vi "MC_8_7_12a_JW.vi"() -> ()   [LabVIEW 2011]
uses:
  <vilib>/Utility/file.llb/Read From Spreadsheet File (string).vi
  <vilib>/Utility/inputDevices.llb/keyboardAcquire.vi
  <vilib>/Utility/file.llb/Write To Spreadsheet File (DBL).vi
  <vilib>/Utility/file.llb/Write To Spreadsheet File (string).vi
  <vilib>/regexp/Match Regular Expression.xnode
panel:
  out "Opj X Axis":string
  in  "Room Temp":dbl=294.0
  out "No Image 2":path=path "\\\\acad1\\physics/Jurchescu-group/JW-PD/Image Not Found.png"
  out "Save1 Array":string[][](array[string])
  out "Lin Vd":dbl
  out "Lin-Vg Array-Used":dbl[](array[numeric])
  out "Lin Id-Used":dbl[](array[numeric])
  out "Comments":string
  out "Folder Index":dbl caption="Length"
  out "Current \nRecord":string[](array[string])
  out "Transformer \nHeaders":string[](array[string])
  out "Current Device ID":string
  out "Column":string
  out "Row":string
  out "Rec: Concentration":dbl
  out "Rec: Solvent":string
  out "Rec: Method":string
  in  "?":T1(tab)
  in  "Transport File":path
  out "Transport Folder":path
  out "Rec: Material":string
  in  "Treatment Concentration (mM):":dbl=nan
  in  "Surface Treatment:":string="NaN"
  in  "# Drops*:":dbl=inf
  in  "Solution Temp (C):":dbl=nan
  in  "Relative Humidity (%):":dbl=nan
  in  "Room Temp (F):":dbl=nan
  in  "Time (s):":dbl=nan
  out "Accel (RPM/s):":dbl
  in  "RPM:":dbl=nan
  in  "Wait Time (s):":dbl=nan
  in  "Sample #:":dbl=1.0
  in  "Fabricator:":string="NaN"
  in  "Transfer File":path
  out "Transfer Folder":path
  in  "Image Folder":path
  out "Image File":path=path "D:/UserData/Desktop/Jeremy/WFU/Research/Programs/VI mods/Image Not Found.png"
  in  "Ramp (s):":dbl=3.0
  out "Calc: On/Off":dbl caption="On/Off-Sat" format="%#.2e"
  out "Calc: Off I-Sat":dbl caption="Off I-Sat" format="%#.2e"
  in  "Manuel-Dielectric":bool
  in  "Manuel-Length":bool
  out "Calc: VT-Lin":dbl
  out "New: VT-Lin":dbl
  out "Rec: VT-Lin":dbl caption="VT-Lin" format="%#_3g"
  out "Calc: Trap Density-STS":dbl format="%#.2e"
  out "New: Trap Density-STS":dbl format="%#.2e"
  out "Rec: Trap Density-STS":dbl caption="N-Sat (STS)" format="%#.2e"
  out "Calc: Trap Density-VT":dbl format="%#.2e"
  out "New: Trap Density-VT":dbl format="%#.2e"
  out "Rec: Trap Density-VT":dbl caption="N-Sat (VT)" format="%#.2e"
  out "Calc: Mobility-Lin":dbl format="%#.2e"
  out "New: Mobility-Lin":dbl format="%#_4e"
  out "Rec: Mobility-Lin":dbl caption="Mobility-Lin" format="%#_3e"
  out "Calc: Mobility-Sat":dbl format="%#.2e"
  out "Rec: Length":dbl caption="Length" format="%#_3g"
  out "Rec: Width":dbl caption="Width" format="%#_4g"
  out "Rec: Dielectric (d)":dbl caption="Dielectric (d)" format="%#_3g"
  in  "Cancel Button":bool
  in  "Up Button":bool
  in  "Down Button":bool
  out "Data Name:":string
  in  "Save Changes?":bool
  in  "New: Dielectric":dbl
  in  "New: Length":dbl
  in  "New: Width":dbl
  out "New: Mobility-Sat":dbl format="%#.2e"
  in  "Blank Button":bool
  in  "Zoom":i16(slide)=-3 scale=-5.0..5.0
  out "Image Out 2":T2(plugin-control)
  out "Image Out":T2(plugin-control)
  in  "Magnification":u16(ring) items=["5x", "10x", "20x", "50x", "80x"]
  out "Total Width":dbl
  out "Distances":dbl[](array[numeric])
  in  "Undo Button":bool
  in  "Remove Button":bool
  out "Rec: Mobility-Sat":dbl caption="Mobility-Sat" format="%#.2e"
  out "Index":string
  out "Image Name":string
  in  "Export":bool
  out "Calc: VT-Sat":dbl format="%#.2g"
  out "New: VT-Sat":dbl format="%#.2g"
  in  "Manual-Width":bool caption="Manual"
  out "Calc: STS":dbl format="%#.2g"
  out "New: STS":dbl format="%#.2g"
  out "Rec: VT-Sat":dbl caption="VT-Sat" format="%#.2g"
  out "Rec: STS":dbl caption="STS-Sat" format="%#.2g"
  out "Rec: On/Off":dbl caption="On/Off-Sat" format="%#.2e"
  in  "Save Changes? 2":bool
  in  "Save Changes? 3":bool
  out "Date Recorded":string="Date Recorded" caption="Measured"
  out "Date Created":string caption="Fabricated"
  out "Rec: Temp":dbl caption="Sample Temp" format="%.1f"
  in  "New: Temp":dbl format="%.1f"
  out "Rec: Off I-Sat":dbl caption="Off I-Sat" format="%#.2e"
  in  "Independant Variable":string(combo)="Length (um):"
  in  "Transfer Plots":enum32{"Linear", "Saturation"}(tab)=enum."Saturation"
  out "XY Graph-Lin":cluster{dbl[], dbl[]}[](graph)
  in  "Slide":dbl(slide) step=1.0 scale=-22.0..89.0 scale format="%#_1p"
  out "XY Graph":cluster{dbl[], dbl[]}[](graph)
  in  "Previous Button":bool
  in  "Next Button":bool
  in  "NumPts":dbl=5.0
  in  "Log Plots":enum32{"Linear", "Saturation"}(tab)=enum."Saturation"
  in  "Slide 2":dbl(slide) step=1.0 scale=-1.0..82.0 scale format="%#_1p"
  out "XY Graph 2":cluster{dbl[], dbl[]}[](graph)
  in  "Previous Button 2":bool
  in  "Next Button 2":bool
  in  "NumPts 2":dbl=5.0 caption="NumPts"
  in  "Manual-Temp":bool caption="Manual"
  in  "Origin Project File":path=path "\\\\acad1\\physics/Jurchescu-group/JW-PD/Group Library/Origin Project Files/DeviceData_7_31_12b_JW.opj"
  in  "No Image File":path=path "\\\\acad1\\physics/Jurchescu-group/JW-PD/Mega Awesome/Image Not Found.png"
  out "String":string
  out "Index 2":dbl
  out "Sat Id-Log-Used":dbl[](array[numeric])
  out "Vg Array-Log-Used":dbl[](array[numeric])
  out "ROI Descriptor out":T3 {"Contours"."Type" items=["No Selection", "Point", "Line", "Rectangle", "Oval", "Polygon", "Freehand Region", "Annulus", "Unused2", "Unused3", "Broken Line", "Freehand Line", "Rotated Rectangle"]}
  out "ROI Descriptor":T3 {"Contours"."Type" items=["No Selection", "Point", "Line", "Rectangle", "Oval", "Polygon", "Freehand Region", "Annulus", "Unused2", "Unused3", "Broken Line", "Freehand Line", "Rotated Rectangle"]}
  out "Numeric 3":dbl
  out "Array 6":dbl[][](array[numeric])
  out "Cluster":T4
  out "Array 5":dbl[](array[numeric])
  out "Array 4":dbl[](array[numeric])
  out "Array 3":dbl[](array[numeric])
  out "Numeric 2":dbl
  out "Numeric":dbl
  out "Sat Id-Used":dbl[](array[numeric])
  out "Sat Vg Array-Used":dbl[](array[numeric])
  out "MobVi Index":dbl
  in  "Row Start":dbl=20.0
  # "Data Locations"
  # "Transport Location"
  # "Transfer Location"
  # "Image Location"
  # "Sample Properties"
  # "*     Inf = Full coverage\n   NaN = Unknown or Not Applicable"
  # "Recorded"
  # "Calculated"
  # "Re-Calculated"
  # "Manual"
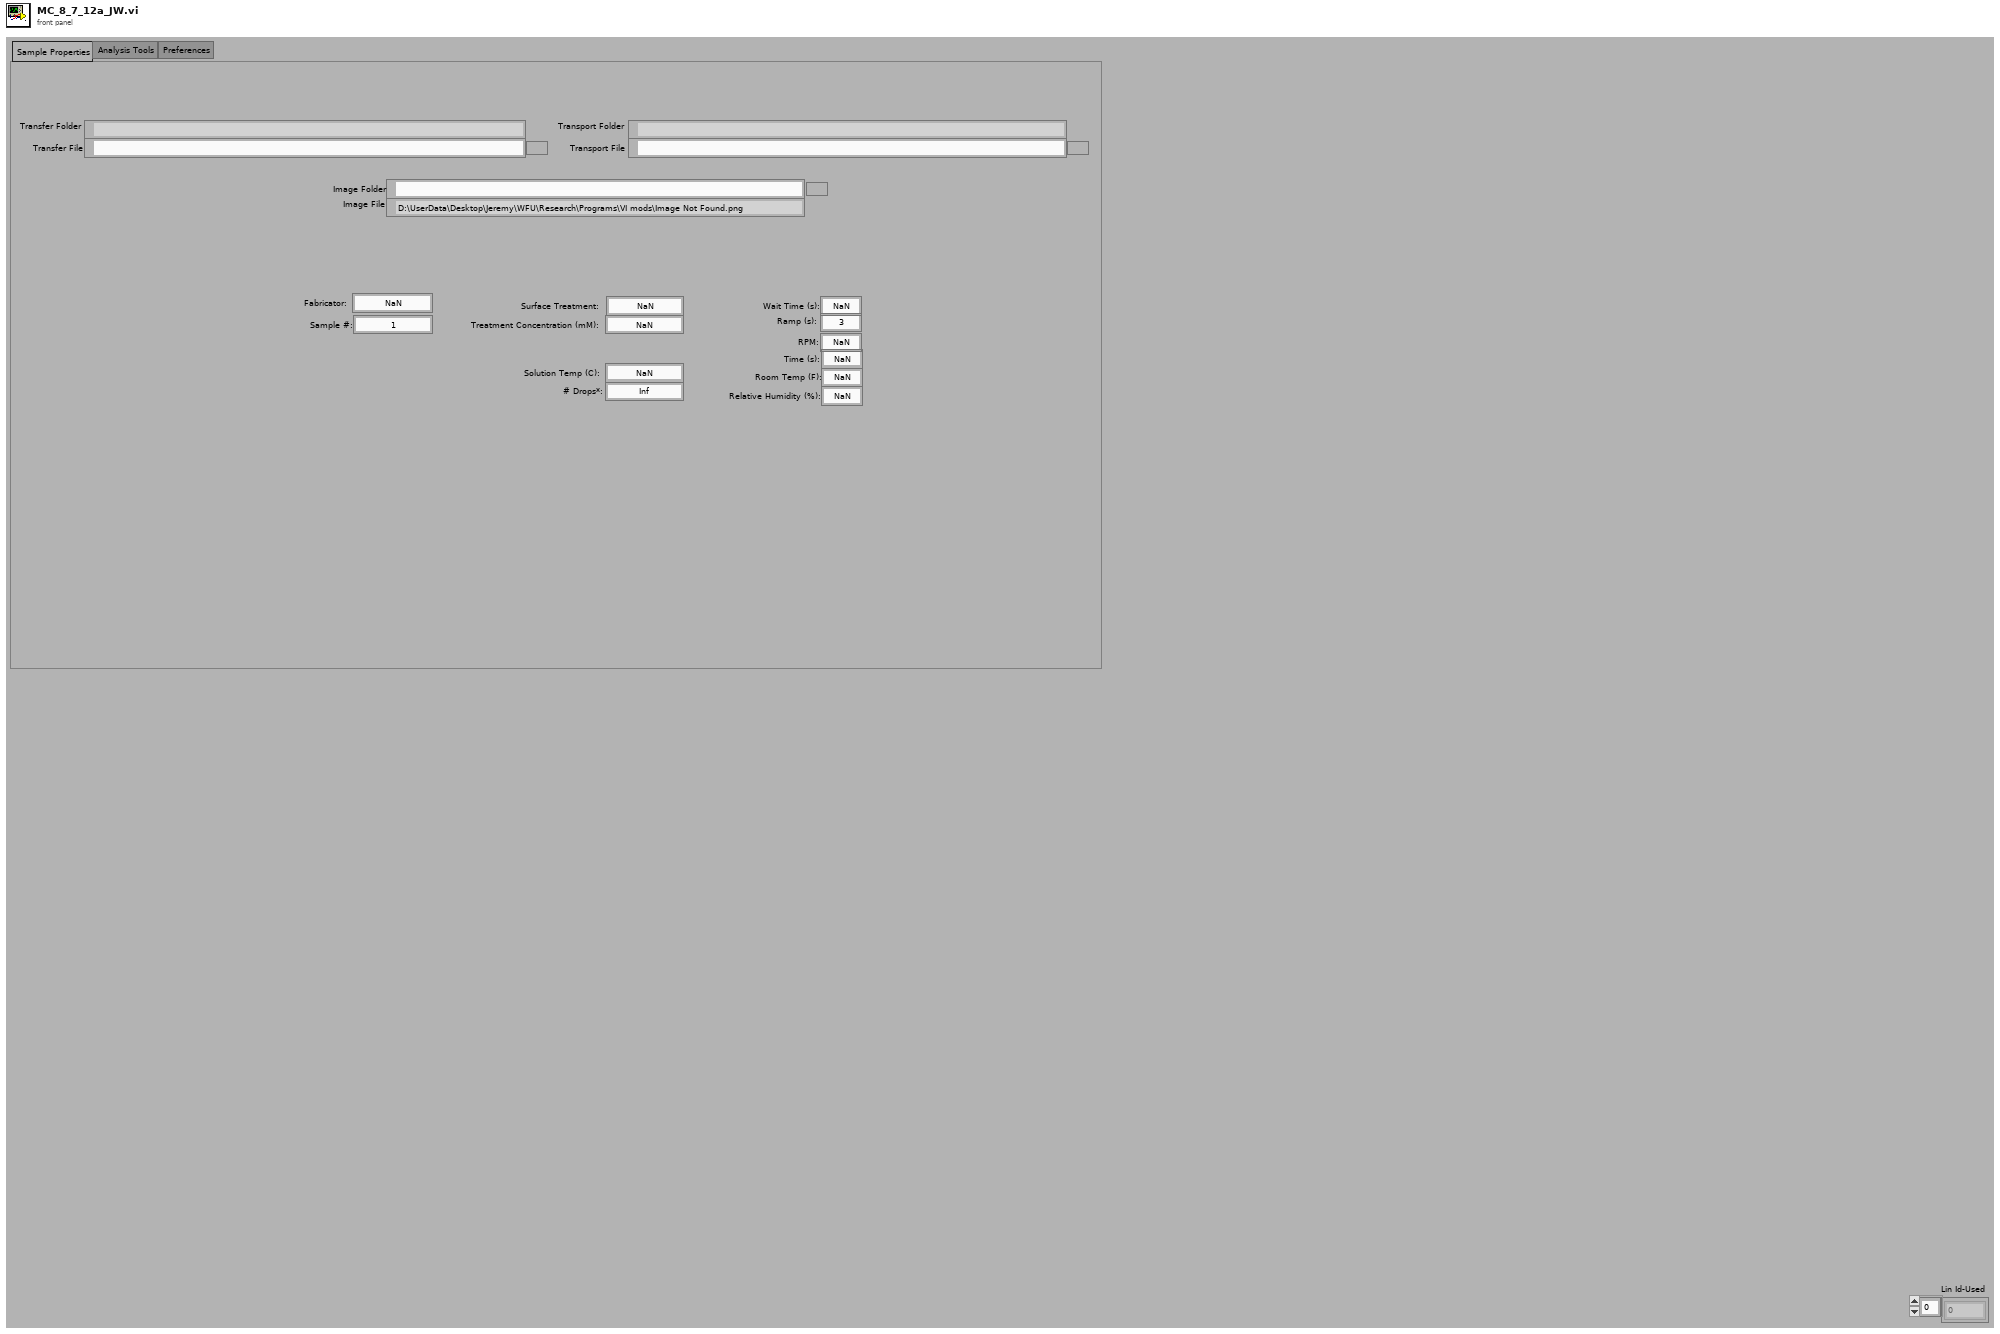
[diagram p1: front panel]
types:
  T1 = enum32{"Sample Properties", "Analysis Tools", "Preferences", "Current Database"}
  T2 = typedef "IMAQ Image.ctl" = refnum<image>
  T3 = typedef "ROI Descriptor" = cluster{"Global Rectangle":i32[], "Contours":cluster{"ID":enum32{"External", "Internal"}, "Type":u32, "Coordinates":i32[]}[]}
  T4 = cluster{"Numeric":dbl, "Numeric 2":dbl, "Numeric 3":dbl, "Numeric 4":dbl}
  T5 = cluster{"Mobility-Sat":dbl, "Moblitity-Lin":dbl, "On/Off":dbl, "Off Current":dbl, "Vt-Sat":dbl, "STS":dbl, "Trap Density-VT":dbl, "Trap Density-STS":dbl}
  T6 = cluster{"Date Recorded":string, "Index":string, "Length":dbl, "Width":dbl, "Sample Temp":dbl}
  T7 = cluster{"Date Created":string, "Material":string, "Solvent":string, "Concentration":dbl, "Method":string, "Dielectric (nm)":dbl, "Treatment":string, "Comments":string}
  T8 = cluster{"Mobility-Sat":dbl, "Vt-Sat":dbl, "Mobility-Lin":dbl, "Vt-Lin":dbl, "Off I-Sat":dbl, "On/Off I-Sat":dbl}
  T9 = cluster{"[0]":cluster{dbl[], dbl[]}, "[1]":cluster{dbl[], dbl[]}, "[2]":cluster{dbl[], dbl[]}, "[3]":cluster{dbl[], dbl[]}, "[4]":cluster{dbl[], dbl[]}, "[5]":cluster{dbl[], dbl[]}, "[6]":cluster{dbl[], dbl[]}, "[7]":cluster{dbl[], dbl[]}, "[8]":cluster{dbl[], dbl[]}}
  T10 = cluster{"Global Rectangle":i32[], "Contours":cluster{"Contour Type":u32, "ROI Type":u32, "Points":i32[]}[]}
  T11 = typedef "LVBoundsTypeDef.ctl" = cluster{"Width":u32, "Height":u32}
  T12 = enum16{"0", "1", "2", "3", "4", "5", "6", "7", "8", "9", "A", "B", "C", "D", "E", "F", "G", "H", "I", "J", "K", "L", "M", "N", "O", "P", "Q", "R", "S", "T", "U", "V", "W", "X", "Y", "Z", "F1", "F2", "F3", "F4", "F5", "F6", "F7", "F8", "F9", "F10", "F11", "F12", "F13", "F14", "F15", "ADD", "BACK", "BACKSLASH", "CAPITAL", "COMMA", "DECIMAL", "DELETE", "DIVIDE", "DOWN", "END", "EQUALS", "ESCAPE", "GRAVE (`)", "HOME", "INSERT", "LBRACKET", "LCONTROL", "LEFT", "L ALT", "LSHIFT", "LWIN", "MINUS", "MULTIPLY", "NEXT", "NUMLOCK", "NUMPAD_0", "NUMPAD_1", "NUMPAD_2", "NUMPAD_3", "NUMPAD_4", "NUMPAD_5", "NUMPAD_6", "NUMPAD_7", "NUMPAD_8", "NUMPAD_9", "PAUSE", "PERIOD", "PRIOR (PG UP)", "RBRACKET", "RCONTROL", "RETURN", "RIGHT", "R ALT", "RSHIFT", "RWIN", "SCROLL", "SEMICOLON", "SLASH", "SPACE", "SUBTRACT", "TAB", "UP", "ENTER (num pad)", "' (quote)"}[]
  T13 = enum16{"0", "1", "2", "3", "4", "5", "6", "7", "8", "9", "A", "B", "C", "D", "E", "F", "G", "H", "I", "J", "K", "L", "M", "N", "O", "P", "Q", "R", "S", "T", "U", "V", "W", "X", "Y", "Z", "F1", "F2", "F3", "F4", "F5", "F6", "F7", "F8", "F9", "F10", "F11", "F12", "F13", "F14", "F15", "ADD", "BACK", "BACKSLASH", "CAPITAL", "COMMA", "DECIMAL", "DELETE", "DIVIDE", "DOWN", "END", "EQUALS", "ESCAPE", "GRAVE (`)", "HOME", "INSERT", "LBRACKET", "LCONTROL", "LEFT", "L ALT", "LSHIFT", "LWIN", "MINUS", "MULTIPLY", "NEXT", "NUMLOCK", "NUMPAD_0", "NUMPAD_1", "NUMPAD_2", "NUMPAD_3", "NUMPAD_4", "NUMPAD_5", "NUMPAD_6", "NUMPAD_7", "NUMPAD_8", "NUMPAD_9", "PAUSE", "PERIOD", "PRIOR (PG UP)", "RBRACKET", "RCONTROL", "RETURN", "RIGHT", "R ALT", "RSHIFT", "RWIN", "SCROLL", "SEMICOLON", "SLASH", "SPACE", "SUBTRACT", "TAB", "UP", "ENTER (num pad)", "' (quote)"}
  T14 = cluster{"Contour Type":u32, "ROI Type":u32, "Points":i32[]}[]
  T15 = cluster{i32[], cluster{"Contour Type":u32, "ROI Type":u32, "Points":i32[]}[]}
  T16 = cluster{"Independant  Variable Indicator":string, "Parameter String Indicator":string}
  T17 = cluster{string, sgl, bool, bool, bool, bool, bool, bool, i32}
  T18 = cluster{i32, cluster{string, sgl, bool, bool, bool, bool, bool, bool, i32}, i32, i32}
  T19 = cluster{"Contour Type":u32, "ROI Type":u32, "Points":i32[]}
  T20 = cluster{"Points[0]":i32, "Points[1]":i32, "Points[2]":i32, "Points[3]":i32, "Points[4]":i32, "Points[5]":i32, "Points[6]":i32, "Points[7]":i32, "Points[8]":i32}
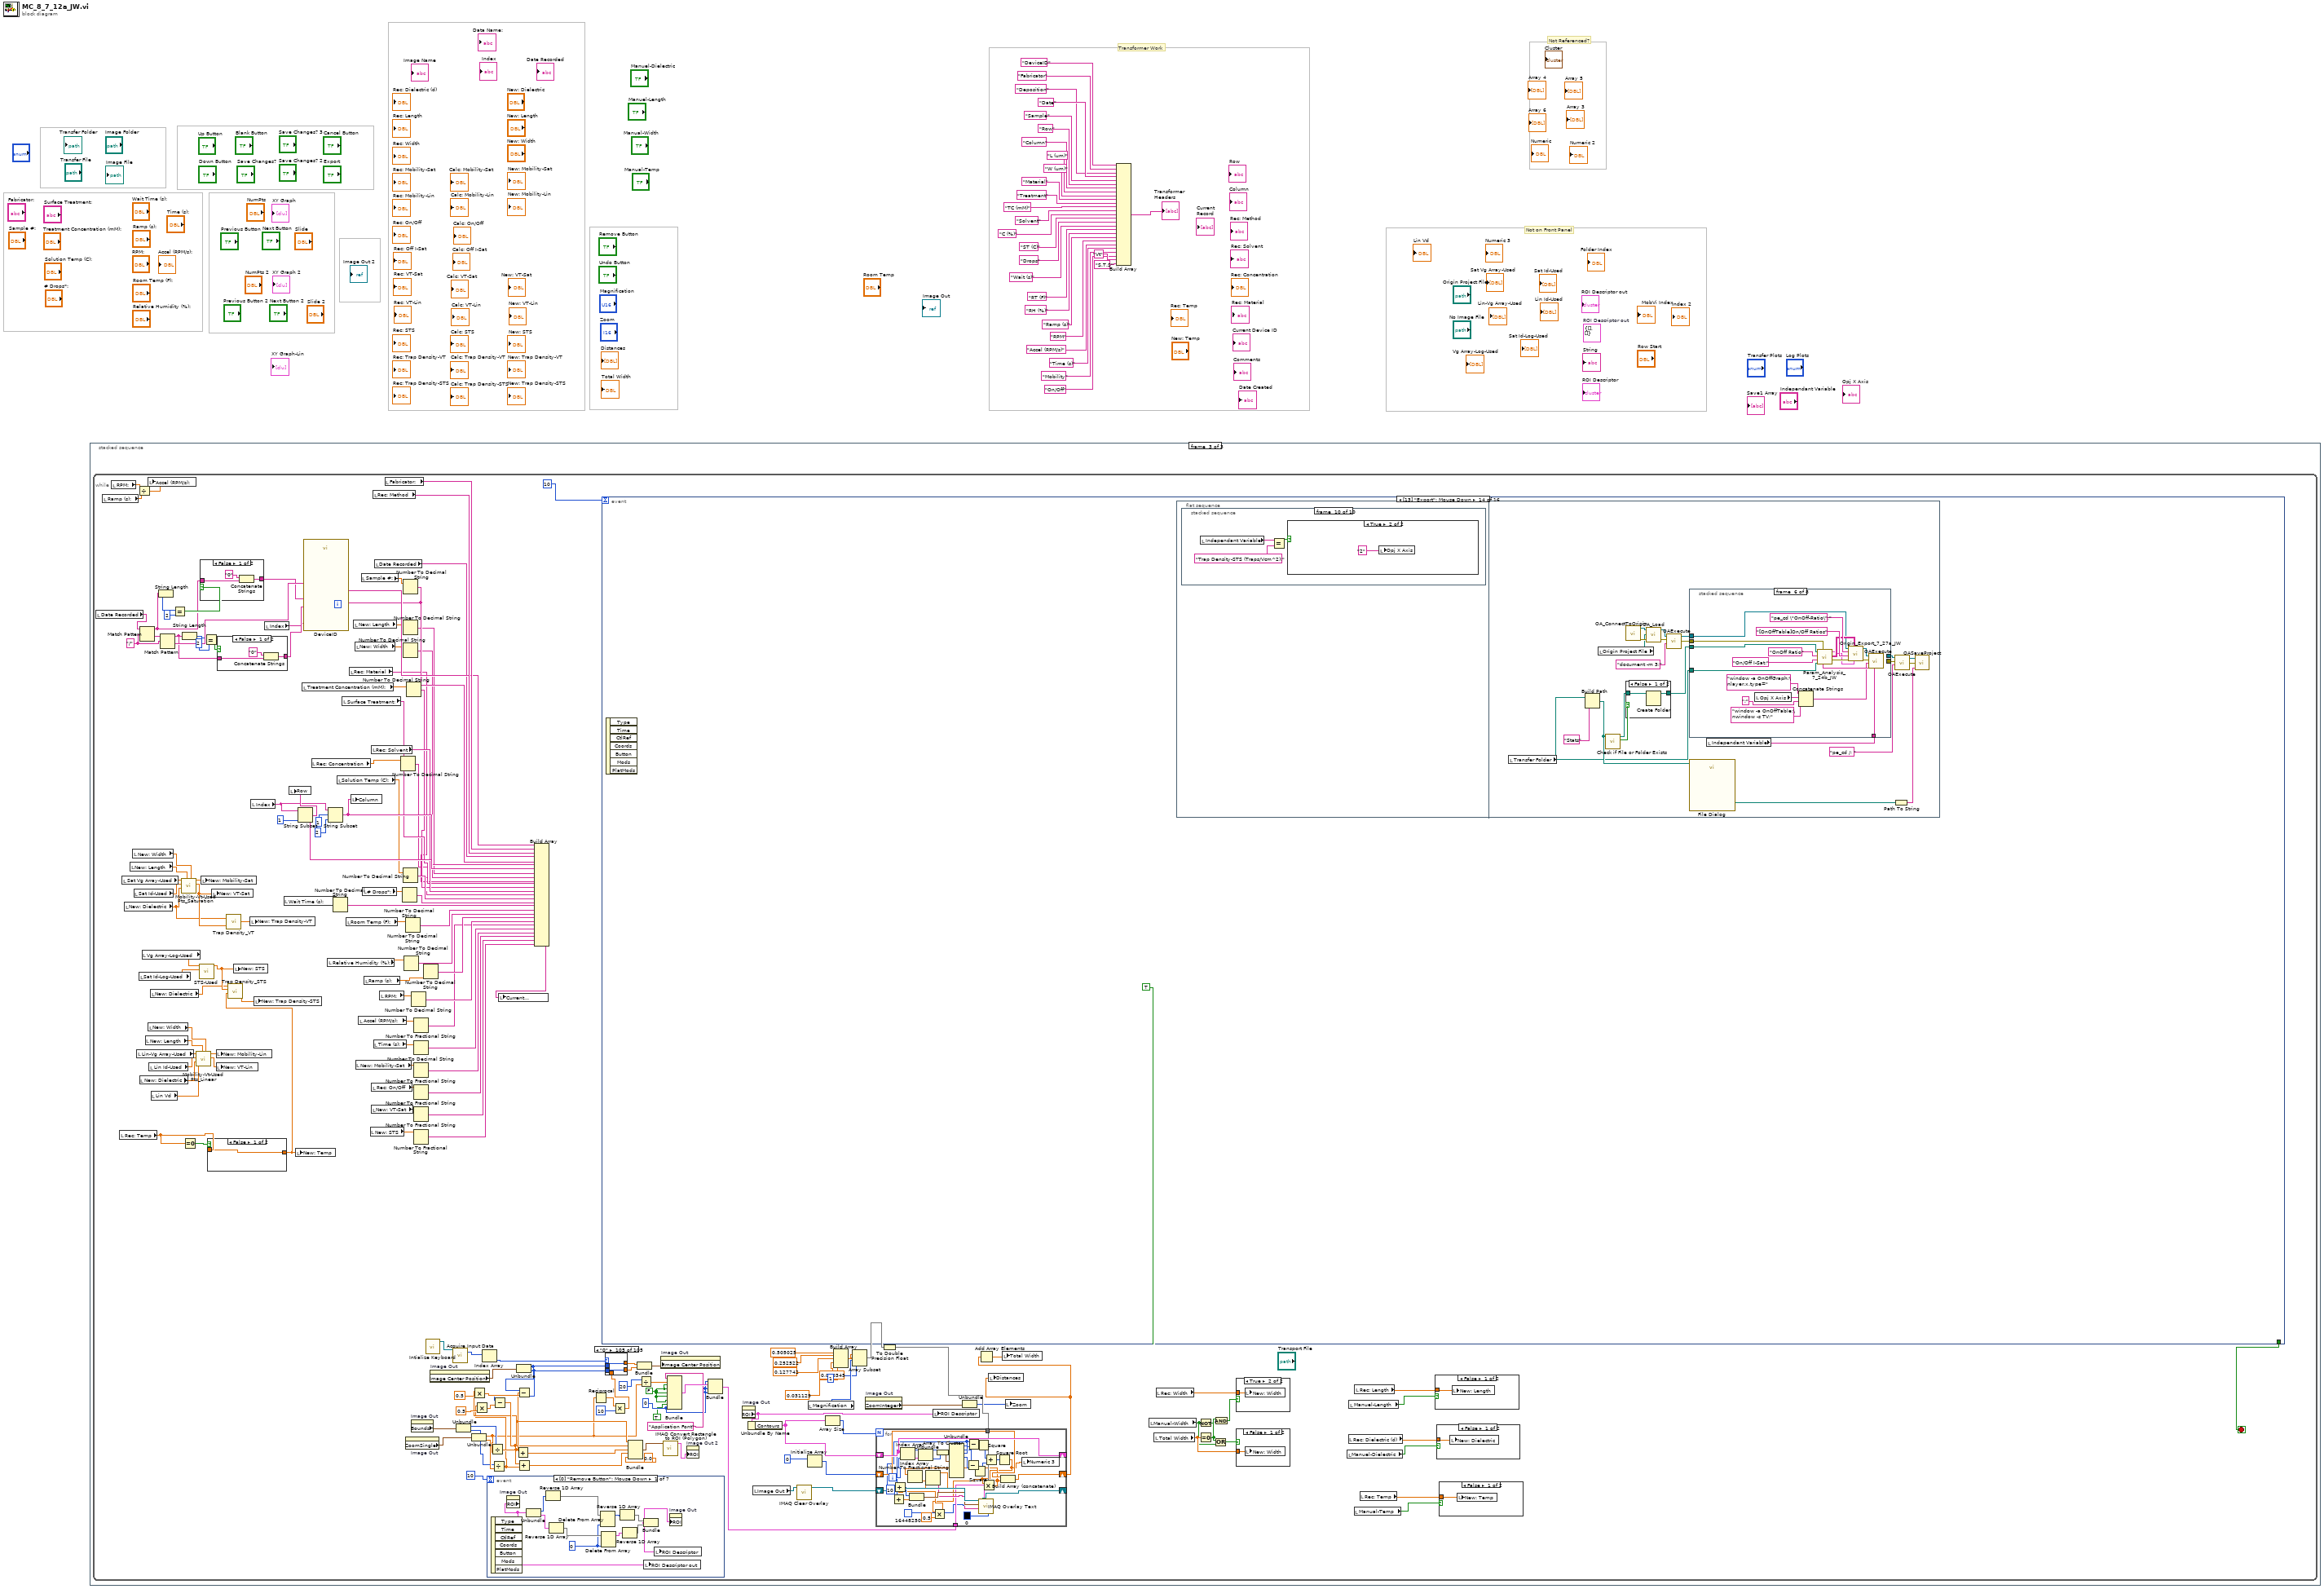
[diagram p0: block diagram]
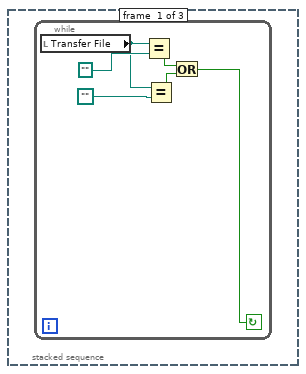
[diagram p2: hidden frame]
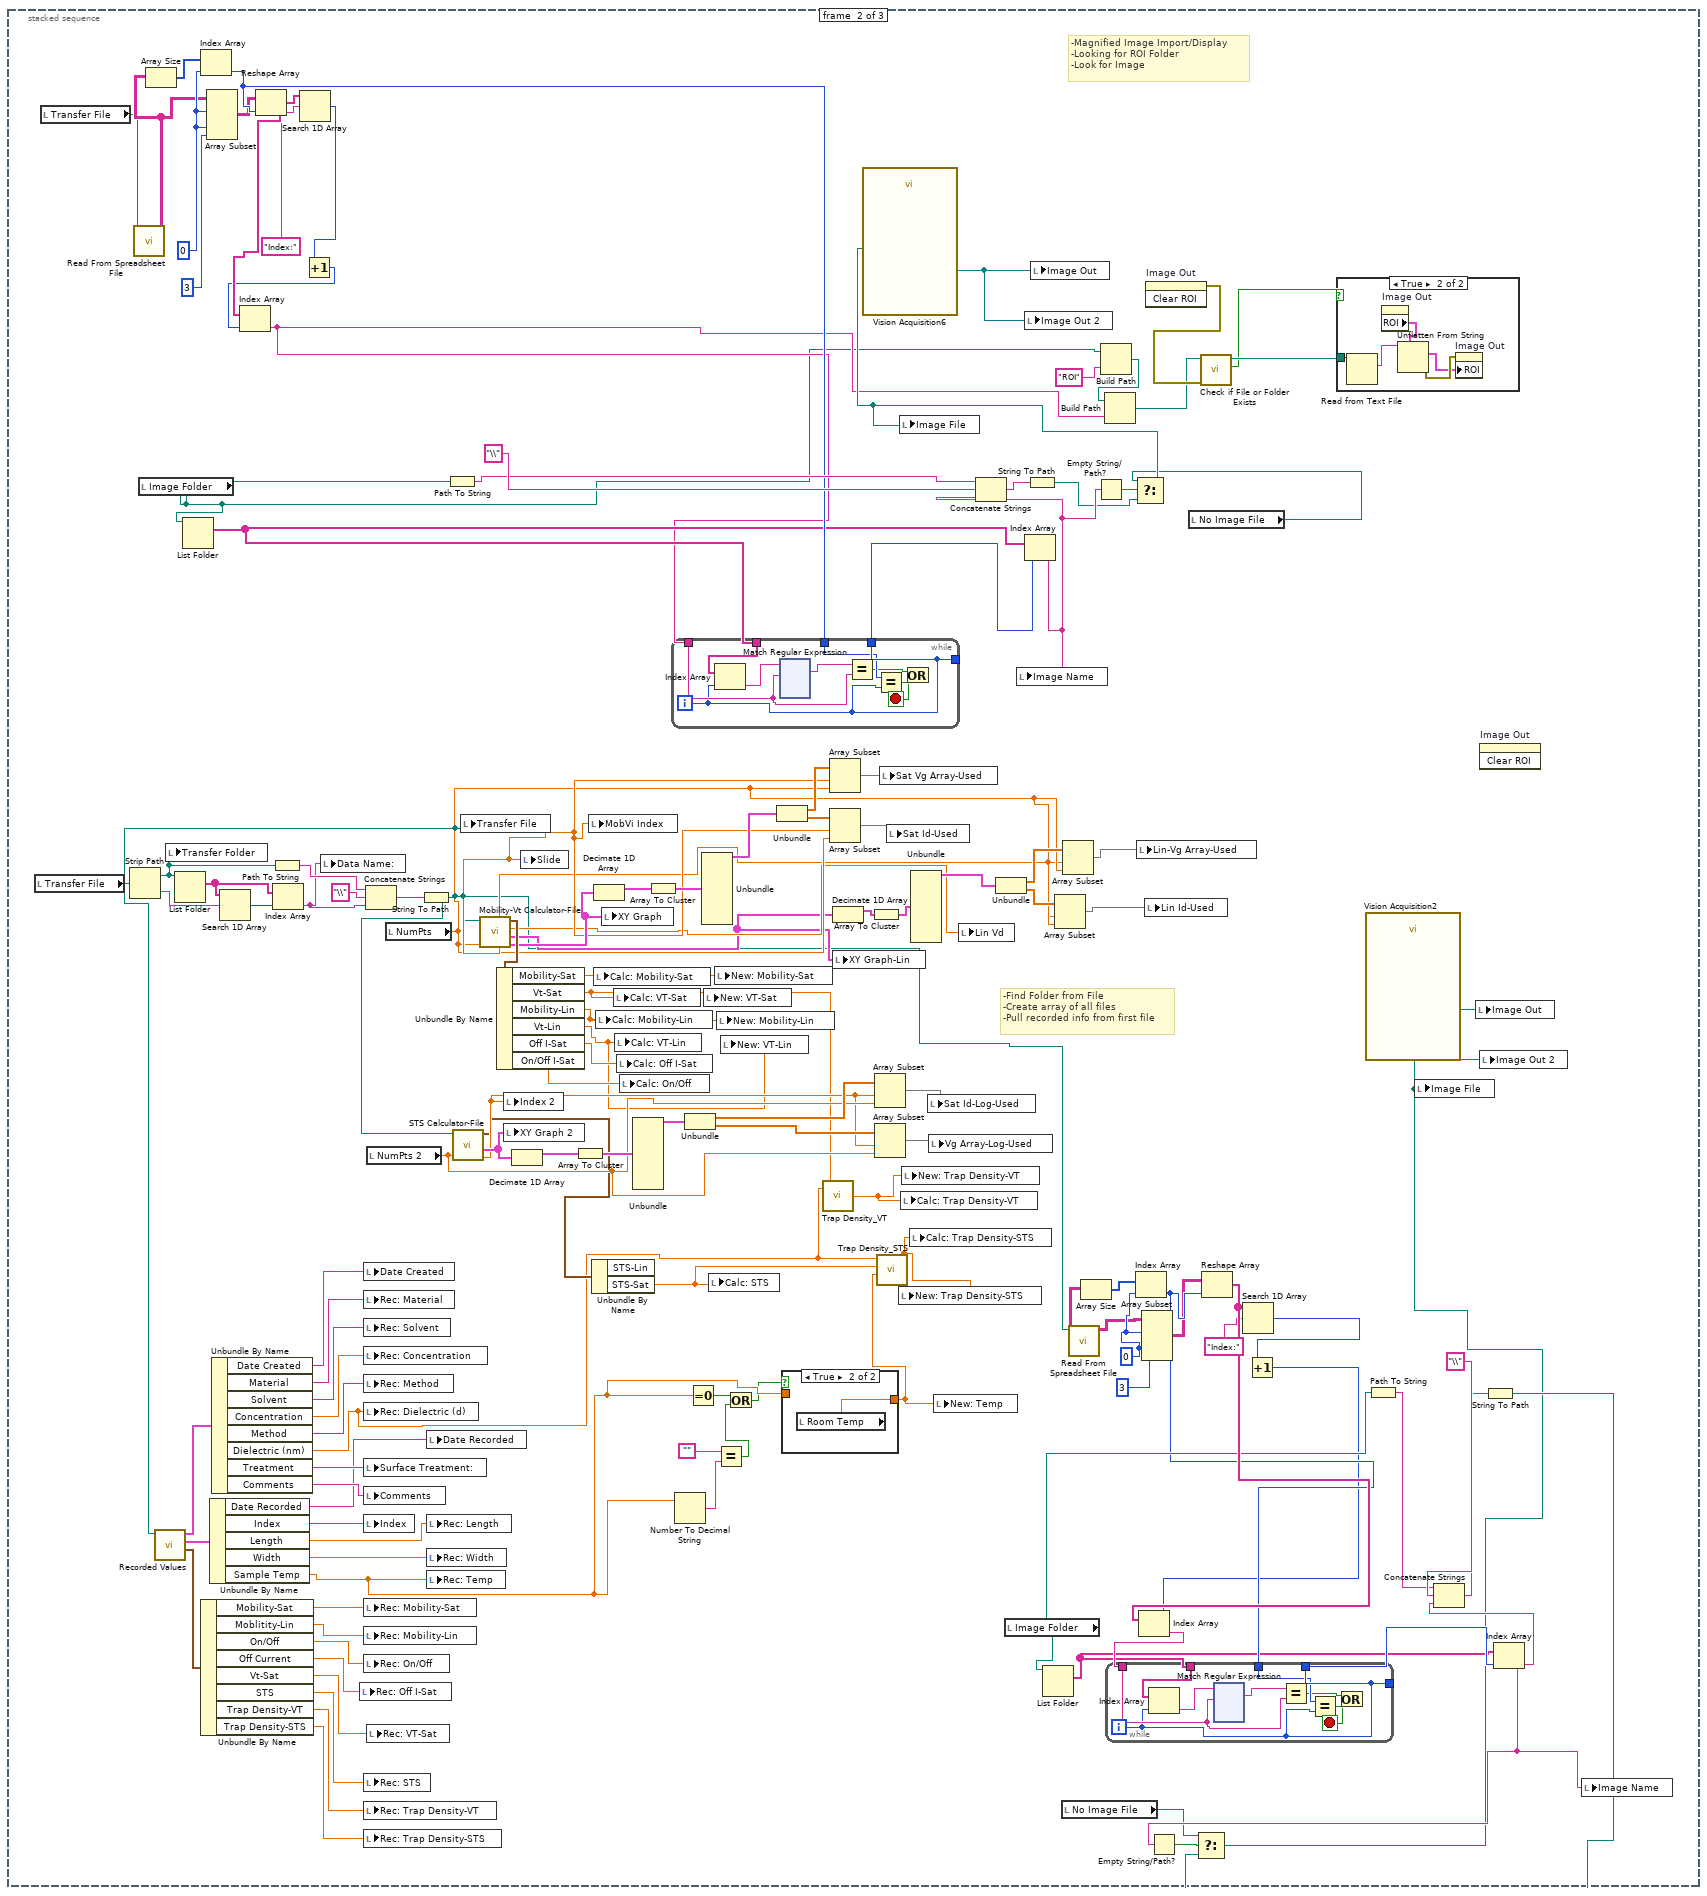
[diagram p3: hidden frame]
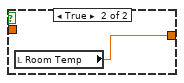
[diagram p7: hidden frame]
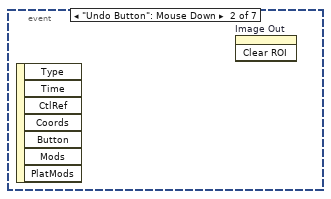
[diagram p14: hidden frame]
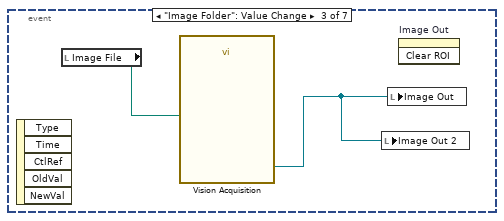
[diagram p15: hidden frame]
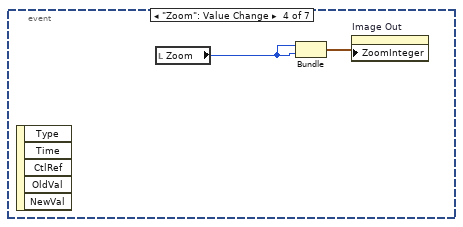
[diagram p16: hidden frame]
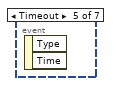
[diagram p17: hidden frame]
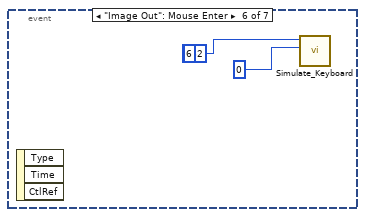
[diagram p18: hidden frame]
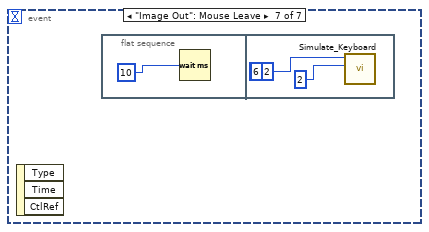
[diagram p19: hidden frame]
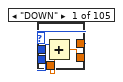
[diagram p20: hidden frame]
diagram:
  (unwired) T3 {"Global Rectangle"=[], "Contours"=[]}  # ROI Descriptor out
  # "Not Referenced?"
  # "Transformer Work"
  # "Not on Front Panel"
  n1 = stacked-sequence {
    frame #0 {
      n2 = while {
        stop <- w29 continue-if-true
        n3 = local read "Transfer File"() -> (w31:path)
        n4 = Equal?(x=w31, y=path "") -> (x = y?=w33:bool)
        n5 = Equal?(x=w31, y=path "") -> (x = y?=w32:bool)
        n6 = Or(x=w33, y=w32) -> (x .or. y?=w29:bool)
      }
    }
    frame #1 {
      w133 = 0
      w157 = 0
      # "-Find Folder from File\n-Create array of all files\n-Pull recorded info from first file"
      # "-Magnified Image Import/Display\n-Looking for ROI Folder\n-Look for Image"
      n7 = local read "Transfer File"() -> (w137:path)
      n8 = local read "Transfer File"() -> (w152:path)
      n9 = Strip Path(path=w137) -> (stripped path=w138:path, name=w124:string)
      n10 = call-poly <vilib>:"Read From Spreadsheet File.vi"("file path (dialog if empty)"=w152) -> ("all rows"=w155:string[][])  [unwired: 6 in, 4 out]
      n11 = local read "Image Folder"() -> (w94:path)
      n12 = Array Size(array=w155) -> (size(s)=w156:i32[])
      n13 = local write "Transfer Folder"(w138) -> ()
      n14 = List Folder(path=w138) -> (filenames=w128:string[])  [unwired: 3 in, 3 out]
      n15 = List Folder(path=w94) -> (filenames=w161:string[])  [unwired: 3 in, 3 out]
      n16 = Index Array(array=w156, index=w157) -> (element=w163:i32)
      n17 = Array Subset(array=w155, index (row)=w157, index (col)=w157, length (col)=3) -> (w154:string[][])  [unwired: 1 in]
      n18 = Search 1D Array(1D array=w128, element=w124) -> (index of element=w127:i32)  [unwired: 1 in]
      n19 = Reshape Array(w154, w163) -> (w168:string[])
      n20 = Path To String(path=w138) -> (string=w123:string)
      n21 = Index Array(array=w128, index=w127) -> (element=w93:string)
      n22 = Search 1D Array(1D array=w168, element="Index:") -> (index of element=w160:i32)  [unwired: 1 in]
      n23 = Increment(x=w160) -> (x+1=w159:i32)
      n24 = Index Array(array=w168, index=w159) -> (element=w95:string)
      n25 = local write "Data Name:"(w93) -> ()
      n26 = Concatenate Strings(w123, "\\", w93) -> (w125:string)
      n27 = local read "NumPts 2"() -> (w68:dbl)
      n28 = local read "NumPts"() -> (w59:dbl)
      n29 = String To Path(string=w125) -> (path=w52:path)
      n30 = call "Recorded Values.vi"("Path"=w52) -> ("Recorded Char"=w91:T5, "Recorded Prop"=w90:T6, "Fabrication Prop"=w92:T7)  [unwired: 8 in]
      n31 = Unbundle By Name(w91) -> ("Mobility-Sat"=w79:dbl, "Moblitity-Lin"=w78:dbl, "On/Off"=w77:dbl, "Off Current"=w76:dbl, "Vt-Sat"=w38:dbl, "STS"=w75:dbl, "Trap Density-VT"=w74:dbl, "Trap Density-STS"=w73:dbl)
      n32 = Unbundle By Name(w90) -> ("Date Recorded"=w83:string, "Index"=w82:string, "Length"=w81:dbl, "Width"=w80:dbl, "Sample Temp"=w44:dbl)
      n33 = Unbundle By Name(w92) -> ("Date Created"=w72:string, "Material"=w89:string, "Solvent"=w88:string, "Concentration"=w87:dbl, "Method"=w86:string, "Dielectric (nm)"=w48:dbl, "Treatment"=w85:string, "Comments"=w84:string)
      n34 = local write "Rec: Off I-Sat"(w76) -> ()
      n35 = local write "Date Created"(w72) -> ()
      n36 = local write "Rec: Material"(w89) -> ()
      n37 = local write "Rec: Solvent"(w88) -> ()
      n38 = local write "Rec: Concentration"(w87) -> ()
      n39 = local write "Rec: Method"(w86) -> ()
      n40 = local write "Rec: Dielectric (d)"(w48) -> ()
      n41 = local write "Surface Treatment:"(w85) -> ()
      n42 = local write "Comments"(w84) -> ()
      n43 = local write "Index"(w82) -> ()
      n44 = local write "Rec: Mobility-Sat"(w79) -> ()
      n45 = local write "Rec: Mobility-Lin"(w78) -> ()
      n46 = local write "Rec: On/Off"(w77) -> ()
      n47 = local write "Rec: STS"(w75) -> ()
      n48 = local write "Rec: Trap Density-VT"(w74) -> ()
      n49 = local write "Rec: Trap Density-STS"(w73) -> ()
      n50 = local write "Rec: VT-Sat"(w38) -> ()
      n51 = local write "Date Recorded"(w83) -> ()
      n52 = local write "Rec: Length"(w81) -> ()
      n53 = local write "Rec: Width"(w80) -> ()
      n54 = local write "Rec: Temp"(w44) -> ()
      n55 = Path To String(path=w94) -> (string=w165:string)
      n56 = call "STS Calculator-File.vi"("NumPts"=w68, "Path"=w52) -> ("STS Index-Sat"=w66:dbl, "XY Graph-Sat"=w67:cluster{dbl[], dbl[]}[], "Ouput"=w65:cluster{"STS-Sat":dbl, "STS-Lin":dbl})  [unwired: 5 in, 2 out]
      n57 = local write "Transfer File"(w52) -> ()
      n58 = call "Mobility-Vt Calculator-File.vi"("NumPts"=w59, "Path"=w52) -> ("XY Graph-Sat"=w70:cluster{dbl[], dbl[]}[], "XY Graph-Lin"=w54:cluster{dbl[], dbl[]}[], "Lin Vd"=w55:dbl, "Output"=w71:T8, "Index-Sat"=w69:dbl, "Index-Lin"=w58:dbl)  [unwired: 4 in]
      n59 = Unbundle By Name(w71) -> ("Mobility-Sat"=w47:dbl, "Vt-Sat"=w46:dbl, "Mobility-Lin"=w37:dbl, "Vt-Lin"=w35:dbl, "Off I-Sat"=w53:dbl, "On/Off I-Sat"=w36:dbl)
      n60 = local write "Index 2"(w66) -> ()
      n61 = local write "XY Graph 2"(w67) -> ()
      n62 = Decimate 1D Array(w67) -> (w115:cluster{dbl[], dbl[]}[])  [unwired: 1 out]
      n63 = local write "Slide"(w69) -> ()
      n64 = Array To Cluster(array=w115) -> (cluster=w117:T9)
      n65 = local write "MobVi Index"(w69) -> ()
      n66 = Unbundle By Name(w65) -> ("STS-Sat"=w51:dbl)  [unwired: 1 out]
      n67 = Decimate 1D Array(w70) -> (w151:cluster{dbl[], dbl[]}[])  [unwired: 1 out]
      n68 = local write "Calc: Mobility-Sat"(w47) -> ()
      n69 = local write "Calc: Mobility-Lin"(w37) -> ()
      n70 = local write "XY Graph"(w70) -> ()
      n71 = local write "Calc: VT-Sat"(w46) -> ()
      n72 = local write "Calc: VT-Lin"(w35) -> ()
      n73 = local write "Calc: Off I-Sat"(w53) -> ()
      n74 = local write "Calc: On/Off"(w36) -> ()
      n75 = Unbundle(w117) -> ("[0]"=w116:cluster{dbl[], dbl[]})  [unwired: 8 out]
      n76 = Array To Cluster(array=w151) -> (cluster=w149:T9)
      n77 = while {
        tunnel: w161 -> [w303]
        tunnel: w95 -> [w301]
        tunnel: [w300] -> _
        tunnel: [w300] -> w162
        tunnel: w163 -> [w299]
        i -> [w300]
        stop <- w296 stop-if-true
        n78 = Index Array(array=w303, index=w300) -> (element=w304:string)
        n79 = xnode "Match Regular Expression"("input string"=w304, "regular expression"=w301) -> ("whole match"=w302:string)  [unwired: 4 in, 4 out]
        n80 = Equal?(x=w302, y=w301) -> (x = y?=w298:bool)
        n81 = Equal?(x=w299, y=w300) -> (x = y?=w297:bool)
        n82 = Or(x=w298, y=w297) -> (x .or. y?=w296:bool)
      }
      n83 = Number To Decimal String(number=w44) -> (decimal integer string=w42:string)  [unwired: 1 in]
      n84 = Unbundle(w116) -> (w113:dbl[], w112:dbl[])
      n85 = Equal To 0?(x=w44) -> (x = 0?=w43:bool)
      n86 = Unbundle(w149) -> ("[0]"=w150:cluster{dbl[], dbl[]})  [unwired: 8 out]
      n87 = local write "New: VT-Sat"(w46) -> ()
      n88 = local write "Calc: STS"(w51) -> ()
      n89 = local write "New: Mobility-Sat"(w47) -> ()
      n90 = Equal?(x="", y=w42) -> (x = y?=w40:bool)
      n91 = local write "New: Mobility-Lin"(w37) -> ()
      n92 = local write "New: VT-Lin"(w35) -> ()
      n93 = Or(x=w43, y=w40) -> (x .or. y?=w39:bool)
      n94 = Unbundle(w150) -> (w114:dbl[], w118:dbl[])
      n95 = case shown="True" w39 {
        tunnel: [w169 w170] -> w50
        tunnel: w44 -> [w169 _]
        frame False {
        }
        frame True {
          n96 = local read "Room Temp"() -> (w170:dbl)
        }
      }
      n97 = call "Trap Density_VT.vi"("VT"=w46, "Dielectric"=w48) -> ("Trap Density-VT"=w45:dbl)
      n98 = Array Subset(array=w114, index=w69, length=w59) -> (w121:dbl[])
      n99 = Array Subset(array=w118, index=w69, length=w59) -> (w122:dbl[])
      n100 = Decimate 1D Array(w54) -> (w64:cluster{dbl[], dbl[]}[])  [unwired: 1 out]
      n101 = local write "XY Graph-Lin"(w54) -> ()
      n102 = Array To Cluster(array=w64) -> (cluster=w63:T9)
      n103 = Array Subset(array=w113, index=w66, length=w68) -> (w120:dbl[])
      n104 = Array Subset(array=w112, index=w66, length=w68) -> (w119:dbl[])
      n105 = call "Trap Density_STS.vi"("Temp (T) [K]"=w50, "S.T.S. (S)"=w51, "Dielectric"=w48) -> ("Trap Density (N)"=w49:dbl)  [unwired: 8 in]
      n106 = local write "Sat Vg Array-Used"(w121) -> ()
      n107 = local write "Sat Id-Used"(w122) -> ()
      n108 = local write "New: Trap Density-STS"(w49) -> ()
      n109 = local write "Calc: Trap Density-VT"(w45) -> ()
      n110 = local write "New: Trap Density-VT"(w45) -> ()
      n111 = local write "Calc: Trap Density-STS"(w49) -> ()
      n112 = Unbundle(w63) -> ("[0]"=w62:cluster{dbl[], dbl[]})  [unwired: 8 out]
      n113 = local write "Sat Id-Log-Used"(w120) -> ()
      n114 = local write "Vg Array-Log-Used"(w119) -> ()
      n115 = local write "New: Temp"(w50) -> ()
      n116 = local write "Lin Vd"(w55) -> ()
      n117 = Unbundle(w62) -> (w61:dbl[], w60:dbl[])
      n118 = local read "Image Folder"() -> (w144:path)
      n119 = Index Array(array=w161, index=w162) -> (element=w111:string)
      n120 = Concatenate Strings(w165, "\\", w111) -> (w166:string)
      n121 = local write "Image Name"(w111) -> ()
      n122 = String To Path(string=w166) -> (path=w109:path)
      n123 = List Folder(path=w144) -> (filenames=w140:string[])  [unwired: 3 in, 3 out]
      n124 = Array Subset(array=w60, index=w58, length=w59) -> (w56:dbl[])
      n125 = local read "No Image File"() -> (w103:path)
      n126 = Array Subset(array=w61, index=w58, length=w59) -> (w57:dbl[])
      n127 = call-poly <vilib>:"Read From Spreadsheet File.vi"("file path (dialog if empty)"=w52) -> ("all rows"=w131:string[][])  [unwired: 6 in, 4 out]
      n128 = Array Size(array=w131) -> (size(s)=w132:i32[])
      n129 = Empty String/Path?(string/path=w111) -> (empty?=w110:bool)
      n130 = Build Path(base path=w94, name or relative path="ROI") -> (appended path=w97:path)
      n131 = Build Path(base path=w97, name or relative path=w95) -> (appended path=w96:path)
      n132 = Index Array(array=w132, index=w133) -> (element=w143:i32)
      n133 = local write "Lin-Vg Array-Used"(w57) -> ()
      n134 = Array Subset(array=w131, index (row)=w133, index (col)=w133, length (col)=3) -> (w130:string[][])  [unwired: 1 in]
      n135 = local write "Lin Id-Used"(w56) -> ()
      n136 = invoke on="Image Out" class="ImageControl" method="Clear ROI"() -> (error out=w101:errorcluster)  [unwired: 3 in, 2 out]
      n137 = local read "No Image File"() -> (w102:path)
      n138 = Select(t=w102, s=w110, f=w109) -> (s? t:f=w108:path)
      n139 = call "Vision Acquisition6"("Image Path"=w108) -> ("Image Out"=w164:T2)  [unwired: 25 in, 1 out]
      n140 = local write "Image File"(w108) -> ()
      n141 = local write "Image Out 2"(w164) -> ()
      n142 = local write "Image Out"(w164) -> ()
      n143 = call <vilib>:"Check if File or Folder Exists.vi"("error in (no error)"=w101, "path"=w96) -> ("file or folder exists?"=w99:bool, "dup path"=w100:path)  [unwired: 7 in, 1 out]
      n144 = Reshape Array(w130, w143) -> (w148:string[])
      n145 = Search 1D Array(1D array=w148, element="Index:") -> (index of element=w136:i32)  [unwired: 1 in]
      n146 = Increment(x=w136) -> (x+1=w135:i32)
      n147 = Index Array(array=w148, index=w135) -> (element=w141:string)
      n148 = while {
        tunnel: w140 -> [w183]
        tunnel: w141 -> [w181]
        tunnel: [w180] -> _
        tunnel: [w180] -> w142
        tunnel: w143 -> [w179]
        i -> [w180]
        stop <- w176 stop-if-true
        n149 = Index Array(array=w183, index=w180) -> (element=w184:string)
        n150 = xnode "Match Regular Expression"("input string"=w184, "regular expression"=w181) -> ("whole match"=w182:string)  [unwired: 4 in, 4 out]
        n151 = Equal?(x=w182, y=w181) -> (x = y?=w178:bool)
        n152 = Equal?(x=w179, y=w180) -> (x = y?=w177:bool)
        n153 = Or(x=w178, y=w177) -> (x .or. y?=w176:bool)
      }
      n154 = case shown="True" w99 {
        tunnel: w100 -> [_ w171]
        frame False {
        }
        frame True {
          n155 = Read from Text File(file (use dialog)=w171) -> (text=w175:string)  [unwired: 3 in, 3 out]
          n156 = property on="Image Out" class="ImageControl"() -> ("ROI"=w172:T10)  [unwired: 2 in, 2 out]
          n157 = Unflatten From String(type=w172, binary string=w175) -> (value=w173:T10, error out=w174:errorcluster)  [unwired: 3 in, 1 out]
          n158 = property on="Image Out" class="ImageControl"(error in=w174, "ROI"=w173) -> ()  [unwired: 1 in, 2 out]
        }
      }
      n159 = Path To String(path=w144) -> (string=w145:string)
      n160 = invoke on="Image Out" class="ImageControl" method="Clear ROI"() -> ()  [unwired: 3 in, 3 out]
      n161 = Index Array(array=w140, index=w142) -> (element=w106:string)
      n162 = Empty String/Path?(string/path=w106) -> (empty?=w107:bool)
      n163 = Concatenate Strings(w145, "\\", w106) -> (w146:string)
      n164 = String To Path(string=w146) -> (path=w105:path)
      n165 = Select(t=w103, s=w107, f=w105) -> (s? t:f=w104:path)
      n166 = call "Vision Acquisition2"("Image Path"=w104) -> ("Image Out"=w139:T2)  [unwired: 25 in, 1 out]
      n167 = local write "Image File"(w104) -> ()
      n168 = local write "Image Out"(w139) -> ()
      n169 = local write "Image Out 2"(w139) -> ()
      n170 = local write "Image Name"(w106) -> ()
    }
    frame #2 {
      n171 = while {
        stop <- w583 stop-if-true
        w479 = "/"
        w533 = FALSE
        w531 = 0
        n172 = local read "Date Recorded"() -> (w482:string)
        n173 = local read "Ramp (s):"() -> (w449:dbl)
        n174 = local read "RPM:"() -> (w450:dbl)
        n175 = local read "Rec: Temp"() -> (w421:dbl)
        n176 = local read "Sat Vg Array-Used"() -> (w438:dbl[])
        n177 = local read "New: Dielectric"() -> (w423:dbl)
        n178 = local read "New: Length"() -> (w439:dbl)
        n179 = local read "New: Width"() -> (w441:dbl)
        n180 = local read "Sat Id-Used"() -> (w437:dbl[])
        n181 = local read "Lin-Vg Array-Used"() -> (w432:dbl[])
        n182 = Divide(x=w450, y=w449) -> (x/y=w448:dbl)
        n183 = local read "Sat Id-Log-Used"() -> (w436:dbl[])
        n184 = local read "New: Dielectric"() -> (w429:dbl)
        n185 = Match Pattern(string=w482, regular expression=w479) -> (before substring=w473:string, after substring=w480:string)  [unwired: 1 in, 2 out]
        n186 = local read "Vg Array-Log-Used"() -> (w435:dbl[])
        n187 = local read "New: Length"() -> (w431:dbl)
        n188 = local write "Accel (RPM/s):"(w448) -> ()
        n189 = local read "New: Width"() -> (w428:dbl)
        n190 = local read "Lin Id-Used"() -> (w433:dbl[])
        n191 = local read "New: Dielectric"() -> (w425:dbl)
        n192 = local read "Lin Vd"() -> (w427:dbl)
        n193 = String Length(string=w473) -> (length=w476:i32)
        n194 = Match Pattern(string=w480, regular expression=w479) -> (before substring=w467:string, after substring=w478:string)  [unwired: 1 in, 2 out]
        n195 = Equal?(x=w476, y=2) -> (x = y?=w474:bool)
        n196 = call "Mobility-Vt-Used Pts_Saturation.vi"("Width"=w441, "Length"=w439, "Dielectric (d)"=w423, "Sat Id Used"=w437, "Vg Used"=w438) -> ("Vt"=w424:dbl, "Mobility"=w440:dbl)  [unwired: 4 in, 1 out]
        n197 = String Length(string=w467) -> (length=w469:i32)
        n198 = Equal To 0?(x=w421) -> (x = 0?=w420:bool)
        n199 = call "Mobility-Vt-Used Pts_Linear.vi"("Width"=w428, "Length"=w431, "Vd"=w427, "Dielectric (d)"=w429, "Sat Id Used"=w433, "Vg Used"=w432) -> ("Vt"=w434:dbl, "Mobility"=w430:dbl)  [unwired: 3 in, 1 out]
        n200 = call "STS-Used.vi"("Id Used"=w436, "Vg-Used"=w435) -> ("STS"=w426:dbl)  [unwired: 9 in]
        n201 = case shown="False" w474 {
          tunnel: w473 -> [w594 w596]
          tunnel: [w593 w596] -> w472
          frame False {
            n202 = Concatenate Strings("0", w594) -> (w593:string)
          }
          frame True {
          }
        }
        n203 = local write "New: Mobility-Sat"(w440) -> ()
        n204 = Equal?(x=w469, y=2) -> (x = y?=w471:bool)
        n205 = case shown="False" w420 {
          tunnel: [w585 w586] -> w418
          tunnel: w421 -> [w585 _]
          frame False {
          }
          frame True {
            n206 = local read "Room Temp"() -> (w586:dbl)
          }
        }
        n207 = local write "New: VT-Sat"(w424) -> ()
        n208 = local write "New: Mobility-Lin"(w430) -> ()
        n209 = local write "New: VT-Lin"(w434) -> ()
        n210 = case shown="False" w471 {
          tunnel: w467 -> [w590 w592]
          tunnel: [w589 w592] -> w468
          frame False {
            n211 = Concatenate Strings("0", w590) -> (w589:string)
          }
          frame True {
          }
        }
        n212 = call "Trap Density_VT.vi"("VT"=w424, "Dielectric"=w423) -> ("Trap Density-VT"=w422:dbl)
        n213 = call "Trap Density_STS.vi"("Temp (T) [K]"=w418, "S.T.S. (S)"=w426, "Dielectric"=w425) -> ("Trap Density (N)"=w419:dbl)  [unwired: 8 in]
        n214 = local write "New: STS"(w426) -> ()
        n215 = local write "New: Trap Density-VT"(w422) -> ()
        n216 = local read "Index"() -> (w452:string)
        n217 = local write "New: Trap Density-STS"(w419) -> ()
        n218 = local read "Index"() -> (w466:string)
        n219 = local read "Wait Time (s):"() -> (w512:dbl)
        n220 = local write "New: Temp"(w418) -> ()
        n221 = String Subset(string=w452, length (rest)=1) -> (substring=w507:string)  [unwired: 1 in]
        n222 = local write "Row"(w507) -> ()
        n223 = local read "Treatment Concentration (mM):"() -> (w460:dbl)
        n224 = local read "Rec: Concentration"() -> (w447:dbl)
        n225 = local read "Relative Humidity (%):"() -> (w457:dbl)
        n226 = String Subset(string=w452, offset (0)=1, length (rest)=2) -> (substring=w508:string)
        n227 = Number To Decimal String(number=w512) -> (decimal integer string=w513:string)  [unwired: 1 in]
        n228 = local read "Solution Temp (C):"() -> (w501:dbl)
        n229 = local read "Surface Treatment:"() -> (w459:string)
        n230 = local read "Room Temp (F):"() -> (w505:dbl)
        n231 = local read "Rec: Material"() -> (w455:string)
        n232 = local write "Column"(w508) -> ()
        n233 = local read "New: Length"() -> (w465:dbl)
        n234 = local read "New: Width"() -> (w464:dbl)
        n235 = local read "New: Mobility-Sat"() -> (w494:dbl)
        n236 = local read "Accel (RPM/s):"() -> (w492:dbl)
        n237 = local read "Sample #:"() -> (w484:dbl)
        n238 = local read "# Drops*:"() -> (w502:dbl)
        n239 = local read "Ramp (s):"() -> (w510:dbl)
        n240 = local read "New: STS"() -> (w486:dbl)
        n241 = local read "Rec: Solvent"() -> (w461:string)
        n242 = local read "New: VT-Sat"() -> (w488:dbl)
        n243 = local read "Rec: On/Off"() -> (w490:dbl)
        n244 = local read "Rec: Method"() -> (w485:string)
        n245 = local read "Time (s):"() -> (w497:dbl)
        n246 = local read "Date Recorded"() -> (w481:string)
        n247 = local read "RPM:"() -> (w498:dbl)
        n248 = local read "Fabricator:"() -> (w506:string)
        n249 = Number To Decimal String(number=w447) -> (decimal integer string=w446:string)  [unwired: 1 in]
        n250 = Number To Decimal String(number=w502) -> (decimal integer string=w503:string)  [unwired: 1 in]
        n251 = Number To Decimal String(number=w484) -> (decimal integer string=w477:string)  [unwired: 1 in]
        n252 = call "DeviceID"("Sample"=w477, "Year"=w478, "Month"=w472, "Day"=w468, "Index"=w466) -> ("Result"=w483:string)  [unwired: 9 in, 1 out]
        n253 = Number To Decimal String(number=w465) -> (decimal integer string=w463:string)  [unwired: 1 in]
        n254 = Number To Decimal String(number=w464) -> (decimal integer string=w462:string)  [unwired: 1 in]
        n255 = Number To Decimal String(number=w501) -> (decimal integer string=w500:string)  [unwired: 1 in]
        n256 = Number To Decimal String(number=w457) -> (decimal integer string=w456:string)  [unwired: 1 in]
        n257 = Number To Decimal String(number=w505) -> (decimal integer string=w504:string)  [unwired: 1 in]
        n258 = property on="Image Out" class="ImageControl"() -> ("ZoomSingle"=w551:cluster{"X":sgl, "Y":sgl})  [unwired: 2 in, 2 out]
        n259 = Number To Decimal String(number=w460) -> (decimal integer string=w458:string)  [unwired: 1 in]
        n260 = property on="Image Out" class="ImageControl"() -> ("Bounds"=w552:T11)  [unwired: 2 in, 2 out]
        n261 = Number To Decimal String(number=w498) -> (decimal integer string=w499:string)  [unwired: 1 in]
        n262 = Number To Fractional String(number=w492) -> (F-format string=w493:string)  [unwired: 3 in]
        n263 = Number To Decimal String(number=w497) -> (decimal integer string=w496:string)  [unwired: 1 in]
        n264 = Number To Fractional String(number=w494) -> (F-format string=w495:string)  [unwired: 3 in]
        n265 = Number To Fractional String(number=w490) -> (F-format string=w491:string)  [unwired: 3 in]
        n266 = Number To Fractional String(number=w488) -> (F-format string=w489:string)  [unwired: 3 in]
        n267 = Number To Fractional String(number=w486) -> (F-format string=w487:string)  [unwired: 3 in]
        n268 = Number To Decimal String(number=w510) -> (decimal integer string=w511:string)  [unwired: 1 in]
        n269 = call <vilib>:"Intialize Keyboard.vi"() -> ("device ID"=w563:refnum<k1>)  [unwired: 10 in, 1 out]
        n270 = property on="Image Out" class="ImageControl"() -> ("Image Center Position"=w558:cluster{"X":u32, "Y":u32})  [unwired: 2 in, 2 out]
        n271 = call-poly <vilib>:"Acquire Input Data.vi"("device ID"=w563) -> ("keys pressed"=w562:T12)  [unwired: 16 in, 2 out]
        n272 = Unbundle(w552) -> ("Width"=w549:u32, "Height"=w548:u32)
        n273 = Unbundle(w551) -> ("X"=w526:sgl, "Y"=w550:sgl)
        n274 = Index Array(array=w562) -> (element=w566:T13)  [unwired: 1 in]
        n275 = event shown="[0] \"Remove Button\": Mouse Down" {
          selector: _ -> [_ _ _ _ _ _ _]
          dyn-events: _ -> [_ _ _ _ _ _ _]
          timeout: 10 -> [_ _ _ _ _ _ _]
          event "Remove Button": Mouse Down {
            w601 = 0
            n276 = event-data() -> ()  [unwired: 1 in, 7 out]
            n277 = property on="Image Out" class="ImageControl"() -> ("ROI"=w599:T10)  [unwired: 2 in, 2 out]
            n278 = Unbundle(w599) -> ("Global Rectangle"=w602:i32[], "Contours"=w604:T14)
            n279 = Reverse 1D Array(array=w602) -> (reversed array=w603:i32[])
            n280 = Reverse 1D Array(array=w604) -> (reversed array=w605:T14)
            n281 = Delete From Array(array=w603, index=w601) -> (array with subset deleted=w606:i32[])  [unwired: 1 in, 1 out]
            n282 = Delete From Array(array=w605, index=w601) -> (array with subset deleted=w607:T14)  [unwired: 1 in, 1 out]
            n283 = Reverse 1D Array(array=w606) -> (reversed array=w608:i32[])
            n284 = Reverse 1D Array(array=w607) -> (reversed array=w609:T14)
            n285 = Bundle(w608, w609) -> (w600:T15)  [unwired: 1 in]
            n286 = local write "ROI Descriptor out"(w599) -> ()
            n287 = local write "ROI Descriptor"(w600) -> ()
            n288 = property on="Image Out" class="ImageControl"("ROI"=w600) -> ()  [unwired: 2 in, 2 out]
          }
          event "Undo Button": Mouse Down {
            n289 = event-data() -> ()  [unwired: 1 in, 7 out]
            n290 = invoke on="Image Out" class="ImageControl" method="Clear ROI"() -> ()  [unwired: 3 in, 3 out]
          }
          event "Image Folder": Value Change {
            n291 = event-data() -> ()  [unwired: 1 in, 5 out]
            n292 = local read "Image File"() -> (w611:path)
            n293 = call "Vision Acquisition"("Image Path"=w611) -> ("Image Out"=w610:T2)  [unwired: 25 in, 1 out]
            n294 = local write "Image Out 2"(w610) -> ()
            n295 = local write "Image Out"(w610) -> ()
            n296 = invoke on="Image Out" class="ImageControl" method="Clear ROI"() -> ()  [unwired: 3 in, 3 out]
          }
          event "Zoom": Value Change {
            n297 = event-data() -> ()  [unwired: 1 in, 5 out]
            n298 = local read "Zoom"() -> (w612:i16)
            n299 = Bundle("Zoom"=w612, "Zoom"=w612) -> (w613:cluster{"Zoom":i16, "Zoom":i16})  [unwired: 1 in]
            n300 = property on="Image Out" class="ImageControl"("ZoomInteger"=w613) -> ()  [unwired: 2 in, 2 out]
          }
          event Timeout {
            n301 = event-data() -> ()  [unwired: 1 in, 2 out]
          }
          event "Image Out": Mouse Enter {
            (unwired) 6
            n302 = event-data() -> ()  [unwired: 1 in, 3 out]
            n303 = call "Simulate_Keyboard.vi"("Action"=0, "Virtual Key"=162) -> ()  [unwired: 7 in, 1 out]
          }
          event "Image Out": Mouse Leave {
            n304 = event-data() -> ()  [unwired: 1 in, 3 out]
            n305 = flat-sequence {
              frame #0 {
                n306 = Wait (ms)(milliseconds to wait=10) -> ()  [unwired: 1 out]
              }
              frame #1 {
                (unwired) 6
                n307 = call "Simulate_Keyboard.vi"("Action"=2, "Virtual Key"=162) -> ()  [unwired: 7 in, 1 out]
              }
            }
          }
        }
        n308 = Divide(x=w549, y=w526) -> (x/y=w539:sgl)
        n309 = Multiply(x=w539, y=0.5) -> (x*y=w545:dbl)
        n310 = Divide(x=w548, y=w550) -> (x/y=w538:sgl)
        n311 = Multiply(x=w538, y=0.5) -> (x*y=w544:dbl)
        n312 = Unbundle(w558) -> ("X"=w540:u32, "Y"=w541:u32)
        n313 = Subtract(x=w541, y=w544) -> (x-y=w542:dbl)
        n314 = Subtract(x=w540, y=w545) -> (x-y=w543:dbl)
        n315 = Add(x=w543, y=w539) -> (x+y=w557:dbl)
        n316 = Add(x=w542, y=w538) -> (x+y=w556:dbl)
        n317 = Build Array(w483, w506, w485, w481, w477, w507, w508, w463, w462, w455, w459, w458, w461, w446, w500, w503, w513, w504, w456, w511, w499, w493, w496, w495, w491, w489, w487) -> (w509:string[])
        n318 = local write "Current \nRecord"(w509) -> ()
        n319 = Reciprocal(x=w526) -> (1/x=w525:sgl)
        n320 = event shown="[13] \"Export\": Mouse Down" {
          selector: _ -> [_ _ _ _ _ _ _ _ _ _ _ _ _ _ _ _]
          dyn-events: _ -> [_ _ _ _ _ _ _ _ _ _ _ _ _ _ _ _]
          timeout: 10 -> [_ _ _ _ _ _ _ _ _ _ _ _ _ _ _ _]
          tunnel: [_ _ _ _ _ _ _ _ _ _ _ _ _ TRUE _ TRUE] -> w583
          event Timeout {
            n321 = event-data() -> ()  [unwired: 1 in, 2 out]
          }
          event "Down Button": Mouse Down {
            w953 = 0
            n322 = event-data() -> ()  [unwired: 1 in, 7 out]
            n323 = local read "Transfer File"() -> (w958:path)
            n324 = Strip Path(path=w958) -> (stripped path=w949:path, name=w967:string)
            n325 = local write "Transfer Folder"(w949) -> ()
            n326 = List Folder(path=w949) -> (filenames=w963:string[], error out=w903:errorcluster)  [unwired: 3 in, 2 out]
            n327 = local read "Folder Index"() -> (w905:dbl)
            n328 = property on="Image Out" class="ImageControl"() -> (error out=w906:errorcluster, "Image Center Position"=w910:cluster{"X":u32, "Y":u32})  [unwired: 2 in, 1 out]
            n329 = Array Size(array=w963) -> (size(s)=w959:i32)
            n330 = Search 1D Array(1D array=w963, element=w967) -> (index of element=w960:i32)  [unwired: 1 in]
            n331 = Decrement(x=w959) -> (x-1=w961:i32)
            n332 = Equal?(x=w960, y=w961) -> (x = y?=w962:bool)
            n333 = invoke on="Image Out" class="ImageControl" method="Clear ROI"() -> ()  [unwired: 3 in, 3 out]
            n334 = case shown="False" w962 {
              tunnel: w905 -> [w1120 _]
              tunnel: [w1119 0] -> w904
              tunnel: w903 -> [w1118 w1121]
              tunnel: [w1118 w1121] -> w902
              frame False {
                n335 = Increment(x=w1120) -> (x+1=w1119:dbl)
              }
              frame True {
              }
            }
            n336 = Unbundle(w910) -> ("X"=w908:u32)  [unwired: 1 out]
            n337 = local write "Folder Index"(w904) -> ()
            n338 = Bundle("X"=w908, 0) -> (w909:cluster{"X":u32, i32})  [unwired: 1 in]
            n339 = property on="Image Out" class="ImageControl"(error in=w906, "Image Center Position"=w909) -> ()  [unwired: 1 in, 2 out]
            n340 = Path To String(path=w949) -> (string=w968:string)
            n341 = Index Array(array=w963, index=w904) -> (element=w964:string)
            n342 = local write "Data Name:"(w964) -> ()
            n343 = Concatenate Strings(w968, "\\", w964) -> (w966:string)
            n344 = String To Path(string=w966) -> (path=w876:path)
            n345 = call "Recorded Values.vi"("Path"=w876) -> ("Recorded Char"=w970:T5, "Recorded Prop"=w971:T6, "Fabrication Prop"=w969:T7)  [unwired: 8 in]
            n346 = Unbundle By Name(w970) -> ("Mobility-Sat"=w983:dbl, "Moblitity-Lin"=w984:dbl, "On/Off"=w985:dbl, "Off Current"=w986:dbl, "Vt-Sat"=w871:dbl, "STS"=w987:dbl, "Trap Density-VT"=w988:dbl, "Trap Density-STS"=w989:dbl)
            n347 = Unbundle By Name(w969) -> ("Date Created"=w990:string, "Material"=w972:string, "Solvent"=w973:string, "Concentration"=w974:dbl, "Method"=w975:string, "Dielectric (nm)"=w976:dbl, "Treatment"=w977:string, "Comments"=w978:string)
            n348 = Unbundle By Name(w971) -> ("Date Recorded"=w979:string, "Index"=w980:string, "Length"=w981:dbl, "Width"=w982:dbl, "Sample Temp"=w873:dbl)
            n349 = local write "Date Created"(w990) -> ()
            n350 = local write "Rec: Off I-Sat"(w986) -> ()
            n351 = local write "Rec: Material"(w972) -> ()
            n352 = local write "Rec: VT-Sat"(w871) -> ()
            n353 = local write "Rec: Concentration"(w974) -> ()
            n354 = local write "Rec: Method"(w975) -> ()
            n355 = local write "Rec: Dielectric (d)"(w976) -> ()
            n356 = local write "Surface Treatment:"(w977) -> ()
            n357 = local write "Comments"(w978) -> ()
            n358 = local write "Index"(w980) -> ()
            n359 = local write "Rec: Mobility-Sat"(w983) -> ()
            n360 = local write "Rec: Mobility-Lin"(w984) -> ()
            n361 = local write "Rec: On/Off"(w985) -> ()
            n362 = local write "Rec: STS"(w987) -> ()
            n363 = local write "Rec: Trap Density-VT"(w988) -> ()
            n364 = local write "Rec: Trap Density-STS"(w989) -> ()
            n365 = local write "Rec: Solvent"(w973) -> ()
            n366 = local write "Date Recorded"(w979) -> ()
            n367 = local write "Rec: Length"(w981) -> ()
            n368 = local write "Rec: Width"(w982) -> ()
            n369 = local write "Rec: Temp"(w873) -> ()
            n370 = Equal To 0?(x=w873) -> (x = 0?=w874:bool)
            n371 = case shown="True" w874 {
              tunnel: [w991 w992] -> w872
              tunnel: w873 -> [w991 _]
              frame False {
              }
              frame True {
                n372 = local read "Room Temp"() -> (w992:dbl)
              }
            }
            n373 = local read "NumPts 2"() -> (w897:dbl)
            n374 = local write "Transfer File"(w876) -> ()
            n375 = local read "NumPts"() -> (w901:dbl)
            n376 = call-poly <vilib>:"Read From Spreadsheet File.vi"("file path (dialog if empty)"=w876) -> ("all rows"=w955:string[][])  [unwired: 6 in, 4 out]
            n377 = call "Mobility-Vt Calculator-File.vi"("NumPts"=w901, "Path"=w876) -> ("XY Graph-Sat"=w899:cluster{dbl[], dbl[]}[], "XY Graph-Lin"=w870:cluster{dbl[], dbl[]}[], "Output"=w900:T8, "Index-Sat"=w898:dbl, "Index-Lin"=w884:dbl)  [unwired: 4 in, 1 out]
            n378 = local read "New: Dielectric"() -> (w881:dbl)
            n379 = call "STS Calculator-File.vi"("NumPts"=w897, "Path"=w876) -> ("STS Index-Sat"=w896:dbl, "XY Graph-Sat"=w895:cluster{dbl[], dbl[]}[], "Ouput"=w894:cluster{"STS-Sat":dbl, "STS-Lin":dbl})  [unwired: 5 in, 2 out]
            n380 = Unbundle By Name(w900) -> ("Mobility-Sat"=w893:dbl, "Vt-Sat"=w880:dbl, "Mobility-Lin"=w892:dbl, "Vt-Lin"=w891:dbl, "Off I-Sat"=w877:dbl, "On/Off I-Sat"=w869:dbl)
            n381 = Unbundle By Name(w894) -> ("STS-Sat"=w875:dbl)  [unwired: 1 out]
            n382 = local write "Index 2"(w896) -> ()
            n383 = local write "XY Graph 2"(w895) -> ()
            n384 = local write "MobVi Index"(w898) -> ()
            n385 = local write "Slide"(w898) -> ()
            n386 = local write "XY Graph"(w899) -> ()
            n387 = Array Size(array=w955) -> (size(s)=w954:i32[])
            n388 = call "Trap Density_VT.vi"("VT"=w880, "Dielectric"=w881) -> ("Trap Density-VT"=w879:dbl)
            n389 = call "Trap Density_STS.vi"("Temp (T) [K]"=w872, "S.T.S. (S)"=w875, "Dielectric"=w881) -> ("Trap Density (N)"=w878:dbl)  [unwired: 8 in]
            n390 = local write "New: STS"(w875) -> ()
            n391 = local write "Calc: STS"(w875) -> ()
            n392 = local write "Calc: Mobility-Sat"(w893) -> ()
            n393 = local write "Calc: Off I-Sat"(w891) -> ()
            n394 = local write "Calc: Mobility-Lin"(w892) -> ()
            n395 = Index Array(array=w954, index=w953) -> (element=w935:i32)
            n396 = Decimate 1D Array(w895) -> (w929:cluster{dbl[], dbl[]}[])  [unwired: 1 out]
            n397 = Decimate 1D Array(w899) -> (w939:cluster{dbl[], dbl[]}[])  [unwired: 1 out]
            n398 = local write "Calc: Off I-Sat"(w877) -> ()
            n399 = local write "Calc: On/Off"(w869) -> ()
            n400 = Decimate 1D Array(w870) -> (w890:cluster{dbl[], dbl[]}[])  [unwired: 1 out]
            n401 = local write "Calc: VT-Sat"(w880) -> ()
            n402 = Array Subset(array=w955, index (row)=w953, index (col)=w953, length (col)=3) -> (w956:string[][])  [unwired: 1 in]
            n403 = local write "Calc: Trap Density-VT"(w879) -> ()
            n404 = local write "Calc: Trap Density-STS"(w878) -> ()
            n405 = local write "New: Trap Density-STS"(w878) -> ()
            n406 = local write "New: Trap Density-VT"(w879) -> ()
            n407 = local write "XY Graph-Lin"(w870) -> ()
            n408 = Array To Cluster(array=w929) -> (cluster=w927:T9)
            n409 = Array To Cluster(array=w939) -> (cluster=w941:T9)
            n410 = local write "New: VT-Lin"(w891) -> ()
            n411 = local write "New: VT-Sat"(w880) -> ()
            n412 = local write "New: Mobility-Sat"(w893) -> ()
            n413 = local write "New: Mobility-Lin"(w892) -> ()
            n414 = Reshape Array(w956, w935) -> (w942:string[])
            n415 = Array To Cluster(array=w890) -> (cluster=w889:T9)
            n416 = Subtract(x=w935, y=20) -> (x-y=w934:i32)
            n417 = property on="Slide" class="Slide (strict)"("Scale.Maximum"=w934) -> ()  [unwired: 2 in, 2 out]
            n418 = Unbundle(w927) -> ("[0]"=w928:cluster{dbl[], dbl[]})  [unwired: 8 out]
            n419 = Unbundle(w941) -> ("[0]"=w940:cluster{dbl[], dbl[]})  [unwired: 8 out]
            n420 = Unbundle(w889) -> ("[0]"=w886:cluster{dbl[], dbl[]})  [unwired: 8 out]
            n421 = Search 1D Array(1D array=w942, element="Index:") -> (index of element=w950:i32)  [unwired: 1 in]
            n422 = local read "NumPts"() -> (w885:dbl)
            n423 = Unbundle(w886) -> (w888:dbl[], w887:dbl[])
            n424 = Increment(x=w950) -> (x+1=w951:i32)
            n425 = Unbundle(w928) -> (w926:dbl[], w925:dbl[])
            n426 = Unbundle(w940) -> (w931:dbl[], w930:dbl[])
            n427 = Array Subset(array=w888, index=w884, length=w885) -> (w883:dbl[])
            n428 = Array Subset(array=w887, index=w884, length=w885) -> (w882:dbl[])
            n429 = Array Subset(array=w926, index=w896, length=w897) -> (w933:dbl[])
            n430 = Array Subset(array=w925, index=w896, length=w897) -> (w932:dbl[])
            n431 = Array Subset(array=w931, index=w898, length=w901) -> (w938:dbl[])
            n432 = Array Subset(array=w930, index=w898, length=w901) -> (w937:dbl[])
            n433 = Index Array(array=w942, index=w951) -> (element=w914:string)
            n434 = local write "Lin-Vg Array-Used"(w883) -> ()
            n435 = local write "Sat Vg Array-Used"(w938) -> ()
            n436 = local write "Vg Array-Log-Used"(w932) -> ()
            n437 = local write "Lin Id-Used"(w882) -> ()
            n438 = local read "Image Folder"() -> (w912:path)
            n439 = local write "Sat Id-Used"(w937) -> ()
            n440 = local write "Sat Id-Log-Used"(w933) -> ()
            n441 = List Folder(path=w912, error in=w902) -> (filenames=w948:string[], error out=w915:errorcluster)  [unwired: 2 in, 2 out]
            n442 = while {
              tunnel: w948 -> [w1005]
              tunnel: w914 -> [w1003]
              tunnel: [w1002] -> _
              tunnel: [w1002] -> w947
              tunnel: w935 -> [w1001]
              i -> [w1002]
              stop <- w998 stop-if-true
              n443 = Index Array(array=w1005, index=w1002) -> (element=w1006:string)
              n444 = xnode "Match Regular Expression"("input string"=w1006, "regular expression"=w1003) -> ("whole match"=w1004:string)  [unwired: 4 in, 4 out]
              n445 = Equal?(x=w1004, y=w1003) -> (x = y?=w1000:bool)
              n446 = Equal?(x=w1001, y=w1002) -> (x = y?=w999:bool)
              n447 = Or(x=w1000, y=w999) -> (x .or. y?=w998:bool)
            }
            n448 = Build Path(base path=w912, name or relative path="ROI") -> (appended path=w911:path)
            n449 = Path To String(path=w912) -> (string=w945:string)
            n450 = Index Array(array=w948, index=w947) -> (element=w923:string)
            n451 = invoke on="Image Out" class="ImageControl" method="Clear ROI"(error in=w915) -> (error out=w918:errorcluster)  [unwired: 2 in, 2 out]
            n452 = local write "Image Name"(w923) -> ()
            n453 = Build Path(base path=w911, name or relative path=w914) -> (appended path=w919:path)
            n454 = call <vilib>:"Check if File or Folder Exists.vi"("error in (no error)"=w918, "path"=w919) -> ("file or folder exists?"=w916:bool, "dup path"=w917:path)  [unwired: 7 in, 1 out]
            n455 = Concatenate Strings(w945, "\\", w923) -> (w944:string)
            n456 = case shown="False" w916 {
              tunnel: w917 -> [_ w993]
              frame False {
              }
              frame True {
                n457 = Read from Text File(file (use dialog)=w993) -> (text=w997:string)  [unwired: 3 in, 3 out]
                n458 = property on="Image Out" class="ImageControl"() -> ("ROI"=w994:T10)  [unwired: 2 in, 2 out]
                n459 = Unflatten From String(type=w994, binary string=w997) -> (value=w995:T10, error out=w996:errorcluster)  [unwired: 3 in, 1 out]
                n460 = property on="Image Out" class="ImageControl"(error in=w996, "ROI"=w995) -> ()  [unwired: 1 in, 2 out]
              }
            }
            n461 = String To Path(string=w944) -> (path=w922:path)
            n462 = Empty String/Path?(string/path=w923) -> (empty?=w924:bool)
            n463 = local read "No Image File"() -> (w920:path)
            n464 = Select(t=w920, s=w924, f=w922) -> (s? t:f=w921:path)
            n465 = local write "Image File"(w921) -> ()
            n466 = call "Vision Acquisition4"("Image Path"=w921) -> ("Image Out"=w946:T2)  [unwired: 25 in, 1 out]
            n467 = local write "Image Out"(w946) -> ()
            n468 = local write "Image Out 2"(w946) -> ()
          }
          event "Transfer File": Value Change {
            w1229 = 0
            n469 = event-data() -> ()  [unwired: 1 in, 5 out]
            n470 = local read "Transfer File"() -> (w1225:path)
            n471 = Strip Path(path=w1225) -> (stripped path=w1224:path, name=w1238:string)
            n472 = local write "Transfer Folder"(w1224) -> ()
            n473 = property on="Image Out" class="ImageControl"() -> (error out=w1180:errorcluster, "Image Center Position"=w1184:cluster{"X":u32, "Y":u32})  [unwired: 2 in, 1 out]
            n474 = List Folder(path=w1224) -> (filenames=w1234:string[], error out=w1190:errorcluster)  [unwired: 3 in, 2 out]
            n475 = Search 1D Array(1D array=w1234, element=w1238) -> (index of element=w1179:i32)  [unwired: 1 in]
            n476 = local write "Folder Index"(w1179) -> ()
            n477 = Unbundle(w1184) -> ("X"=w1182:u32)  [unwired: 1 out]
            n478 = Path To String(path=w1224) -> (string=w1239:string)
            n479 = Index Array(array=w1234, index=w1179) -> (element=w1235:string)
            n480 = Bundle("X"=w1182, 0) -> (w1183:cluster{"X":u32, i32})  [unwired: 1 in]
            n481 = local write "Data Name:"(w1235) -> ()
            n482 = property on="Image Out" class="ImageControl"(error in=w1180, "Image Center Position"=w1183) -> ()  [unwired: 1 in, 2 out]
            n483 = Concatenate Strings(w1239, "\\", w1235) -> (w1237:string)
            n484 = String To Path(string=w1237) -> (path=w1130:path)
            n485 = call "Recorded Values.vi"("Path"=w1130) -> ("Recorded Char"=w1177:T5, "Recorded Prop"=w1176:T6, "Fabrication Prop"=w1178:T7)  [unwired: 8 in]
            n486 = Unbundle By Name(w1177) -> ("Mobility-Sat"=w1164:dbl, "Moblitity-Lin"=w1163:dbl, "On/Off"=w1162:dbl, "Off Current"=w1161:dbl, "Vt-Sat"=w1126:dbl, "STS"=w1160:dbl, "Trap Density-VT"=w1159:dbl, "Trap Density-STS"=w1158:dbl)
            n487 = Unbundle By Name(w1178) -> ("Date Created"=w1157:string, "Material"=w1175:string, "Solvent"=w1174:string, "Concentration"=w1173:dbl, "Method"=w1172:string, "Dielectric (nm)"=w1171:dbl, "Treatment"=w1170:string, "Comments"=w1169:string)
            n488 = Unbundle By Name(w1176) -> ("Date Recorded"=w1168:string, "Index"=w1167:string, "Length"=w1166:dbl, "Width"=w1165:dbl, "Sample Temp"=w1128:dbl)
            n489 = local write "Date Created"(w1157) -> ()
            n490 = local write "Rec: Material"(w1175) -> ()
            n491 = local write "Rec: Off I-Sat"(w1161) -> ()
            n492 = local write "Rec: VT-Sat"(w1126) -> ()
            n493 = local write "Rec: Concentration"(w1173) -> ()
            n494 = local write "Rec: Method"(w1172) -> ()
            n495 = local write "Rec: Dielectric (d)"(w1171) -> ()
            n496 = local write "Surface Treatment:"(w1170) -> ()
            n497 = local write "Comments"(w1169) -> ()
            n498 = local write "Index"(w1167) -> ()
            n499 = local write "Rec: Mobility-Sat"(w1164) -> ()
            n500 = local write "Rec: Mobility-Lin"(w1163) -> ()
            n501 = local write "Rec: On/Off"(w1162) -> ()
            n502 = local write "Rec: STS"(w1160) -> ()
            n503 = local write "Rec: Trap Density-VT"(w1159) -> ()
            n504 = local write "Rec: Trap Density-STS"(w1158) -> ()
            n505 = local write "Rec: Solvent"(w1174) -> ()
            n506 = local write "Date Recorded"(w1168) -> ()
            n507 = local write "Rec: Length"(w1166) -> ()
            n508 = local write "Rec: Width"(w1165) -> ()
            n509 = local write "Rec: Temp"(w1128) -> ()
            n510 = Equal To 0?(x=w1128) -> (x = 0?=w1129:bool)
            n511 = case shown="False" w1129 {
              tunnel: [w1240 w1241] -> w1127
              tunnel: w1128 -> [w1240 _]
              frame False {
              }
              frame True {
                n512 = local read "Room Temp"() -> (w1241:dbl)
              }
            }
            n513 = local write "Transfer File"(w1130) -> ()
            n514 = local read "NumPts 2"() -> (w1152:dbl)
            n515 = local read "NumPts"() -> (w1153:dbl)
            n516 = call-poly <vilib>:"Read From Spreadsheet File.vi"("file path (dialog if empty)"=w1130) -> ("all rows"=w1231:string[][])  [unwired: 6 in, 4 out]
            n517 = local read "New: Dielectric"() -> (w1136:dbl)
            n518 = call "STS Calculator-File.vi"("NumPts"=w1152, "Path"=w1130) -> ("STS Index-Sat"=w1150:dbl, "XY Graph-Sat"=w1151:cluster{dbl[], dbl[]}[], "Ouput"=w1149:cluster{"STS-Sat":dbl, "STS-Lin":dbl})  [unwired: 5 in, 2 out]
            n519 = call "Mobility-Vt Calculator-File.vi"("NumPts"=w1153, "Path"=w1130) -> ("XY Graph-Sat"=w1156:cluster{dbl[], dbl[]}[], "XY Graph-Lin"=w1125:cluster{dbl[], dbl[]}[], "Output"=w1154:T8, "Index-Sat"=w1155:dbl, "Index-Lin"=w1142:dbl)  [unwired: 4 in, 1 out]
            n520 = Unbundle By Name(w1154) -> ("Mobility-Sat"=w1138:dbl, "Vt-Sat"=w1132:dbl, "Mobility-Lin"=w1137:dbl, "Vt-Lin"=w1123:dbl, "Off I-Sat"=w1131:dbl, "On/Off I-Sat"=w1124:dbl)
            n521 = local write "Index 2"(w1150) -> ()
            n522 = local write "XY Graph 2"(w1151) -> ()
            n523 = Unbundle By Name(w1149) -> ("STS-Sat"=w1133:dbl)  [unwired: 1 out]
            n524 = local write "MobVi Index"(w1155) -> ()
            n525 = Array Size(array=w1231) -> (size(s)=w1230:i32[])
            n526 = call "Trap Density_VT.vi"("VT"=w1132, "Dielectric"=w1136) -> ("Trap Density-VT"=w1135:dbl)
            n527 = call "Trap Density_STS.vi"("Temp (T) [K]"=w1127, "S.T.S. (S)"=w1133, "Dielectric"=w1136) -> ("Trap Density (N)"=w1134:dbl)  [unwired: 8 in]
            n528 = local write "Slide"(w1155) -> ()
            n529 = local write "Calc: Mobility-Lin"(w1137) -> ()
            n530 = local write "Calc: Mobility-Sat"(w1138) -> ()
            n531 = local write "Calc: VT-Sat"(w1132) -> ()
            n532 = local write "Calc: Off I-Sat"(w1131) -> ()
            n533 = local write "Calc: VT-Lin"(w1123) -> ()
            n534 = local write "Calc: On/Off"(w1124) -> ()
            n535 = local write "Calc: STS"(w1133) -> ()
            n536 = Decimate 1D Array(w1125) -> (w1148:cluster{dbl[], dbl[]}[])  [unwired: 1 out]
            n537 = local write "Calc: Trap Density-VT"(w1135) -> ()
            n538 = local write "Calc: Trap Density-STS"(w1134) -> ()
            n539 = local write "New: Trap Density-STS"(w1134) -> ()
            n540 = local write "New: Trap Density-VT"(w1135) -> ()
            n541 = local write "XY Graph-Lin"(w1125) -> ()
            n542 = local write "New: VT-Sat"(w1132) -> ()
            n543 = Decimate 1D Array(w1151) -> (w1205:cluster{dbl[], dbl[]}[])  [unwired: 1 out]
            n544 = Index Array(array=w1230, index=w1229) -> (element=w1211:i32)
            n545 = Decimate 1D Array(w1156) -> (w1214:cluster{dbl[], dbl[]}[])  [unwired: 1 out]
            n546 = local write "XY Graph"(w1156) -> ()
            n547 = local write "New: Mobility-Lin"(w1137) -> ()
            n548 = Array Subset(array=w1231, index (row)=w1229, index (col)=w1229, length (col)=3) -> (w1232:string[][])  [unwired: 1 in]
            n549 = local write "New: VT-Lin"(w1123) -> ()
            n550 = Array To Cluster(array=w1148) -> (cluster=w1147:T9)
            n551 = local write "New: STS"(w1133) -> ()
            n552 = local write "New: Mobility-Sat"(w1138) -> ()
            n553 = Array To Cluster(array=w1205) -> (cluster=w1203:T9)
            n554 = Array To Cluster(array=w1214) -> (cluster=w1216:T9)
            n555 = Reshape Array(w1232, w1211) -> (w1217:string[])
            n556 = Subtract(x=w1211, y=20) -> (x-y=w1209:i32)
            n557 = Unbundle(w1147) -> ("[0]"=w1146:cluster{dbl[], dbl[]})  [unwired: 8 out]
            n558 = property on="Slide" class="Slide (strict)"("Scale.Maximum"=w1209) -> ()  [unwired: 2 in, 2 out]
            n559 = local read "NumPts"() -> (w1143:dbl)
            n560 = Unbundle(w1146) -> (w1145:dbl[], w1144:dbl[])
            n561 = Unbundle(w1203) -> ("[0]"=w1204:cluster{dbl[], dbl[]})  [unwired: 8 out]
            n562 = Unbundle(w1216) -> ("[0]"=w1215:cluster{dbl[], dbl[]})  [unwired: 8 out]
            n563 = Search 1D Array(1D array=w1217, element="Index:") -> (index of element=w1226:i32)  [unwired: 1 in]
            n564 = local read "NumPts"() -> (w1139:dbl)
            n565 = Array Subset(array=w1145, index=w1142, length=w1143) -> (w1141:dbl[])
            n566 = Array Subset(array=w1144, index=w1142, length=w1143) -> (w1140:dbl[])
            n567 = Increment(x=w1226) -> (x+1=w1227:i32)
            n568 = Unbundle(w1204) -> (w1201:dbl[], w1200:dbl[])
            n569 = Unbundle(w1215) -> (w1202:dbl[], w1206:dbl[])
            n570 = local read "Image Folder"() -> (w1186:path)
            n571 = local write "Lin-Vg Array-Used"(w1141) -> ()
            n572 = Array Subset(array=w1201, index=w1150, length=w1152) -> (w1208:dbl[])
            n573 = Array Subset(array=w1200, index=w1150, length=w1152) -> (w1207:dbl[])
            n574 = Array Subset(array=w1202, index=w1155, length=w1139) -> (w1213:dbl[])
            n575 = Array Subset(array=w1206, index=w1155, length=w1139) -> (w1212:dbl[])
            n576 = Index Array(array=w1217, index=w1227) -> (element=w1188:string)
            n577 = local write "Lin Id-Used"(w1140) -> ()
            n578 = local write "Sat Vg Array-Used"(w1213) -> ()
            n579 = local write "Vg Array-Log-Used"(w1207) -> ()
            n580 = local write "Sat Id-Log-Used"(w1208) -> ()
            n581 = local write "Sat Id-Used"(w1212) -> ()
            n582 = local write "Index"(w1188) -> ()
            n583 = List Folder(path=w1186, error in=w1190) -> (filenames=w1222:string[], error out=w1189:errorcluster)  [unwired: 2 in, 2 out]
            n584 = Build Path(base path=w1186, name or relative path="ROI") -> (appended path=w1185:path)
            n585 = invoke on="Image Out" class="ImageControl" method="Clear ROI"(error in=w1189) -> (error out=w1193:errorcluster)  [unwired: 2 in, 2 out]
            n586 = Build Path(base path=w1185, name or relative path=w1188) -> (appended path=w1194:path)
            n587 = while {
              tunnel: w1222 -> [w1254]
              tunnel: w1188 -> [w1252]
              tunnel: [w1251] -> _
              tunnel: [w1251] -> w1221
              tunnel: w1211 -> [w1250]
              i -> [w1251]
              stop <- w1247 stop-if-true
              n588 = Index Array(array=w1254, index=w1251) -> (element=w1255:string)
              n589 = xnode "Match Regular Expression"("input string"=w1255, "regular expression"=w1252) -> ("whole match"=w1253:string)  [unwired: 4 in, 4 out]
              n590 = Equal?(x=w1253, y=w1252) -> (x = y?=w1249:bool)
              n591 = Equal?(x=w1250, y=w1251) -> (x = y?=w1248:bool)
              n592 = Or(x=w1249, y=w1248) -> (x .or. y?=w1247:bool)
            }
            n593 = call <vilib>:"Check if File or Folder Exists.vi"("error in (no error)"=w1193, "path"=w1194) -> ("file or folder exists?"=w1191:bool, "dup path"=w1192:path)  [unwired: 7 in, 1 out]
            n594 = case shown="True" w1191 {
              tunnel: w1192 -> [_ w1242]
              frame False {
              }
              frame True {
                n595 = Read from Text File(file (use dialog)=w1242) -> (text=w1246:string)  [unwired: 3 in, 3 out]
                n596 = property on="Image Out" class="ImageControl"() -> ("ROI"=w1243:T10)  [unwired: 2 in, 2 out]
                n597 = Unflatten From String(type=w1243, binary string=w1246) -> (value=w1244:T10, error out=w1245:errorcluster)  [unwired: 3 in, 1 out]
                n598 = property on="Image Out" class="ImageControl"(error in=w1245, "ROI"=w1244) -> ()  [unwired: 1 in, 2 out]
              }
            }
            n599 = invoke on="Image Out" class="ImageControl" method="Clear ROI"() -> ()  [unwired: 3 in, 3 out]
            n600 = Path To String(path=w1186) -> (string=w1220:string)
            n601 = Index Array(array=w1222, index=w1221) -> (element=w1198:string)
            n602 = Concatenate Strings(w1220, "\\", w1198) -> (w1219:string)
            n603 = local write "Image Name"(w1198) -> ()
            n604 = String To Path(string=w1219) -> (path=w1197:path)
            n605 = Empty String/Path?(string/path=w1198) -> (empty?=w1199:bool)
            n606 = local read "No Image File"() -> (w1195:path)
            n607 = Select(t=w1195, s=w1199, f=w1197) -> (s? t:f=w1196:path)
            n608 = local write "Image File"(w1196) -> ()
            n609 = call "Vision Acquisition3"("Image Path"=w1196) -> ("Image Out"=w1223:T2)  [unwired: 25 in, 1 out]
            n610 = local write "Image Out"(w1223) -> ()
            n611 = local write "Image Out 2"(w1223) -> ()
          }
          event "Up Button": Mouse Down {
            w1474 = 0
            n612 = event-data() -> ()  [unwired: 1 in, 5 out]
            n613 = local read "Transfer File"() -> (w1470:path)
            n614 = Strip Path(path=w1470) -> (stripped path=w1469:path, name=w1485:string)
            n615 = local write "Transfer Folder"(w1469) -> ()
            n616 = List Folder(path=w1469) -> (filenames=w1479:string[], error out=w1436:errorcluster)  [unwired: 3 in, 2 out]
            n617 = Array Size(array=w1479) -> (size(s)=w1424:i32)
            n618 = Search 1D Array(1D array=w1479, element=w1485) -> (index of element=w1480:i32)  [unwired: 1 in]
            n619 = Equal To 0?(x=w1480) -> (x = 0?=w1481:bool)
            n620 = local read "Folder Index"() -> (w1423:dbl)
            n621 = property on="Image Out" class="ImageControl"() -> (error out=w1426:errorcluster, "Image Center Position"=w1430:cluster{"X":u32, "Y":u32})  [unwired: 2 in, 1 out]
            n622 = case shown="True" w1481 {
              tunnel: w1423 -> [w1615 _]
              tunnel: [w1614 w1616] -> w1422
              tunnel: w1424 -> [_ w1617]
              frame False {
                n623 = Decrement(x=w1615) -> (x-1=w1614:dbl)
              }
              frame True {
                n624 = Decrement(x=w1617) -> (x-1=w1616:i32)
              }
            }
            n625 = Unbundle(w1430) -> ("X"=w1428:u32)  [unwired: 1 out]
            n626 = local write "Folder Index"(w1422) -> ()
            n627 = Bundle("X"=w1428, 0) -> (w1429:cluster{"X":u32, i32})  [unwired: 1 in]
            n628 = Path To String(path=w1469) -> (string=w1486:string)
            n629 = Index Array(array=w1479, index=w1422) -> (element=w1482:string)
            n630 = local write "Data Name:"(w1482) -> ()
            n631 = property on="Image Out" class="ImageControl"(error in=w1426, "Image Center Position"=w1429) -> ()  [unwired: 1 in, 2 out]
            n632 = Concatenate Strings(w1486, "\\", w1482) -> (w1484:string)
            n633 = String To Path(string=w1484) -> (path=w1373:path)
            n634 = call "Recorded Values.vi"("Path"=w1373) -> ("Recorded Char"=w1420:T5, "Recorded Prop"=w1419:T6, "Fabrication Prop"=w1421:T7)  [unwired: 8 in]
            n635 = Unbundle By Name(w1420) -> ("Mobility-Sat"=w1407:dbl, "Moblitity-Lin"=w1406:dbl, "On/Off"=w1405:dbl, "Off Current"=w1404:dbl, "Vt-Sat"=w1369:dbl, "STS"=w1403:dbl, "Trap Density-VT"=w1402:dbl, "Trap Density-STS"=w1401:dbl)
            n636 = Unbundle By Name(w1421) -> ("Date Created"=w1400:string, "Material"=w1418:string, "Solvent"=w1417:string, "Concentration"=w1416:dbl, "Method"=w1415:string, "Dielectric (nm)"=w1414:dbl, "Treatment"=w1413:string, "Comments"=w1412:string)
            n637 = Unbundle By Name(w1419) -> ("Date Recorded"=w1411:string, "Index"=w1410:string, "Length"=w1409:dbl, "Width"=w1408:dbl, "Sample Temp"=w1370:dbl)
            n638 = local write "Date Created"(w1400) -> ()
            n639 = local write "Rec: Material"(w1418) -> ()
            n640 = local write "Rec: Off I-Sat"(w1404) -> ()
            n641 = local write "Rec: VT-Sat"(w1369) -> ()
            n642 = local write "Rec: Solvent"(w1417) -> ()
            n643 = local write "Rec: Concentration"(w1416) -> ()
            n644 = local write "Rec: Method"(w1415) -> ()
            n645 = local write "Rec: Dielectric (d)"(w1414) -> ()
            n646 = local write "Surface Treatment:"(w1413) -> ()
            n647 = local write "Comments"(w1412) -> ()
            n648 = local write "Index"(w1410) -> ()
            n649 = local write "Rec: Mobility-Sat"(w1407) -> ()
            n650 = local write "Rec: Mobility-Lin"(w1406) -> ()
            n651 = local write "Rec: On/Off"(w1405) -> ()
            n652 = local write "Rec: STS"(w1403) -> ()
            n653 = local write "Rec: Trap Density-VT"(w1402) -> ()
            n654 = local write "Rec: Trap Density-STS"(w1401) -> ()
            n655 = local write "Date Recorded"(w1411) -> ()
            n656 = local write "Rec: Length"(w1409) -> ()
            n657 = local write "Rec: Width"(w1408) -> ()
            n658 = local write "Rec: Temp"(w1370) -> ()
            n659 = Equal To 0?(x=w1370) -> (x = 0?=w1372:bool)
            n660 = case shown="False" w1372 {
              tunnel: [w1487 w1488] -> w1371
              tunnel: w1370 -> [w1487 _]
              frame False {
              }
              frame True {
                n661 = local read "Room Temp"() -> (w1488:dbl)
              }
            }
            n662 = local write "Transfer File"(w1373) -> ()
            n663 = local read "NumPts 2"() -> (w1395:dbl)
            n664 = local read "NumPts"() -> (w1399:dbl)
            n665 = local read "New: Dielectric"() -> (w1379:dbl)
            n666 = call "Mobility-Vt Calculator-File.vi"("NumPts"=w1399, "Path"=w1373) -> ("XY Graph-Sat"=w1397:cluster{dbl[], dbl[]}[], "XY Graph-Lin"=w1368:cluster{dbl[], dbl[]}[], "Output"=w1398:T8, "Index-Sat"=w1396:dbl, "Index-Lin"=w1383:dbl)  [unwired: 4 in, 1 out]
            n667 = call "STS Calculator-File.vi"("NumPts"=w1395, "Path"=w1373) -> ("STS Index-Sat"=w1394:dbl, "XY Graph-Sat"=w1393:cluster{dbl[], dbl[]}[], "Ouput"=w1392:cluster{"STS-Sat":dbl, "STS-Lin":dbl})  [unwired: 5 in, 2 out]
            n668 = call-poly <vilib>:"Read From Spreadsheet File.vi"("file path (dialog if empty)"=w1373) -> ("all rows"=w1476:string[][])  [unwired: 6 in, 4 out]
            n669 = Unbundle By Name(w1398) -> ("Mobility-Sat"=w1382:dbl, "Vt-Sat"=w1375:dbl, "Mobility-Lin"=w1381:dbl, "Vt-Lin"=w1380:dbl, "Off I-Sat"=w1374:dbl, "On/Off I-Sat"=w1367:dbl)
            n670 = Unbundle By Name(w1392) -> ("STS-Sat"=w1376:dbl)  [unwired: 1 out]
            n671 = local write "Index 2"(w1394) -> ()
            n672 = local write "XY Graph 2"(w1393) -> ()
            n673 = local write "MobVi Index"(w1396) -> ()
            n674 = local write "Slide"(w1396) -> ()
            n675 = local write "XY Graph"(w1397) -> ()
            n676 = local write "Calc: Mobility-Sat"(w1382) -> ()
            n677 = local write "Calc: VT-Sat"(w1375) -> ()
            n678 = local write "Calc: Mobility-Lin"(w1381) -> ()
            n679 = local write "Calc: Off I-Sat"(w1374) -> ()
            n680 = local write "Calc: On/Off"(w1367) -> ()
            n681 = Array Size(array=w1476) -> (size(s)=w1475:i32[])
            n682 = local write "Calc: VT-Lin"(w1380) -> ()
            n683 = call "Trap Density_VT.vi"("VT"=w1375, "Dielectric"=w1379) -> ("Trap Density-VT"=w1378:dbl)
            n684 = call "Trap Density_STS.vi"("Temp (T) [K]"=w1371, "S.T.S. (S)"=w1376, "Dielectric"=w1379) -> ("Trap Density (N)"=w1377:dbl)  [unwired: 8 in]
            n685 = local write "Calc: STS"(w1376) -> ()
            n686 = local write "New: STS"(w1376) -> ()
            n687 = Decimate 1D Array(w1368) -> (w1391:cluster{dbl[], dbl[]}[])  [unwired: 1 out]
            n688 = local write "Calc: Trap Density-VT"(w1378) -> ()
            n689 = local write "New: VT-Sat"(w1375) -> ()
            n690 = local write "Calc: Trap Density-STS"(w1377) -> ()
            n691 = local write "New: Trap Density-STS"(w1377) -> ()
            n692 = local write "New: Trap Density-VT"(w1378) -> ()
            n693 = local write "XY Graph-Lin"(w1368) -> ()
            n694 = local write "New: VT-Lin"(w1380) -> ()
            n695 = local write "New: Mobility-Sat"(w1382) -> ()
            n696 = local write "New: Mobility-Lin"(w1381) -> ()
            n697 = Decimate 1D Array(w1393) -> (w1453:cluster{dbl[], dbl[]}[])  [unwired: 1 out]
            n698 = Index Array(array=w1475, index=w1474) -> (element=w1459:i32)
            n699 = Decimate 1D Array(w1397) -> (w1463:cluster{dbl[], dbl[]}[])  [unwired: 1 out]
            n700 = Array To Cluster(array=w1391) -> (cluster=w1390:T9)
            n701 = Array Subset(array=w1476, index (row)=w1474, index (col)=w1474, length (col)=3) -> (w1477:string[][])  [unwired: 1 in]
            n702 = Array To Cluster(array=w1453) -> (cluster=w1451:T9)
            n703 = Array To Cluster(array=w1463) -> (cluster=w1465:T9)
            n704 = Reshape Array(w1477, w1459) -> (w1466:string[])
            n705 = Subtract(x=w1459, y=20) -> (x-y=w1458:i32)
            n706 = Unbundle(w1390) -> ("[0]"=w1387:cluster{dbl[], dbl[]})  [unwired: 8 out]
            n707 = property on="Slide" class="Slide (strict)"("Scale.Maximum"=w1458) -> ()  [unwired: 2 in, 2 out]
            n708 = Unbundle(w1451) -> ("[0]"=w1452:cluster{dbl[], dbl[]})  [unwired: 8 out]
            n709 = Unbundle(w1465) -> ("[0]"=w1464:cluster{dbl[], dbl[]})  [unwired: 8 out]
            n710 = local read "NumPts"() -> (w1384:dbl)
            n711 = Unbundle(w1387) -> (w1386:dbl[], w1385:dbl[])
            n712 = Search 1D Array(1D array=w1466, element="Index:") -> (index of element=w1471:i32)  [unwired: 1 in]
            n713 = Increment(x=w1471) -> (x+1=w1472:i32)
            n714 = Unbundle(w1452) -> (w1450:dbl[], w1449:dbl[])
            n715 = Unbundle(w1464) -> (w1457:dbl[], w1456:dbl[])
            n716 = Array Subset(array=w1386, index=w1383, length=w1384) -> (w1388:dbl[])
            n717 = Array Subset(array=w1385, index=w1383, length=w1384) -> (w1389:dbl[])
            n718 = local read "Image Folder"() -> (w1425:path)
            n719 = local write "Lin-Vg Array-Used"(w1388) -> ()
            n720 = Array Subset(array=w1450, index=w1394, length=w1395) -> (w1455:dbl[])
            n721 = Array Subset(array=w1449, index=w1394, length=w1395) -> (w1454:dbl[])
            n722 = Array Subset(array=w1457, index=w1396, length=w1399) -> (w1462:dbl[])
            n723 = Array Subset(array=w1456, index=w1396, length=w1399) -> (w1461:dbl[])
            n724 = local write "Lin Id-Used"(w1389) -> ()
            n725 = Index Array(array=w1466, index=w1472) -> (element=w1432:string)
            n726 = local write "Sat Vg Array-Used"(w1462) -> ()
            n727 = local write "Vg Array-Log-Used"(w1454) -> ()
            n728 = local write "Sat Id-Log-Used"(w1455) -> ()
            n729 = local write "Sat Id-Used"(w1461) -> ()
            n730 = local write "Index"(w1432) -> ()
            n731 = List Folder(path=w1425, error in=w1436) -> (filenames=w1468:string[], error out=w1435:errorcluster)  [unwired: 2 in, 2 out]
            n732 = Build Path(base path=w1425, name or relative path="ROI") -> (appended path=w1433:path)
            n733 = while {
              tunnel: w1468 -> [w1501]
              tunnel: w1432 -> [w1499]
              tunnel: [w1498] -> w1467
              tunnel: w1459 -> [w1497]
              i -> [w1498]
              stop <- w1494 stop-if-true
              n734 = Index Array(array=w1501, index=w1498) -> (element=w1502:string)
              n735 = xnode "Match Regular Expression"("input string"=w1502, "regular expression"=w1499) -> ("whole match"=w1500:string)  [unwired: 4 in, 4 out]
              n736 = Equal?(x=w1500, y=w1499) -> (x = y?=w1496:bool)
              n737 = Equal?(x=w1497, y=w1498) -> (x = y?=w1495:bool)
              n738 = Or(x=w1496, y=w1495) -> (x .or. y?=w1494:bool)
            }
            n739 = invoke on="Image Out" class="ImageControl" method="Clear ROI"(error in=w1435) -> (error out=w1439:errorcluster)  [unwired: 2 in, 2 out]
            n740 = Build Path(base path=w1433, name or relative path=w1432) -> (appended path=w1431:path)
            n741 = call <vilib>:"Check if File or Folder Exists.vi"("error in (no error)"=w1439, "path"=w1431) -> ("file or folder exists?"=w1437:bool, "dup path"=w1438:path)  [unwired: 7 in, 1 out]
            n742 = case shown="True" w1437 {
              tunnel: w1438 -> [_ w1489]
              frame False {
              }
              frame True {
                n743 = Read from Text File(file (use dialog)=w1489) -> (text=w1493:string)  [unwired: 3 in, 3 out]
                n744 = property on="Image Out" class="ImageControl"() -> ("ROI"=w1490:T10)  [unwired: 2 in, 2 out]
                n745 = Unflatten From String(type=w1490, binary string=w1493) -> (value=w1491:T10, error out=w1492:errorcluster)  [unwired: 3 in, 1 out]
                n746 = property on="Image Out" class="ImageControl"(error in=w1492, "ROI"=w1491) -> ()  [unwired: 1 in, 2 out]
              }
            }
            n747 = Index Array(array=w1468, index=w1467) -> (element=w1441:string)
            n748 = local write "Image Name"(w1441) -> ()
            n749 = Empty String/Path?(string/path=w1441) -> (empty?=w1448:bool)
            n750 = Build Path(base path=w1425, name or relative path=w1441) -> (appended path=w1440:path)
            n751 = local read "No Image File"() -> (w1447:path)
            n752 = Select(t=w1447, s=w1448, f=w1440) -> (s? t:f=w1442:path)
            n753 = call <vilib>:"Get File Extension.vi"("file"=w1442) -> ("lowercase file extension"=w1444:string)  [unwired: 7 in, 3 out]
            n754 = local write "Image File"(w1442) -> ()
            n755 = local write "String"(w1444) -> ()
            n756 = Search 1D Array(1D array=string[] ["bmp", "jpeg", "png", "jpg", "gif"], element=w1444) -> (index of element=w1443:i32)  [unwired: 1 in]
            n757 = call "Vision Acquisition5"("Image Path"=w1442) -> ("Image Out"=w1446:T2)  [unwired: 25 in, 1 out]
            n758 = Less Than 0?(x=w1443) -> ()  [unwired: 1 out]
            n759 = local write "Image Out"(w1446) -> ()
            n760 = local write "Image Out 2"(w1446) -> ()
          }
          event "Save Changes? 3": Mouse Down {
            n761 = event-data() -> ()  [unwired: 1 in, 7 out]
            n762 = local read "Image Folder"() -> (w1618:path)
            n763 = Build Path(base path=w1618, name or relative path="ROI") -> (appended path=w1625:path)
            n764 = call <vilib>:"Check if File or Folder Exists.vi"("path"=w1625) -> ("file or folder exists?"=w1627:bool, "dup path"=w1624:path)  [unwired: 8 in, 1 out]
            n765 = case shown="False" w1627 {
              tunnel: w1624 -> [w1629 w1630]
              tunnel: [w1628 w1630] -> w1619
              frame False {
                n766 = Create Folder(path (use dialog)=w1629) -> (created path=w1628:path)  [unwired: 2 in, 2 out]
              }
              frame True {
              }
            }
            n767 = local read "Index"() -> (w1621:string)
            n768 = property on="Image Out" class="ImageControl"() -> ("ROI"=w1623:T10)  [unwired: 2 in, 2 out]
            n769 = Build Path(base path=w1619, name or relative path=w1621) -> (appended path=w1620:path)
            n770 = Flatten To String(anything=w1623) -> (data string=w1622:string)  [unwired: 3 in, 2 out]
            n771 = Write to Text File(file (use dialog)=w1620, text=w1622) -> ()  [unwired: 2 in, 3 out]
          }
          event "Next Button": Mouse Down {
            n772 = event-data() -> ()  [unwired: 1 in, 5 out]
            n773 = local read "XY Graph"() -> (w1643:cluster{dbl[], dbl[]}[])
            n774 = Decimate 1D Array(w1643) -> (w1639:cluster{dbl[], dbl[]}[], w1638:cluster{dbl[], dbl[]}[])
            n775 = Array To Cluster(array=w1639) -> (cluster=w1649:T9)
            n776 = local read "MobVi Index"() -> (w1645:dbl)
            n777 = Unbundle(w1649) -> ("[0]"=w1648:cluster{dbl[], dbl[]})  [unwired: 8 out]
            n778 = local read "NumPts"() -> (w1644:dbl)
            n779 = Unbundle(w1648) -> (w1647:dbl[], w1646:dbl[])
            n780 = Increment(x=w1645) -> (x+1=w1640:dbl)
            n781 = local read "New: Dielectric"() -> (w1634:dbl)
            n782 = local read "New: Length"() -> (w1633:dbl)
            n783 = local read "New: Width"() -> (w1632:dbl)
            n784 = local write "MobVi Index"(w1640) -> ()
            n785 = Array Subset(array=w1647, index=w1640, length=w1644) -> (w1636:dbl[])
            n786 = Array Subset(array=w1646, index=w1640, length=w1644) -> (w1635:dbl[])
            n787 = local write "Sat Vg Array-Used"(w1636) -> ()
            n788 = local write "Sat Id-Used"(w1635) -> ()
            n789 = call "Mobility-Vt-Used Pts_Saturation.vi"("Width"=w1632, "Length"=w1633, "Dielectric (d)"=w1634, "Sat Id Used"=w1635, "Vg Used"=w1636) -> ("Vt"=w1631:dbl, "Mobility"=w1637:dbl)  [unwired: 4 in, 1 out]
            n790 = Bundle(w1636, w1635) -> (w1642:cluster{dbl[], dbl[]})  [unwired: 1 in]
            n791 = Build Array (concatenate)(w1639, w1638, w1642) -> (w1641:cluster{dbl[], dbl[]}[])
            n792 = local write "New: Mobility-Sat"(w1637) -> ()
            n793 = local write "New: VT-Sat"(w1631) -> ()
            n794 = local write "XY Graph"(w1641) -> ()
          }
          event "Next Button 2": Mouse Down {
            n795 = event-data() -> ()  [unwired: 1 in, 7 out]
            n796 = local read "XY Graph 2"() -> (w1658:cluster{dbl[], dbl[]}[])
            n797 = Decimate 1D Array(w1658) -> (w1654:cluster{dbl[], dbl[]}[], w1653:cluster{dbl[], dbl[]}[])
            n798 = Array To Cluster(array=w1654) -> (cluster=w1664:T9)
            n799 = local read "Index 2"() -> (w1660:dbl)
            n800 = Unbundle(w1664) -> ("[0]"=w1663:cluster{dbl[], dbl[]})  [unwired: 8 out]
            n801 = local read "NumPts 2"() -> (w1659:dbl)
            n802 = Unbundle(w1663) -> (w1662:dbl[], w1661:dbl[])
            n803 = Increment(x=w1660) -> (x+1=w1655:dbl)
            n804 = local write "Index 2"(w1655) -> ()
            n805 = Array Subset(array=w1661, index=w1655, length=w1659) -> (w1650:dbl[])
            n806 = Array Subset(array=w1662, index=w1655, length=w1659) -> (w1651:dbl[])
            n807 = call "STS-Used.vi"("Id Used"=w1651, "Vg-Used"=w1650) -> ("STS"=w1652:dbl)  [unwired: 9 in]
            n808 = Bundle(w1651, w1650) -> (w1657:cluster{dbl[], dbl[]})  [unwired: 1 in]
            n809 = local write "Vg Array-Log-Used"(w1650) -> ()
            n810 = local write "Sat Id-Log-Used"(w1651) -> ()
            n811 = local write "New: STS"(w1652) -> ()
            n812 = Build Array (concatenate)(w1654, w1653, w1657) -> (w1656:cluster{dbl[], dbl[]}[])
            n813 = local write "XY Graph 2"(w1656) -> ()
          }
          event "Previous Button 2": Mouse Down {
            n814 = event-data() -> ()  [unwired: 1 in, 7 out]
            n815 = local read "XY Graph 2"() -> (w1674:cluster{dbl[], dbl[]}[])
            n816 = Decimate 1D Array(w1674) -> (w1671:cluster{dbl[], dbl[]}[], w1670:cluster{dbl[], dbl[]}[])
            n817 = Array To Cluster(array=w1671) -> (cluster=w1679:T9)
            n818 = local read "Index 2"() -> (w1667:dbl)
            n819 = Unbundle(w1679) -> ("[0]"=w1678:cluster{dbl[], dbl[]})  [unwired: 8 out]
            n820 = local read "NumPts 2"() -> (w1675:dbl)
            n821 = Unbundle(w1678) -> (w1677:dbl[], w1676:dbl[])
            n822 = Decrement(x=w1667) -> (x-1=w1668:dbl)
            n823 = local write "Index 2"(w1668) -> ()
            n824 = Array Subset(array=w1677, index=w1668, length=w1675) -> (w1665:dbl[])
            n825 = Array Subset(array=w1676, index=w1668, length=w1675) -> (w1666:dbl[])
            n826 = local write "Vg Array-Log-Used"(w1666) -> ()
            n827 = local write "Sat Id-Log-Used"(w1665) -> ()
            n828 = Bundle(w1665, w1666) -> (w1673:cluster{dbl[], dbl[]})  [unwired: 1 in]
            n829 = call "STS-Used.vi"("Id Used"=w1665, "Vg-Used"=w1666) -> ("STS"=w1669:dbl)  [unwired: 9 in]
            n830 = Build Array (concatenate)(w1671, w1670, w1673) -> (w1672:cluster{dbl[], dbl[]}[])
            n831 = local write "New: STS"(w1669) -> ()
            n832 = local write "XY Graph 2"(w1672) -> ()
          }
          event "Previous Button": Mouse Down {
            n833 = event-data() -> ()  [unwired: 1 in, 5 out]
            n834 = local read "XY Graph"() -> (w1693:cluster{dbl[], dbl[]}[])
            n835 = Decimate 1D Array(w1693) -> (w1690:cluster{dbl[], dbl[]}[], w1689:cluster{dbl[], dbl[]}[])
            n836 = Array To Cluster(array=w1690) -> (cluster=w1698:T9)
            n837 = local read "MobVi Index"() -> (w1688:dbl)
            n838 = Unbundle(w1698) -> ("[0]"=w1697:cluster{dbl[], dbl[]})  [unwired: 8 out]
            n839 = local read "NumPts"() -> (w1694:dbl)
            n840 = Unbundle(w1697) -> (w1696:dbl[], w1695:dbl[])
            n841 = Decrement(x=w1688) -> (x-1=w1687:dbl)
            n842 = local read "New: Dielectric"() -> (w1681:dbl)
            n843 = local read "New: Length"() -> (w1682:dbl)
            n844 = local read "New: Width"() -> (w1683:dbl)
            n845 = local write "MobVi Index"(w1687) -> ()
            n846 = Array Subset(array=w1696, index=w1687, length=w1694) -> (w1686:dbl[])
            n847 = Array Subset(array=w1695, index=w1687, length=w1694) -> (w1685:dbl[])
            n848 = local write "Sat Vg Array-Used"(w1686) -> ()
            n849 = local write "Sat Id-Used"(w1685) -> ()
            n850 = call "Mobility-Vt-Used Pts_Linear.vi"("Width"=w1683, "Length"=w1682, "Dielectric (d)"=w1681, "Sat Id Used"=w1685, "Vg Used"=w1686) -> ("Vt"=w1680:dbl, "Mobility"=w1684:dbl)  [unwired: 4 in, 1 out]
            n851 = Bundle(w1686, w1685) -> (w1692:cluster{dbl[], dbl[]})  [unwired: 1 in]
            n852 = local write "New: VT-Sat"(w1680) -> ()
            n853 = Build Array (concatenate)(w1690, w1689, w1692) -> (w1691:cluster{dbl[], dbl[]}[])
            n854 = local write "New: Mobility-Sat"(w1684) -> ()
            n855 = local write "XY Graph"(w1691) -> ()
          }
          event "Slide": Value Change {
            n856 = event-data() -> ()  [unwired: 1 in, 5 out]
            n857 = local read "XY Graph"() -> (w1711:cluster{dbl[], dbl[]}[])
            n858 = Decimate 1D Array(w1711) -> (w1708:cluster{dbl[], dbl[]}[], w1707:cluster{dbl[], dbl[]}[])
            n859 = Array To Cluster(array=w1708) -> (cluster=w1716:T9)
            n860 = Unbundle(w1716) -> ("[0]"=w1715:cluster{dbl[], dbl[]})  [unwired: 8 out]
            n861 = local read "NumPts"() -> (w1712:dbl)
            n862 = local read "Slide"() -> (w1700:dbl)
            n863 = Unbundle(w1715) -> (w1714:dbl[], w1713:dbl[])
            n864 = local read "New: Dielectric"() -> (w1701:dbl)
            n865 = local read "New: Length"() -> (w1702:dbl)
            n866 = local read "New: Width"() -> (w1703:dbl)
            n867 = local write "MobVi Index"(w1700) -> ()
            n868 = Array Subset(array=w1714, index=w1700, length=w1712) -> (w1706:dbl[])
            n869 = Array Subset(array=w1713, index=w1700, length=w1712) -> (w1705:dbl[])
            n870 = local write "Sat Vg Array-Used"(w1706) -> ()
            n871 = local write "Sat Id-Used"(w1705) -> ()
            n872 = call "Mobility-Vt-Used Pts_Linear.vi"("Width"=w1703, "Length"=w1702, "Dielectric (d)"=w1701, "Sat Id Used"=w1705, "Vg Used"=w1706) -> ("Vt"=w1699:dbl, "Mobility"=w1704:dbl)  [unwired: 4 in, 1 out]
            n873 = Bundle(w1706, w1705) -> (w1710:cluster{dbl[], dbl[]})  [unwired: 1 in]
            n874 = local write "New: VT-Sat"(w1699) -> ()
            n875 = Build Array (concatenate)(w1708, w1707, w1710) -> (w1709:cluster{dbl[], dbl[]}[])
            n876 = local write "New: Mobility-Sat"(w1704) -> ()
            n877 = local write "XY Graph"(w1709) -> ()
          }
          event "Slide 2": Value Change {
            n878 = event-data() -> ()  [unwired: 1 in, 5 out]
            n879 = local read "XY Graph 2"() -> (w1725:cluster{dbl[], dbl[]}[])
            n880 = Decimate 1D Array(w1725) -> (w1722:cluster{dbl[], dbl[]}[], w1721:cluster{dbl[], dbl[]}[])
            n881 = Array To Cluster(array=w1722) -> (cluster=w1730:T9)
            n882 = Unbundle(w1730) -> ("[0]"=w1729:cluster{dbl[], dbl[]})  [unwired: 8 out]
            n883 = local read "NumPts 2"() -> (w1726:dbl)
            n884 = local read "Slide 2"() -> (w1720:dbl)
            n885 = Unbundle(w1729) -> (w1728:dbl[], w1727:dbl[])
            n886 = local write "Index 2"(w1720) -> ()
            n887 = Array Subset(array=w1728, index=w1720, length=w1726) -> (w1718:dbl[])
            n888 = Array Subset(array=w1727, index=w1720, length=w1726) -> (w1717:dbl[])
            n889 = local write "Vg Array-Log-Used"(w1717) -> ()
            n890 = local write "Sat Id-Log-Used"(w1718) -> ()
            n891 = call "STS-Used.vi"("Id Used"=w1718, "Vg-Used"=w1717) -> ("STS"=w1719:dbl)  [unwired: 9 in]
            n892 = Bundle(w1718, w1717) -> (w1724:cluster{dbl[], dbl[]})  [unwired: 1 in]
            n893 = local write "New: STS"(w1719) -> ()
            n894 = Build Array (concatenate)(w1722, w1721, w1724) -> (w1723:cluster{dbl[], dbl[]}[])
            n895 = local write "XY Graph 2"(w1723) -> ()
          }
          event "Save Changes?": Mouse Down {
            n896 = event-data() -> ()  [unwired: 1 in, 5 out]
            n897 = flat-sequence {
              tunnel: [w1758] -> w1735
              tunnel: [w1752] -> w1734
              tunnel: [w1738] -> w1733
              tunnel: w1735 -> [w2057]
              tunnel: w1734 -> [w2054]
              tunnel: [w2055] -> w1732
              tunnel: w1733 -> [w2055]
              tunnel: [w2054] -> w1731
              tunnel: w1732 -> [w2062]
              tunnel: w1731 -> [w2061]
              frame #0 {
                n898 = local read "Transfer File"() -> (w1758:path)
                n899 = local read "New: Temp"() -> (w1739:dbl)
                n900 = local read "New: Length"() -> (w1743:dbl)
                n901 = local read "New: Width"() -> (w1741:dbl)
                n902 = To Single Precision Float(number=w1739) -> (single precision float=w1740:sgl)
                n903 = call-poly <vilib>:"Read From Spreadsheet File.vi"("file path (dialog if empty)"=w1758) -> ("all rows"=w1736:string[][])  [unwired: 6 in, 4 out]
                n904 = Number To Decimal String(number=w1740) -> (decimal integer string=w1755:string)  [unwired: 1 in]
                n905 = To Single Precision Float(number=w1741) -> (single precision float=w1742:sgl)
                n906 = To Single Precision Float(number=w1743) -> (single precision float=w1744:sgl)
                n907 = local read "Index"() -> (w1761:string)
                n908 = Strip Path(path=w1758) -> (stripped path=w1766:path)  [unwired: 1 out]
                n909 = Number To Decimal String(number=w1744) -> (decimal integer string=w1759:string)  [unwired: 1 in]
                n910 = Number To Decimal String(number=w1742) -> (decimal integer string=w1760:string)  [unwired: 1 in]
                n911 = Array Size(array=w1736) -> (size(s)=w1749:i32[])
                n912 = Concatenate Strings("_", w1755, "K") -> (w1753:string)
                n913 = Array Subset(array=w1736, index (row)=0, index (col)=0, length (col)=3) -> (w1745:string[][])  [unwired: 1 in]
                n914 = Index Array(array=w1749, index=0) -> (element=w1751:i32)
                n915 = call "Build Text"("Temp"=w1753, "Index"=w1761, "Length"=w1759, "Width"=w1760) -> ("Result"=w1762:string)  [unwired: 10 in, 1 out]
                n916 = flat-sequence {
                  tunnel: [w2011] -> w1757
                  tunnel: w1757 -> [w2028]
                  frame #0 {
                    # "Makes Empty File for Transformer Data"
                    n917 = local read "Transfer Folder"() -> (w2000:path)
                    n918 = Build Path(base path=w2000, name or relative path="Stats") -> (appended path=w2002:path)
                    n919 = call <vilib>:"Check if File or Folder Exists.vi"("path"=w2002) -> ("file or folder exists?"=w2003:bool, "dup path"=w2004:path)  [unwired: 8 in, 1 out]
                    n920 = case shown="False" w2003 {
                      tunnel: [w2008 w2010] -> w2005
                      tunnel: w2004 -> [w2009 w2010]
                      frame False {
                        n921 = Create Folder(path (use dialog)=w2009) -> (created path=w2008:path)  [unwired: 2 in, 2 out]
                      }
                      frame True {
                      }
                    }
                    n922 = Build Path(base path=w2005, name or relative path="Tranformer Data.txt") -> (appended path=w2007:path)
                    n923 = call-poly <vilib>:"Write To Spreadsheet File.vi"("append to file? (new file:F)"=TRUE, "file path (dialog if empty)"=w2007) -> ()  [unwired: 6 in, 1 out]
                  }
                  frame #1 {
                    # "Adds Headers if they don't exist"
                    n924 = local read "Transfer Folder"() -> (w2017:path)
                    n925 = Concatenate Strings("Stats\\", "Tranformer Data.txt") -> (w2018:string)
                    n926 = Build Path(base path=w2017, name or relative path=w2018) -> (appended path=w2011:path)
                    n927 = call-poly <vilib>:"Read From Spreadsheet File.vi"("file path (dialog if empty)"=w2011) -> ("first row"=w2016:string[])  [unwired: 6 in, 4 out]
                    n928 = Search 1D Array(1D array=w2016, element="DeviceID") -> (index of element=w2014:i32)  [unwired: 1 in]
                    n929 = Equal?(x=w2014, y=0) -> (x = y?=w2012:bool)
                    n930 = case shown="False" w2012 {
                      tunnel: w2011 -> [w2022 _]
                      frame False {
                        n931 = local read "Transformer \nHeaders"() -> (w2021:string[])
                        n932 = call-poly <vilib>:"Write To Spreadsheet File.vi"("1D data"=w2021, "file path (dialog if empty)"=w2022) -> ()  [unwired: 6 in, 1 out]
                      }
                      frame True {
                      }
                    }
                  }
                  frame #2 {
                    # "Adds current device if it doesn't exist"
                    n933 = local read "Current \nRecord"() -> (w2027:string[])
                    n934 = Index Array(array=w2027, index=0) -> (element=w2026:string)
                    n935 = local read "Transfer Folder"() -> (w2030:path)
                    n936 = Concatenate Strings("Stats\\", "Tranformer Data.txt") -> (w2031:string)
                    n937 = local write "Current Device ID"(w2026) -> ()
                    n938 = local read "Current Device ID"() -> (w2036:string)
                    n939 = Build Path(base path=w2030, name or relative path=w2031) -> (appended path=w2029:path)
                    n940 = call-poly <vilib>:"Read From Spreadsheet File.vi"("file path (dialog if empty)"=w2029) -> ("all rows"=w2023:string[][])  [unwired: 6 in, 4 out]
                    n941 = Index Array(array=w2023, index (col)=0) -> (element=w2024:string[])  [unwired: 1 in]
                    n942 = Search 1D Array(1D array=w2024, element=w2036) -> (index of element=w2025:i32)  [unwired: 1 in]
                    n943 = Equal?(x=w2025, y=-1) -> (x = y?=w2038:bool)
                    n944 = case shown="False" w2038 {
                      tunnel: w2028 -> [w2041 w2052]
                      tunnel: w2025 -> [w2044 _]
                      tunnel: w2023 -> [w2045 _]
                      frame False {
                        n945 = local read "Current \nRecord"() -> (w2043:string[])
                        n946 = Replace Array Subset(array=w2045, new element=w2043, index (row)=w2044) -> (w2042:string[][])  [unwired: 1 in]
                        n947 = flat-sequence {
                          tunnel: w2041 -> [w2046]
                          tunnel: w2042 -> [w2047]
                          tunnel: [w2047] -> w2040
                          tunnel: [w2046] -> w2039
                          tunnel: w2040 -> [w2049]
                          tunnel: w2039 -> [w2048]
                          frame #0 {
                            n948 = Delete(path (use dialog)=w2046) -> ()  [unwired: 4 in, 3 out]
                          }
                          frame #1 {
                            n949 = call-poly <vilib>:"Write To Spreadsheet File.vi"("append to file? (new file:F)"=TRUE, "2D data"=w2049, "file path (dialog if empty)"=w2048) -> ()  [unwired: 5 in, 1 out]
                          }
                        }
                      }
                      frame True {
                        n950 = local read "Current \nRecord"() -> (w2051:string[])
                        n951 = call-poly <vilib>:"Write To Spreadsheet File.vi"("append to file? (new file:F)"=TRUE, "1D data"=w2051, "file path (dialog if empty)"=w2052) -> ()  [unwired: 5 in, 1 out]
                      }
                    }
                  }
                }
                n952 = Reshape Array(w1745, w1751) -> (w1737:string[])
                n953 = Path To String(path=w1766) -> (string=w1764:string)
                n954 = stacked-sequence {
                  tunnel: w1737 -> [w1773 w1786 w1804 w1822 w1840 w1858 w1874 w1894 w1912 w1929 w1947 w1965 w1983]
                  tunnel: [_ _ _ _ _ _ _ _ _ _ _ _ w1981] -> w1738
                  frame #0 {
                    n955 = Search 1D Array(1D array=w1773, element="Dielectric (nm):") -> (index of element=w1770:i32)  [unwired: 1 in]
                    n956 = Equal?(x=w1770, y=-1) -> (x = y?=w1769:bool)
                    n957 = local read "Save1 Array"() -> (w1768:string[][])
                    n958 = case shown="False" w1769 {
                      tunnel: w1768 -> [w1779 w1783]
                      tunnel: w1770 -> [w1775 _]
                      tunnel: [w1774 w1783] -> w1767
                      frame False {
                        n959 = local read "New: Dielectric"() -> (w1781:dbl)
                        n960 = Number To Fractional String(number=w1781) -> (F-format string=w1776:string)  [unwired: 3 in]
                        n961 = Divide(x=w1775, y=3) -> (x/y=w1778:dbl)
                        n962 = To Word Integer(number=w1778) -> (16bit integer=w1777:i16)
                        n963 = Replace Array Subset(array=w1779, new element=w1776, index (row)=w1777, index (col)=1) -> (w1774:string[][])
                      }
                      frame True {
                      }
                    }
                    n964 = local write "Save1 Array"(w1767) -> ()
                  }
                  frame #1 {
                    n965 = Search 1D Array(1D array=w1786, element="Length (um):") -> (index of element=w1788:i32)  [unwired: 1 in]
                    n966 = Equal?(x=w1788, y=-1) -> (x = y?=w1787:bool)
                    n967 = local read "Save1 Array"() -> (w1785:string[][])
                    n968 = case shown="False" w1787 {
                      tunnel: w1785 -> [w1798 w1801]
                      tunnel: w1788 -> [w1795 _]
                      tunnel: [w1794 w1801] -> w1784
                      frame False {
                        n969 = local read "New: Length"() -> (w1791:dbl)
                        n970 = Divide(x=w1795, y=3) -> (x/y=w1797:dbl)
                        n971 = Format Value(format string="%#g", value (0)=w1791) -> (output string=w1792:string)  [unwired: 1 in]
                        n972 = To Word Integer(number=w1797) -> (16bit integer=w1796:i16)
                        n973 = Replace Array Subset(array=w1798, new element=w1792, index (row)=w1796, index (col)=1) -> (w1794:string[][])
                      }
                      frame True {
                      }
                    }
                    n974 = local write "Save1 Array"(w1784) -> ()
                  }
                  frame #2 {
                    n975 = Search 1D Array(1D array=w1804, element="Width (um):") -> (index of element=w1806:i32)  [unwired: 1 in]
                    n976 = Equal?(x=w1806, y=-1) -> (x = y?=w1805:bool)
                    n977 = local read "Save1 Array"() -> (w1803:string[][])
                    n978 = case shown="False" w1805 {
                      tunnel: w1806 -> [w1814 _]
                      tunnel: w1803 -> [w1813 w1819]
                      tunnel: [w1812 w1819] -> w1802
                      frame False {
                        n979 = local read "New: Width"() -> (w1809:dbl)
                        n980 = Divide(x=w1814, y=3) -> (x/y=w1816:dbl)
                        n981 = To Word Integer(number=w1816) -> (16bit integer=w1815:i16)
                        n982 = Format Value(format string="%#g", value (0)=w1809) -> (output string=w1810:string)  [unwired: 1 in]
                        n983 = Replace Array Subset(array=w1813, new element=w1810, index (row)=w1815, index (col)=1) -> (w1812:string[][])
                      }
                      frame True {
                      }
                    }
                    n984 = local write "Save1 Array"(w1802) -> ()
                  }
                  frame #3 {
                    n985 = Search 1D Array(1D array=w1822, element="Sample Temp (K):") -> (index of element=w1824:i32)  [unwired: 1 in]
                    n986 = Equal?(x=w1824, y=-1) -> (x = y?=w1823:bool)
                    n987 = local read "Save1 Array"() -> (w1821:string[][])
                    n988 = case shown="False" w1823 {
                      tunnel: w1821 -> [w1834 w1837]
                      tunnel: w1824 -> [w1831 _]
                      tunnel: [w1830 w1837] -> w1820
                      frame False {
                        n989 = local read "New: Temp"() -> (w1828:dbl)
                        n990 = Divide(x=w1831, y=3) -> (x/y=w1833:dbl)
                        n991 = Format Value(format string="%#g", value (0)=w1828) -> (output string=w1827:string)  [unwired: 1 in]
                        n992 = To Word Integer(number=w1833) -> (16bit integer=w1832:i16)
                        n993 = Replace Array Subset(array=w1834, new element=w1827, index (row)=w1832, index (col)=1) -> (w1830:string[][])
                      }
                      frame True {
                      }
                    }
                    n994 = local write "Save1 Array"(w1820) -> ()
                  }
                  frame #4 {
                    n995 = Search 1D Array(1D array=w1840, element="Mobility-Sat (cm^2/Vs):") -> (index of element=w1842:i32)  [unwired: 1 in]
                    n996 = Equal?(x=w1842, y=-1) -> (x = y?=w1841:bool)
                    n997 = local read "Save1 Array"() -> (w1838:string[][])
                    n998 = case shown="False" w1841 {
                      tunnel: w1838 -> [w1852 w1855]
                      tunnel: w1842 -> [w1849 _]
                      tunnel: [w1848 w1855] -> w1839
                      frame False {
                        n999 = local read "New: Mobility-Sat"() -> (w1845:dbl)
                        n1000 = Divide(x=w1849, y=3) -> (x/y=w1851:dbl)
                        n1001 = To Word Integer(number=w1851) -> (16bit integer=w1850:i16)
                        n1002 = Format Value(format string="%#g", value (0)=w1845) -> (output string=w1846:string)  [unwired: 1 in]
                        n1003 = Replace Array Subset(array=w1852, new element=w1846, index (row)=w1850, index (col)=1) -> (w1848:string[][])
                      }
                      frame True {
                      }
                    }
                    n1004 = local write "Save1 Array"(w1839) -> ()
                  }
                  frame #5 {
                    n1005 = Search 1D Array(1D array=w1858, element="On/Off I-Sat:") -> (index of element=w1860:i32)  [unwired: 1 in]
                    n1006 = Equal?(x=w1860, y=-1) -> (x = y?=w1859:bool)
                    n1007 = local read "Save1 Array"() -> (w1857:string[][])
                    n1008 = case shown="False" w1859 {
                      tunnel: w1857 -> [w1870 w1873]
                      tunnel: w1860 -> [w1867 _]
                      tunnel: [w1866 w1873] -> w1856
                      frame False {
                        n1009 = local read "Calc: On/Off"() -> (w1863:dbl)
                        n1010 = Divide(x=w1867, y=3) -> (x/y=w1869:dbl)
                        n1011 = To Word Integer(number=w1869) -> (16bit integer=w1868:i16)
                        n1012 = Format Value(format string="%#g", value (0)=w1863) -> (output string=w1864:string)  [unwired: 1 in]
                        n1013 = Replace Array Subset(array=w1870, new element=w1864, index (row)=w1868, index (col)=1) -> (w1866:string[][])
                      }
                      frame True {
                      }
                    }
                    n1014 = local write "Save1 Array"(w1856) -> ()
                  }
                  frame #6 {
                    n1015 = Search 1D Array(1D array=w1874, element="Mobility-Lin (cm^2/Vs):") -> (index of element=w1878:i32)  [unwired: 1 in]
                    n1016 = Equal?(x=w1878, y=-1) -> (x = y?=w1877:bool)
                    n1017 = local read "Save1 Array"() -> (w1876:string[][])
                    n1018 = case shown="False" w1877 {
                      tunnel: w1876 -> [w1888 w1891]
                      tunnel: w1878 -> [w1885 _]
                      tunnel: [w1884 w1891] -> w1875
                      frame False {
                        n1019 = local read "Calc: Mobility-Lin"() -> (w1881:dbl)
                        n1020 = Divide(x=w1885, y=3) -> (x/y=w1887:dbl)
                        n1021 = To Word Integer(number=w1887) -> (16bit integer=w1886:i16)
                        n1022 = Format Value(format string="%#g", value (0)=w1881) -> (output string=w1882:string)  [unwired: 1 in]
                        n1023 = Replace Array Subset(array=w1888, new element=w1882, index (row)=w1886, index (col)=1) -> (w1884:string[][])
                      }
                      frame True {
                      }
                    }
                    n1024 = local write "Save1 Array"(w1875) -> ()
                  }
                  frame #7 {
                    n1025 = Search 1D Array(1D array=w1894, element="Off I-Sat (A):") -> (index of element=w1896:i32)  [unwired: 1 in]
                    n1026 = Equal?(x=w1896, y=-1) -> (x = y?=w1895:bool)
                    n1027 = local read "Save1 Array"() -> (w1893:string[][])
                    n1028 = case shown="False" w1895 {
                      tunnel: w1893 -> [w1906 w1909]
                      tunnel: w1896 -> [w1903 _]
                      tunnel: [w1902 w1909] -> w1892
                      frame False {
                        n1029 = local read "Calc: Off I-Sat"() -> (w1901:dbl)
                        n1030 = Divide(x=w1903, y=3) -> (x/y=w1905:dbl)
                        n1031 = Format Value(format string="%#g", value (0)=w1901) -> (output string=w1899:string)  [unwired: 1 in]
                        n1032 = To Word Integer(number=w1905) -> (16bit integer=w1904:i16)
                        n1033 = Replace Array Subset(array=w1906, new element=w1899, index (row)=w1904, index (col)=1) -> (w1902:string[][])
                      }
                      frame True {
                      }
                    }
                    n1034 = local write "Save1 Array"(w1892) -> ()
                  }
                  frame #8 {
                    n1035 = Search 1D Array(1D array=w1912, element="Vt-Sat (V):") -> (index of element=w1914:i32)  [unwired: 1 in]
                    n1036 = Equal?(x=w1914, y=-1) -> (x = y?=w1913:bool)
                    n1037 = local read "Save1 Array"() -> (w1911:string[][])
                    n1038 = case shown="False" w1913 {
                      tunnel: w1911 -> [w1922 w1926]
                      tunnel: w1914 -> [w1918 _]
                      tunnel: [w1917 w1926] -> w1910
                      frame False {
                        n1039 = local read "New: VT-Sat"() -> (w1924:dbl)
                        n1040 = Number To Fractional String(number=w1924) -> (F-format string=w1919:string)  [unwired: 3 in]
                        n1041 = Divide(x=w1918, y=3) -> (x/y=w1921:dbl)
                        n1042 = To Word Integer(number=w1921) -> (16bit integer=w1920:i16)
                        n1043 = Replace Array Subset(array=w1922, new element=w1919, index (row)=w1920, index (col)=1) -> (w1917:string[][])
                      }
                      frame True {
                      }
                    }
                    n1044 = local write "Save1 Array"(w1910) -> ()
                  }
                  frame #9 {
                    n1045 = Search 1D Array(1D array=w1929, element="VT-Lin (V):") -> (index of element=w1931:i32)  [unwired: 1 in]
                    n1046 = Equal?(x=w1931, y=-1) -> (x = y?=w1930:bool)
                    n1047 = local read "Save1 Array"() -> (w1928:string[][])
                    n1048 = case shown="False" w1930 {
                      tunnel: w1928 -> [w1941 w1944]
                      tunnel: w1931 -> [w1938 _]
                      tunnel: [w1937 w1944] -> w1927
                      frame False {
                        n1049 = local read "New: VT-Lin"() -> (w1935:dbl)
                        n1050 = Divide(x=w1938, y=3) -> (x/y=w1940:dbl)
                        n1051 = Format Value(format string="%#g", value (0)=w1935) -> (output string=w1934:string)  [unwired: 1 in]
                        n1052 = To Word Integer(number=w1940) -> (16bit integer=w1939:i16)
                        n1053 = Replace Array Subset(array=w1941, new element=w1934, index (row)=w1939, index (col)=1) -> (w1937:string[][])
                      }
                      frame True {
                      }
                    }
                    n1054 = local write "Save1 Array"(w1927) -> ()
                  }
                  frame #10 {
                    n1055 = Search 1D Array(1D array=w1947, element="STS-Sat (V/decade):") -> (index of element=w1949:i32)  [unwired: 1 in]
                    n1056 = Equal?(x=w1949, y=-1) -> (x = y?=w1948:bool)
                    n1057 = local read "Save1 Array"() -> (w1946:string[][])
                    n1058 = case shown="False" w1948 {
                      tunnel: w1946 -> [w1959 w1962]
                      tunnel: w1949 -> [w1956 _]
                      tunnel: [w1955 w1962] -> w1945
                      frame False {
                        n1059 = local read "New: STS"() -> (w1953:dbl)
                        n1060 = Divide(x=w1956, y=3) -> (x/y=w1958:dbl)
                        n1061 = Format Value(format string="%#g", value (0)=w1953) -> (output string=w1952:string)  [unwired: 1 in]
                        n1062 = To Word Integer(number=w1958) -> (16bit integer=w1957:i16)
                        n1063 = Replace Array Subset(array=w1959, new element=w1952, index (row)=w1957, index (col)=1) -> (w1955:string[][])
                      }
                      frame True {
                      }
                    }
                    n1064 = local write "Save1 Array"(w1945) -> ()
                  }
                  frame #11 {
                    n1065 = Search 1D Array(1D array=w1965, element="Trap Density-VT (Traps/Vcm^2):") -> (index of element=w1967:i32)  [unwired: 1 in]
                    n1066 = Equal?(x=w1967, y=-1) -> (x = y?=w1966:bool)
                    n1067 = local read "Save1 Array"() -> (w1964:string[][])
                    n1068 = case shown="False" w1966 {
                      tunnel: w1964 -> [w1977 w1980]
                      tunnel: w1967 -> [w1973 _]
                      tunnel: [w1972 w1980] -> w1963
                      frame False {
                        n1069 = local read "New: Trap Density-VT"() -> (w1971:dbl)
                        n1070 = Format Value(format string="%#g", value (0)=w1971) -> (output string=w1974:string)  [unwired: 1 in]
                        n1071 = Divide(x=w1973, y=3) -> (x/y=w1976:dbl)
                        n1072 = To Word Integer(number=w1976) -> (16bit integer=w1975:i16)
                        n1073 = Replace Array Subset(array=w1977, new element=w1974, index (row)=w1975, index (col)=1) -> (w1972:string[][])
                      }
                      frame True {
                      }
                    }
                    n1074 = local write "Save1 Array"(w1963) -> ()
                  }
                  frame #12 {
                    n1075 = Search 1D Array(1D array=w1983, element="Trap Density-STS (Traps/Vcm^2):") -> (index of element=w1985:i32)  [unwired: 1 in]
                    n1076 = Equal?(x=w1985, y=-1) -> (x = y?=w1984:bool)
                    n1077 = local read "Save1 Array"() -> (w1982:string[][])
                    n1078 = case shown="False" w1984 {
                      tunnel: w1982 -> [w1995 w1998]
                      tunnel: w1985 -> [w1992 _]
                      tunnel: [w1991 w1998] -> w1981
                      frame False {
                        n1079 = local read "New: Trap Density-STS"() -> (w1989:dbl)
                        n1080 = Divide(x=w1992, y=3) -> (x/y=w1994:dbl)
                        n1081 = To Word Integer(number=w1994) -> (16bit integer=w1993:i16)
                        n1082 = Format Value(format string="%#g", value (0)=w1989) -> (output string=w1988:string)  [unwired: 1 in]
                        n1083 = Replace Array Subset(array=w1995, new element=w1988, index (row)=w1993, index (col)=1) -> (w1991:string[][])
                      }
                      frame True {
                      }
                    }
                    n1084 = local write "Save1 Array"(w1981) -> ()
                  }
                }
                n1085 = Concatenate Strings(w1764, "\\", w1762) -> (w1763:string)
                n1086 = String To Path(string=w1763) -> (path=w1752:path)
                n1087 = local write "Save1 Array"(w1736) -> ()
              }
              frame #1 {
                n1088 = Equal?(x=w2057, y=w2054) -> (x = y?=w2056:bool)
                n1089 = case shown="False" w2056 {
                  tunnel: w2057 -> [w2060 _]
                  tunnel: w2054 -> [w2059 _]
                  frame False {
                    n1090 = Move(source path=w2060, 9:TRUE, 10:w2059) -> ()  [unwired: 2 in, 3 out]
                  }
                  frame True {
                  }
                }
              }
              frame #2 {
                n1091 = local write "Transfer File"(w2061) -> ()
                n1092 = call-poly <vilib>:"Write To Spreadsheet File.vi"("2D data"=w2062, "file path (dialog if empty)"=w2061) -> ()  [unwired: 6 in, 1 out]
              }
            }
          }
          event "Save Changes? 2": Mouse Down {
            n1093 = event-data() -> ()  [unwired: 1 in, 5 out]
            n1094 = stacked-sequence {
              seq-local: [w2122 _ _ _ _] -> [_ w2374 _ _ _]
              seq-local: [w2125 _ _ _ _] -> [_ w2375 _ _ _]
              seq-local: [w2122 _ _ _ _] -> [_ w2373 _ _ _]
              seq-local: [w2120 _ _ _ _] -> [_ w2371 _ _ _]
              seq-local: [_ w2375 _ _ _] -> [_ _ w2380 _ _]
              seq-local: [_ w2371 _ _ _] -> [_ _ w2379 _ _]
              frame #0 {
                n1095 = local read "Transfer File"() -> (w2125:path)
                n1096 = local read "New: Temp"() -> (w2124:dbl)
                n1097 = local read "New: Length"() -> (w2128:dbl)
                n1098 = local read "New: Width"() -> (w2126:dbl)
                n1099 = To Word Integer(number=w2124) -> (16bit integer=w2123:i16)
                n1100 = call-poly <vilib>:"Read From Spreadsheet File.vi"("file path (dialog if empty)"=w2125) -> ("all rows"=w2119:string[][])  [unwired: 6 in, 4 out]
                n1101 = Number To Decimal String(number=w2123) -> (decimal integer string=w2139:string)  [unwired: 1 in]
                n1102 = To Single Precision Float(number=w2126) -> (single precision float=w2127:sgl)
                n1103 = To Single Precision Float(number=w2128) -> (single precision float=w2129:sgl)
                n1104 = local read "Index"() -> (w2143:string)
                n1105 = Strip Path(path=w2125) -> (stripped path=w2148:path)  [unwired: 1 out]
                n1106 = Number To Decimal String(number=w2129) -> (decimal integer string=w2141:string)  [unwired: 1 in]
                n1107 = Number To Decimal String(number=w2127) -> (decimal integer string=w2142:string)  [unwired: 1 in]
                n1108 = Array Size(array=w2119) -> (size(s)=w2134:i32[])
                n1109 = Concatenate Strings("_", w2139, "K") -> (w2137:string)
                n1110 = Array Subset(array=w2119, index (row)=0, index (col)=0, length (col)=3) -> (w2130:string[][])  [unwired: 1 in]
                n1111 = Index Array(array=w2134, index=0) -> (element=w2136:i32)
                n1112 = call "Build Text2"("Temp"=w2137, "Index"=w2143, "Length"=w2141, "Width"=w2142) -> ("Result"=w2144:string)  [unwired: 10 in, 1 out]
                n1113 = Reshape Array(w2130, w2136) -> (w2121:string[])
                n1114 = Path To String(path=w2148) -> (string=w2146:string)
                n1115 = stacked-sequence {
                  tunnel: w2121 -> [w2155 w2168 w2185 w2202 w2219 w2236 w2251 w2270 w2288 w2305 w2322 w2339 w2356]
                  tunnel: [_ _ _ _ _ _ _ _ _ _ _ _ w2354] -> w2120
                  frame #0 {
                    n1116 = Search 1D Array(1D array=w2155, element="Dielectric (nm):") -> (index of element=w2152:i32)  [unwired: 1 in]
                    n1117 = Equal?(x=w2152, y=-1) -> (x = y?=w2151:bool)
                    n1118 = local read "Save1 Array"() -> (w2150:string[][])
                    n1119 = case shown="False" w2151 {
                      tunnel: w2150 -> [w2161 w2165]
                      tunnel: w2152 -> [w2157 _]
                      tunnel: [w2156 w2165] -> w2149
                      frame False {
                        n1120 = local read "New: Dielectric"() -> (w2163:dbl)
                        n1121 = Number To Fractional String(number=w2163) -> (F-format string=w2158:string)  [unwired: 3 in]
                        n1122 = Divide(x=w2157, y=3) -> (x/y=w2160:dbl)
                        n1123 = To Word Integer(number=w2160) -> (16bit integer=w2159:i16)
                        n1124 = Replace Array Subset(array=w2161, new element=w2158, index (row)=w2159, index (col)=1) -> (w2156:string[][])
                      }
                      frame True {
                      }
                    }
                    n1125 = local write "Save1 Array"(w2149) -> ()
                  }
                  frame #1 {
                    n1126 = Search 1D Array(1D array=w2168, element="Length (um):") -> (index of element=w2170:i32)  [unwired: 1 in]
                    n1127 = Equal?(x=w2170, y=-1) -> (x = y?=w2169:bool)
                    n1128 = local read "Save1 Array"() -> (w2167:string[][])
                    n1129 = case shown="True" w2169 {
                      tunnel: w2167 -> [w2178 w2182]
                      tunnel: w2170 -> [w2174 _]
                      tunnel: [w2173 w2182] -> w2166
                      frame False {
                        n1130 = local read "New: Length"() -> (w2180:dbl)
                        n1131 = Number To Fractional String(number=w2180) -> (F-format string=w2175:string)  [unwired: 3 in]
                        n1132 = Divide(x=w2174, y=3) -> (x/y=w2177:dbl)
                        n1133 = To Word Integer(number=w2177) -> (16bit integer=w2176:i16)
                        n1134 = Replace Array Subset(array=w2178, new element=w2175, index (row)=w2176, index (col)=1) -> (w2173:string[][])
                      }
                      frame True {
                      }
                    }
                    n1135 = local write "Save1 Array"(w2166) -> ()
                  }
                  frame #2 {
                    n1136 = Search 1D Array(1D array=w2185, element="Width (um):") -> (index of element=w2187:i32)  [unwired: 1 in]
                    n1137 = Equal?(x=w2187, y=-1) -> (x = y?=w2186:bool)
                    n1138 = local read "Save1 Array"() -> (w2184:string[][])
                    n1139 = case shown="False" w2186 {
                      tunnel: w2187 -> [w2192 _]
                      tunnel: w2184 -> [w2191 w2199]
                      tunnel: [w2190 w2199] -> w2183
                      frame False {
                        n1140 = local read "New: Width"() -> (w2197:dbl)
                        n1141 = Number To Fractional String(number=w2197) -> (F-format string=w2193:string)  [unwired: 3 in]
                        n1142 = Divide(x=w2192, y=3) -> (x/y=w2195:dbl)
                        n1143 = To Word Integer(number=w2195) -> (16bit integer=w2194:i16)
                        n1144 = Replace Array Subset(array=w2191, new element=w2193, index (row)=w2194, index (col)=1) -> (w2190:string[][])
                      }
                      frame True {
                      }
                    }
                    n1145 = local write "Save1 Array"(w2183) -> ()
                  }
                  frame #3 {
                    n1146 = Search 1D Array(1D array=w2202, element="Sample Temp (K):") -> (index of element=w2204:i32)  [unwired: 1 in]
                    n1147 = Equal?(x=w2204, y=-1) -> (x = y?=w2203:bool)
                    n1148 = local read "Save1 Array"() -> (w2201:string[][])
                    n1149 = case shown="False" w2203 {
                      tunnel: w2201 -> [w2212 w2216]
                      tunnel: w2204 -> [w2208 _]
                      tunnel: [w2207 w2216] -> w2200
                      frame False {
                        n1150 = local read "New: Temp"() -> (w2214:dbl)
                        n1151 = Number To Fractional String(number=w2214) -> (F-format string=w2209:string)  [unwired: 3 in]
                        n1152 = Divide(x=w2208, y=3) -> (x/y=w2211:dbl)
                        n1153 = To Word Integer(number=w2211) -> (16bit integer=w2210:i16)
                        n1154 = Replace Array Subset(array=w2212, new element=w2209, index (row)=w2210, index (col)=1) -> (w2207:string[][])
                      }
                      frame True {
                      }
                    }
                    n1155 = local write "Save1 Array"(w2200) -> ()
                  }
                  frame #4 {
                    n1156 = Search 1D Array(1D array=w2219, element="Mobility-Sat (cm^2/Vs):") -> (index of element=w2221:i32)  [unwired: 1 in]
                    n1157 = Equal?(x=w2221, y=-1) -> (x = y?=w2220:bool)
                    n1158 = local read "Save1 Array"() -> (w2217:string[][])
                    n1159 = case shown="False" w2220 {
                      tunnel: w2217 -> [w2229 w2233]
                      tunnel: w2221 -> [w2225 _]
                      tunnel: [w2224 w2233] -> w2218
                      frame False {
                        n1160 = local read "New: Mobility-Sat"() -> (w2231:dbl)
                        n1161 = Number To Fractional String(number=w2231) -> (F-format string=w2226:string)  [unwired: 3 in]
                        n1162 = Divide(x=w2225, y=3) -> (x/y=w2228:dbl)
                        n1163 = To Word Integer(number=w2228) -> (16bit integer=w2227:i16)
                        n1164 = Replace Array Subset(array=w2229, new element=w2226, index (row)=w2227, index (col)=1) -> (w2224:string[][])
                      }
                      frame True {
                      }
                    }
                    n1165 = local write "Save1 Array"(w2218) -> ()
                  }
                  frame #5 {
                    n1166 = Search 1D Array(1D array=w2236, element="Mobility-Lin (cm^2/Vs):") -> (index of element=w2238:i32)  [unwired: 1 in]
                    n1167 = Equal?(x=w2238, y=-1) -> (x = y?=w2237:bool)
                    n1168 = local read "Save1 Array"() -> (w2235:string[][])
                    n1169 = case shown="False" w2237 {
                      tunnel: w2235 -> [w2246 w2250]
                      tunnel: w2238 -> [w2242 _]
                      tunnel: [w2241 w2250] -> w2234
                      frame False {
                        n1170 = local read "Calc: Mobility-Lin"() -> (w2248:dbl)
                        n1171 = Number To Fractional String(number=w2248) -> (F-format string=w2243:string)  [unwired: 3 in]
                        n1172 = Divide(x=w2242, y=3) -> (x/y=w2245:dbl)
                        n1173 = To Word Integer(number=w2245) -> (16bit integer=w2244:i16)
                        n1174 = Replace Array Subset(array=w2246, new element=w2243, index (row)=w2244, index (col)=1) -> (w2241:string[][])
                      }
                      frame True {
                      }
                    }
                    n1175 = local write "Save1 Array"(w2234) -> ()
                  }
                  frame #6 {
                    n1176 = Search 1D Array(1D array=w2251, element="On/Off I-Sat:") -> (index of element=w2255:i32)  [unwired: 1 in]
                    n1177 = Equal?(x=w2255, y=-1) -> (x = y?=w2254:bool)
                    n1178 = local read "Save1 Array"() -> (w2253:string[][])
                    n1179 = case shown="False" w2254 {
                      tunnel: w2253 -> [w2263 w2267]
                      tunnel: w2255 -> [w2259 _]
                      tunnel: [w2258 w2267] -> w2252
                      frame False {
                        n1180 = local read "Calc: On/Off"() -> (w2265:dbl)
                        n1181 = Number To Fractional String(number=w2265) -> (F-format string=w2260:string)  [unwired: 3 in]
                        n1182 = Divide(x=w2259, y=3) -> (x/y=w2262:dbl)
                        n1183 = To Word Integer(number=w2262) -> (16bit integer=w2261:i16)
                        n1184 = Replace Array Subset(array=w2263, new element=w2260, index (row)=w2261, index (col)=1) -> (w2258:string[][])
                      }
                      frame True {
                      }
                    }
                    n1185 = local write "Save1 Array"(w2252) -> ()
                  }
                  frame #7 {
                    n1186 = Search 1D Array(1D array=w2270, element="Off I-Sat (A):") -> (index of element=w2272:i32)  [unwired: 1 in]
                    n1187 = Equal?(x=w2272, y=-1) -> (x = y?=w2271:bool)
                    n1188 = local read "Save1 Array"() -> (w2269:string[][])
                    n1189 = case shown="False" w2271 {
                      tunnel: w2269 -> [w2282 w2285]
                      tunnel: w2272 -> [w2279 _]
                      tunnel: [w2278 w2285] -> w2268
                      frame False {
                        n1190 = local read "Calc: Off I-Sat"() -> (w2277:dbl)
                        n1191 = Format Value(format string="%#g", value (0)=w2277) -> (output string=w2276:string)  [unwired: 1 in]
                        n1192 = Divide(x=w2279, y=3) -> (x/y=w2281:dbl)
                        n1193 = To Word Integer(number=w2281) -> (16bit integer=w2280:i16)
                        n1194 = Replace Array Subset(array=w2282, new element=w2276, index (row)=w2280, index (col)=1) -> (w2278:string[][])
                      }
                      frame True {
                      }
                    }
                    n1195 = local write "Save1 Array"(w2268) -> ()
                  }
                  frame #8 {
                    n1196 = Search 1D Array(1D array=w2288, element="Vt-Sat (V):") -> (index of element=w2290:i32)  [unwired: 1 in]
                    n1197 = Equal?(x=w2290, y=-1) -> (x = y?=w2289:bool)
                    n1198 = local read "Save1 Array"() -> (w2287:string[][])
                    n1199 = case shown="False" w2289 {
                      tunnel: w2287 -> [w2298 w2302]
                      tunnel: w2290 -> [w2294 _]
                      tunnel: [w2293 w2302] -> w2286
                      frame False {
                        n1200 = local read "New: VT-Sat"() -> (w2300:dbl)
                        n1201 = Number To Fractional String(number=w2300) -> (F-format string=w2295:string)  [unwired: 3 in]
                        n1202 = Divide(x=w2294, y=3) -> (x/y=w2297:dbl)
                        n1203 = To Word Integer(number=w2297) -> (16bit integer=w2296:i16)
                        n1204 = Replace Array Subset(array=w2298, new element=w2295, index (row)=w2296, index (col)=1) -> (w2293:string[][])
                      }
                      frame True {
                      }
                    }
                    n1205 = local write "Save1 Array"(w2286) -> ()
                  }
                  frame #9 {
                    n1206 = Search 1D Array(1D array=w2305, element="VT-Lin (V):") -> (index of element=w2307:i32)  [unwired: 1 in]
                    n1207 = Equal?(x=w2307, y=-1) -> (x = y?=w2306:bool)
                    n1208 = local read "Save1 Array"() -> (w2304:string[][])
                    n1209 = case shown="True" w2306 {
                      tunnel: w2304 -> [w2315 w2319]
                      tunnel: w2307 -> [w2311 _]
                      tunnel: [w2310 w2319] -> w2303
                      frame False {
                        n1210 = local read "New: VT-Lin"() -> (w2317:dbl)
                        n1211 = Number To Fractional String(number=w2317) -> (F-format string=w2312:string)  [unwired: 3 in]
                        n1212 = Divide(x=w2311, y=3) -> (x/y=w2314:dbl)
                        n1213 = To Word Integer(number=w2314) -> (16bit integer=w2313:i16)
                        n1214 = Replace Array Subset(array=w2315, new element=w2312, index (row)=w2313, index (col)=1) -> (w2310:string[][])
                      }
                      frame True {
                      }
                    }
                    n1215 = local write "Save1 Array"(w2303) -> ()
                  }
                  frame #10 {
                    n1216 = Search 1D Array(1D array=w2322, element="STS-Sat (V/decade):") -> (index of element=w2324:i32)  [unwired: 1 in]
                    n1217 = Equal?(x=w2324, y=-1) -> (x = y?=w2323:bool)
                    n1218 = local read "Save1 Array"() -> (w2321:string[][])
                    n1219 = case shown="False" w2323 {
                      tunnel: w2321 -> [w2332 w2336]
                      tunnel: w2324 -> [w2328 _]
                      tunnel: [w2327 w2336] -> w2320
                      frame False {
                        n1220 = local read "New: STS"() -> (w2334:dbl)
                        n1221 = Number To Fractional String(number=w2334) -> (F-format string=w2329:string)  [unwired: 3 in]
                        n1222 = Divide(x=w2328, y=3) -> (x/y=w2331:dbl)
                        n1223 = To Word Integer(number=w2331) -> (16bit integer=w2330:i16)
                        n1224 = Replace Array Subset(array=w2332, new element=w2329, index (row)=w2330, index (col)=1) -> (w2327:string[][])
                      }
                      frame True {
                      }
                    }
                    n1225 = local write "Save1 Array"(w2320) -> ()
                  }
                  frame #11 {
                    n1226 = Search 1D Array(1D array=w2339, element="Trap Density-VT (Traps/Vcm^2):") -> (index of element=w2341:i32)  [unwired: 1 in]
                    n1227 = Equal?(x=w2341, y=-1) -> (x = y?=w2340:bool)
                    n1228 = local read "Save1 Array"() -> (w2338:string[][])
                    n1229 = case shown="False" w2340 {
                      tunnel: w2338 -> [w2349 w2353]
                      tunnel: w2341 -> [w2345 _]
                      tunnel: [w2344 w2353] -> w2337
                      frame False {
                        n1230 = local read "New: Trap Density-VT"() -> (w2351:dbl)
                        n1231 = Number To Fractional String(number=w2351) -> (F-format string=w2346:string)  [unwired: 3 in]
                        n1232 = Divide(x=w2345, y=3) -> (x/y=w2348:dbl)
                        n1233 = To Word Integer(number=w2348) -> (16bit integer=w2347:i16)
                        n1234 = Replace Array Subset(array=w2349, new element=w2346, index (row)=w2347, index (col)=1) -> (w2344:string[][])
                      }
                      frame True {
                      }
                    }
                    n1235 = local write "Save1 Array"(w2337) -> ()
                  }
                  frame #12 {
                    n1236 = Search 1D Array(1D array=w2356, element="Trap Density-STS (Traps/Vcm^2):") -> (index of element=w2358:i32)  [unwired: 1 in]
                    n1237 = Equal?(x=w2358, y=-1) -> (x = y?=w2357:bool)
                    n1238 = local read "Save1 Array"() -> (w2355:string[][])
                    n1239 = case shown="False" w2357 {
                      tunnel: w2355 -> [w2366 w2370]
                      tunnel: w2358 -> [w2362 _]
                      tunnel: [w2361 w2370] -> w2354
                      frame False {
                        n1240 = local read "New: Trap Density-STS"() -> (w2368:dbl)
                        n1241 = Number To Fractional String(number=w2368) -> (F-format string=w2363:string)  [unwired: 3 in]
                        n1242 = Divide(x=w2362, y=3) -> (x/y=w2365:dbl)
                        n1243 = To Word Integer(number=w2365) -> (16bit integer=w2364:i16)
                        n1244 = Replace Array Subset(array=w2366, new element=w2363, index (row)=w2364, index (col)=1) -> (w2361:string[][])
                      }
                      frame True {
                      }
                    }
                    n1245 = local write "Save1 Array"(w2354) -> ()
                  }
                }
                n1246 = Concatenate Strings(w2146, "\\", w2144) -> (w2145:string)
                n1247 = String To Path(string=w2145) -> (path=w2122:path)
                "No Image 2" <- w2122
                n1248 = local write "Save1 Array"(w2119) -> ()
              }
              frame #1 {
                n1249 = Equal?(x=w2374, y=w2373) -> (x = y?=w2372:bool)
                n1250 = case shown="False" w2372 {
                  tunnel: w2374 -> [w2378 _]
                  tunnel: w2373 -> [w2377 _]
                  frame False {
                    n1251 = Move(source path=w2378, 9:TRUE, 10:w2377) -> ()  [unwired: 2 in, 3 out]
                  }
                  frame True {
                  }
                }
              }
              frame #2 {
                n1252 = local write "Transfer File"(w2380) -> ()
                n1253 = call-poly <vilib>:"Write To Spreadsheet File.vi"("2D data"=w2379, "file path (dialog if empty)"=w2380) -> ()  [unwired: 6 in, 1 out]
              }
              frame #3 {
                w2480 = 0
                # "Moves to next file and displays new image/data"
                n1254 = property on="Image Out" class="ImageControl"() -> (error out=w2442:errorcluster, "Image Center Position"=w2446:cluster{"X":u32, "Y":u32})  [unwired: 2 in, 1 out]
                n1255 = local read "Transfer File"() -> (w2485:path)
                n1256 = Strip Path(path=w2485) -> (stripped path=w2476:path, name=w2494:string)
                n1257 = Unbundle(w2446) -> ("X"=w2444:u32)  [unwired: 1 out]
                n1258 = local write "Transfer Folder"(w2476) -> ()
                n1259 = Bundle("X"=w2444, 0) -> (w2445:cluster{"X":u32, i32})  [unwired: 1 in]
                n1260 = property on="Image Out" class="ImageControl"(error in=w2442, "Image Center Position"=w2445) -> ()  [unwired: 1 in, 2 out]
                n1261 = List Folder(path=w2476) -> (filenames=w2490:string[])  [unwired: 3 in, 3 out]
                n1262 = Search 1D Array(1D array=w2490, element=w2494) -> (index of element=w2487:i32)  [unwired: 1 in]
                n1263 = Array Size(array=w2490) -> (size(s)=w2486:i32)
                n1264 = Decrement(x=w2486) -> (x-1=w2488:i32)
                n1265 = Equal?(x=w2487, y=w2488) -> (x = y?=w2489:bool)
                n1266 = local read "Folder Index"() -> (w2438:dbl)
                n1267 = case shown="False" w2489 {
                  tunnel: w2438 -> [w2619 _]
                  tunnel: [w2618 0] -> w2437
                  frame False {
                    n1268 = Increment(x=w2619) -> (x+1=w2618:dbl)
                  }
                  frame True {
                  }
                }
                n1269 = invoke on="Image Out" class="ImageControl" method="Clear ROI"() -> ()  [unwired: 3 in, 3 out]
                n1270 = local write "Folder Index"(w2437) -> ()
                n1271 = Path To String(path=w2476) -> (string=w2495:string)
                n1272 = Index Array(array=w2490, index=w2437) -> (element=w2491:string)
                n1273 = local write "Data Name:"(w2491) -> ()
                n1274 = Concatenate Strings(w2495, "\\", w2491) -> (w2493:string)
                n1275 = String To Path(string=w2493) -> (path=w2389:path)
                n1276 = call "Recorded Values.vi"("Path"=w2389) -> ("Recorded Char"=w2391:T5, "Recorded Prop"=w2392:T6, "Fabrication Prop"=w2390:T7)  [unwired: 8 in]
                n1277 = Unbundle By Name(w2391) -> ("Mobility-Sat"=w2404:dbl, "Moblitity-Lin"=w2405:dbl, "On/Off"=w2406:dbl, "Off Current"=w2407:dbl, "Vt-Sat"=w2383:dbl, "STS"=w2408:dbl, "Trap Density-VT"=w2409:dbl, "Trap Density-STS"=w2410:dbl)
                n1278 = Unbundle By Name(w2392) -> ("Date Recorded"=w2400:string, "Index"=w2401:string, "Length"=w2402:dbl, "Width"=w2403:dbl, "Sample Temp"=w2386:dbl)
                n1279 = Unbundle By Name(w2390) -> ("Date Created"=w2411:string, "Material"=w2393:string, "Solvent"=w2394:string, "Concentration"=w2395:dbl, "Method"=w2396:string, "Dielectric (nm)"=w2397:dbl, "Treatment"=w2398:string, "Comments"=w2399:string)
                n1280 = local write "Rec: Off I-Sat"(w2407) -> ()
                n1281 = local write "Rec: VT-Sat"(w2383) -> ()
                n1282 = local write "Date Created"(w2411) -> ()
                n1283 = local write "Rec: Material"(w2393) -> ()
                n1284 = local write "Rec: Solvent"(w2394) -> ()
                n1285 = local write "Rec: Concentration"(w2395) -> ()
                n1286 = local write "Rec: Method"(w2396) -> ()
                n1287 = local write "Rec: Dielectric (d)"(w2397) -> ()
                n1288 = local write "Surface Treatment:"(w2398) -> ()
                n1289 = local write "Comments"(w2399) -> ()
                n1290 = local write "Index"(w2401) -> ()
                n1291 = local write "Rec: Mobility-Sat"(w2404) -> ()
                n1292 = local write "Rec: Mobility-Lin"(w2405) -> ()
                n1293 = local write "Rec: On/Off"(w2406) -> ()
                n1294 = local write "Rec: STS"(w2408) -> ()
                n1295 = local write "Rec: Trap Density-VT"(w2409) -> ()
                n1296 = local write "Rec: Trap Density-STS"(w2410) -> ()
                n1297 = local write "Date Recorded"(w2400) -> ()
                n1298 = local write "Rec: Length"(w2402) -> ()
                n1299 = local write "Rec: Width"(w2403) -> ()
                n1300 = local write "Rec: Temp"(w2386) -> ()
                n1301 = Equal To 0?(x=w2386) -> (x = 0?=w2387:bool)
                n1302 = case shown="False" w2387 {
                  tunnel: [w2496 w2497] -> w2384
                  tunnel: w2386 -> [w2496 _]
                  frame False {
                  }
                  frame True {
                    n1303 = local read "Room Temp"() -> (w2497:dbl)
                  }
                }
                n1304 = local write "Transfer File"(w2389) -> ()
                n1305 = local read "NumPts 2"() -> (w2433:dbl)
                n1306 = local read "NumPts"() -> (w2422:dbl)
                n1307 = local read "NumPts"() -> (w2434:dbl)
                n1308 = call-poly <vilib>:"Read From Spreadsheet File.vi"("file path (dialog if empty)"=w2389) -> ("all rows"=w2482:string[][])  [unwired: 6 in, 4 out]
                n1309 = call "Mobility-Vt Calculator-File.vi"("NumPts"=w2434, "Path"=w2389) -> ("XY Graph-Sat"=w2435:cluster{dbl[], dbl[]}[], "XY Graph-Lin"=w2417:cluster{dbl[], dbl[]}[], "Output"=w2436:T8, "Index-Sat"=w2414:dbl, "Index-Lin"=w2421:dbl)  [unwired: 4 in, 1 out]
                n1310 = Decimate 1D Array(w2417) -> (w2429:cluster{dbl[], dbl[]}[])  [unwired: 1 out]
                n1311 = Array To Cluster(array=w2429) -> (cluster=w2427:T9)
                n1312 = Unbundle(w2427) -> ("[0]"=w2428:cluster{dbl[], dbl[]})  [unwired: 8 out]
                n1313 = local write "XY Graph-Lin"(w2417) -> ()
                n1314 = Unbundle(w2428) -> (w2426:dbl[], w2425:dbl[])
                n1315 = Array Subset(array=w2425, index=w2421, length=w2422) -> (w2423:dbl[])
                n1316 = Array Subset(array=w2426, index=w2421, length=w2422) -> (w2424:dbl[])
                n1317 = call "STS Calculator-File.vi"("NumPts"=w2433, "Path"=w2389) -> ("STS Index-Sat"=w2432:dbl, "XY Graph-Sat"=w2431:cluster{dbl[], dbl[]}[], "Ouput"=w2430:cluster{"STS-Sat":dbl, "STS-Lin":dbl})  [unwired: 5 in, 2 out]
                n1318 = local read "New: Dielectric"() -> (w2416:dbl)
                n1319 = local write "Lin Id-Used"(w2423) -> ()
                n1320 = local write "Lin-Vg Array-Used"(w2424) -> ()
                n1321 = local write "MobVi Index"(w2414) -> ()
                n1322 = local write "Slide"(w2414) -> ()
                n1323 = local write "XY Graph"(w2435) -> ()
                n1324 = local write "Index 2"(w2432) -> ()
                n1325 = local write "XY Graph 2"(w2431) -> ()
                n1326 = Unbundle By Name(w2436) -> ("Mobility-Sat"=w2420:dbl, "Vt-Sat"=w2381:dbl, "Mobility-Lin"=w2419:dbl, "Mobility-Lin"=w2418:dbl, "Off I-Sat"=w2412:dbl, "On/Off I-Sat"=w2382:dbl)
                n1327 = Array Size(array=w2482) -> (size(s)=w2481:i32[])
                n1328 = local write "New: Temp"(w2384) -> ()
                n1329 = Unbundle By Name(w2430) -> ("STS-Sat"=w2415:dbl)
                n1330 = call "Trap Density_STS.vi"("Temp (T) [K]"=w2384, "S.T.S. (S)"=w2415, "Dielectric"=w2416) -> ("Trap Density (N)"=w2388:dbl)  [unwired: 8 in]
                n1331 = local write "Calc: Mobility-Lin"(w2419) -> ()
                n1332 = local write "Calc: Mobility-Sat"(w2420) -> ()
                n1333 = local write "Calc: Off I-Sat"(w2412) -> ()
                n1334 = local write "Calc: VT-Sat"(w2381) -> ()
                n1335 = local write "New: VT-Lin"(w2418) -> ()
                n1336 = local write "New: Trap Density-STS"(w2388) -> ()
                n1337 = local write "Calc: Trap Density-STS"(w2388) -> ()
                n1338 = local read "Image Folder"() -> (w2470:path)
                n1339 = local read "New: Dielectric"() -> (w2413:dbl)
                n1340 = Decimate 1D Array(w2435) -> (w2465:cluster{dbl[], dbl[]}[])  [unwired: 1 out]
                n1341 = Decimate 1D Array(w2431) -> (w2455:cluster{dbl[], dbl[]}[])  [unwired: 1 out]
                n1342 = Index Array(array=w2481, index=w2480) -> (element=w2461:i32)
                n1343 = Array Subset(array=w2482, index (row)=w2480, index (col)=w2480, length (col)=3) -> (w2483:string[][])  [unwired: 1 in]
                n1344 = local write "Calc: STS"(w2415) -> ()
                n1345 = local write "New: VT-Sat"(w2381) -> ()
                n1346 = local write "New: Mobility-Sat"(w2420) -> ()
                n1347 = local write "Calc: On/Off"(w2382) -> ()
                n1348 = local write "New: Mobility-Lin"(w2419) -> ()
                n1349 = List Folder(path=w2470) -> (filenames=w2475:string[])  [unwired: 3 in, 3 out]
                n1350 = local write "New: VT-Lin"(w2418) -> ()
                n1351 = Array To Cluster(array=w2465) -> (cluster=w2467:T9)
                n1352 = Array To Cluster(array=w2455) -> (cluster=w2453:T9)
                n1353 = Reshape Array(w2483, w2461) -> (w2468:string[])
                n1354 = Subtract(x=w2461, y=20) -> (x-y=w2460:i32)
                n1355 = local write "New: STS"(w2415) -> ()
                n1356 = property on="Slide" class="Slide (strict)"("Scale.Maximum"=w2460) -> ()  [unwired: 2 in, 2 out]
                n1357 = call "Trap Density_VT.vi"("VT"=w2381, "Dielectric"=w2413) -> ("Trap Density-VT"=w2385:dbl)
                n1358 = Unbundle(w2467) -> ("[0]"=w2466:cluster{dbl[], dbl[]})  [unwired: 8 out]
                n1359 = Unbundle(w2453) -> ("[0]"=w2454:cluster{dbl[], dbl[]})  [unwired: 8 out]
                n1360 = Search 1D Array(1D array=w2468, element="Index:") -> (index of element=w2477:i32)  [unwired: 1 in]
                n1361 = local write "New: Trap Density-VT"(w2385) -> ()
                n1362 = local write "Calc: Trap Density-VT"(w2385) -> ()
                n1363 = Unbundle(w2466) -> (w2457:dbl[], w2456:dbl[])
                n1364 = Unbundle(w2454) -> (w2452:dbl[], w2451:dbl[])
                n1365 = Increment(x=w2477) -> (x+1=w2478:i32)
                n1366 = Array Subset(array=w2457, index=w2414, length=w2434) -> (w2464:dbl[])
                n1367 = Array Subset(array=w2456, index=w2414, length=w2434) -> (w2463:dbl[])
                n1368 = Array Subset(array=w2452, index=w2432, length=w2433) -> (w2459:dbl[])
                n1369 = Array Subset(array=w2451, index=w2432, length=w2433) -> (w2458:dbl[])
                n1370 = Index Array(array=w2468, index=w2478) -> (element=w2473:string)
                n1371 = local write "Vg Array-Log-Used"(w2458) -> ()
                n1372 = local write "Sat Id-Log-Used"(w2459) -> ()
                n1373 = local write "Sat Id-Used"(w2463) -> ()
                n1374 = local write "Index"(w2473) -> ()
                n1375 = local write "Sat Vg Array-Used"(w2464) -> ()
                n1376 = while {
                  tunnel: w2475 -> [w2505]
                  tunnel: w2473 -> [w2503]
                  tunnel: [w2502] -> _
                  tunnel: [w2502] -> w2474
                  tunnel: w2461 -> [w2501]
                  i -> [w2502]
                  stop <- w2498 stop-if-true
                  n1377 = Index Array(array=w2505, index=w2502) -> (element=w2506:string)
                  n1378 = xnode "Match Regular Expression"("input string"=w2506, "regular expression"=w2503) -> ("whole match"=w2504:string)  [unwired: 4 in, 4 out]
                  n1379 = Equal?(x=w2504, y=w2503) -> (x = y?=w2500:bool)
                  n1380 = Equal?(x=w2501, y=w2502) -> (x = y?=w2499:bool)
                  n1381 = Or(x=w2500, y=w2499) -> (x .or. y?=w2498:bool)
                }
                n1382 = Path To String(path=w2470) -> (string=w2472:string)
                n1383 = Index Array(array=w2475, index=w2474) -> (element=w2449:string)
                n1384 = local write "Image Name"(w2449) -> ()
                n1385 = Empty String/Path?(string/path=w2449) -> (empty?=w2450:bool)
                n1386 = Concatenate Strings(w2472, "\\", w2449) -> (w2471:string)
                n1387 = String To Path(string=w2471) -> (path=w2448:path)
                n1388 = local read "No Image File"() -> (w2447:path)
                n1389 = Select(t=w2447, s=w2450, f=w2448) -> (s? t:f=w2441:path)
                n1390 = local write "Image File"(w2441) -> ()
                n1391 = local read "Image Out"() -> (w2439:T2)
                n1392 = call "IMAQ ReadFile"("File Path"=w2441, "Image"=w2439) -> ("Image Out"=w2440:T2)  [unwired: 5 in, 4 out]
                n1393 = local write "Image Out"(w2440) -> ()
                n1394 = local write "Image Out 2"(w2440) -> ()
              }
              frame #4 {
                # "Output ROI data"
                n1395 = local read "Image Folder"() -> (w2621:path)
                n1396 = Build Path(base path=w2621, name or relative path="ROI") -> (appended path=w2623:path)
                n1397 = local read "Index"() -> (w2622:string)
                n1398 = Build Path(base path=w2623, name or relative path=w2622) -> (appended path=w2628:path)
                n1399 = invoke on="Image Out" class="ImageControl" method="Clear ROI"() -> (error out=w2627:errorcluster)  [unwired: 3 in, 2 out]
                n1400 = call <vilib>:"Check if File or Folder Exists.vi"("error in (no error)"=w2627, "path"=w2628) -> ("file or folder exists?"=w2625:bool, "dup path"=w2626:path)  [unwired: 7 in, 1 out]
                n1401 = case shown="True" w2625 {
                  tunnel: w2626 -> [_ w2629]
                  frame False {
                  }
                  frame True {
                    n1402 = Read from Text File(file (use dialog)=w2629) -> (text=w2633:string)  [unwired: 3 in, 3 out]
                    n1403 = property on="Image Out" class="ImageControl"() -> ("ROI"=w2630:T10)  [unwired: 2 in, 2 out]
                    n1404 = Unflatten From String(type=w2630, binary string=w2633) -> (value=w2631:T10, error out=w2632:errorcluster)  [unwired: 3 in, 1 out]
                    n1405 = property on="Image Out" class="ImageControl"(error in=w2632, "ROI"=w2631) -> ()  [unwired: 1 in, 2 out]
                  }
                }
              }
            }
            n1406 = flat-sequence {
              tunnel: [w2076] -> w2063
              tunnel: w2063 -> [w2090]
              frame #0 {
                # "Makes Empty File for Transformer Data"
                n1407 = local read "Transfer Folder"() -> (w2065:path)
                n1408 = Build Path(base path=w2065, name or relative path="Stats") -> (appended path=w2067:path)
                n1409 = call <vilib>:"Check if File or Folder Exists.vi"("path"=w2067) -> ("file or folder exists?"=w2068:bool, "dup path"=w2069:path)  [unwired: 8 in, 1 out]
                n1410 = case shown="False" w2068 {
                  tunnel: [w2073 w2075] -> w2070
                  tunnel: w2069 -> [w2074 w2075]
                  frame False {
                    n1411 = Create Folder(path (use dialog)=w2074) -> (created path=w2073:path)  [unwired: 2 in, 2 out]
                  }
                  frame True {
                  }
                }
                n1412 = Build Path(base path=w2070, name or relative path="Tranformer Data.txt") -> (appended path=w2072:path)
                n1413 = call-poly <vilib>:"Write To Spreadsheet File.vi"("append to file? (new file:F)"=TRUE, "file path (dialog if empty)"=w2072) -> ()  [unwired: 6 in, 1 out]
              }
              frame #1 {
                # "Adds Headers if they don't exist"
                n1414 = local read "Transfer Folder"() -> (w2082:path)
                n1415 = Concatenate Strings("Stats\\", "Tranformer Data.txt") -> (w2083:string)
                n1416 = Build Path(base path=w2082, name or relative path=w2083) -> (appended path=w2076:path)
                n1417 = call-poly <vilib>:"Read From Spreadsheet File.vi"("file path (dialog if empty)"=w2076) -> ("first row"=w2081:string[])  [unwired: 6 in, 4 out]
                n1418 = Search 1D Array(1D array=w2081, element="DeviceID") -> (index of element=w2079:i32)  [unwired: 1 in]
                n1419 = Equal?(x=w2079, y=0) -> (x = y?=w2077:bool)
                n1420 = case shown="False" w2077 {
                  tunnel: w2076 -> [w2087 _]
                  frame False {
                    n1421 = local read "Transformer \nHeaders"() -> (w2086:string[])
                    n1422 = call-poly <vilib>:"Write To Spreadsheet File.vi"("1D data"=w2086, "file path (dialog if empty)"=w2087) -> ()  [unwired: 6 in, 1 out]
                  }
                  frame True {
                  }
                }
              }
              frame #2 {
                # "Adds current device if it doesn't exist"
                n1423 = local read "Current \nRecord"() -> (w2093:string[])
                n1424 = Index Array(array=w2093, index=0) -> (element=w2092:string)
                n1425 = local read "Transfer Folder"() -> (w2095:path)
                n1426 = Concatenate Strings("Stats\\", "Tranformer Data.txt") -> (w2096:string)
                n1427 = local write "Current Device ID"(w2092) -> ()
                n1428 = local read "Current Device ID"() -> (w2102:string)
                n1429 = Build Path(base path=w2095, name or relative path=w2096) -> (appended path=w2094:path)
                n1430 = call-poly <vilib>:"Read From Spreadsheet File.vi"("file path (dialog if empty)"=w2094) -> ("all rows"=w2089:string[][])  [unwired: 6 in, 4 out]
                n1431 = Index Array(array=w2089, index (col)=0) -> (element=w2100:string[])  [unwired: 1 in]
                n1432 = Search 1D Array(1D array=w2100, element=w2102) -> (index of element=w2088:i32)  [unwired: 1 in]
                n1433 = Equal?(x=w2088, y=-1) -> (x = y?=w2091:bool)
                n1434 = case shown="False" w2091 {
                  tunnel: w2090 -> [w2104 w2117]
                  tunnel: w2088 -> [w2109 _]
                  tunnel: w2089 -> [w2110 _]
                  frame False {
                    n1435 = local read "Current \nRecord"() -> (w2108:string[])
                    n1436 = Replace Array Subset(array=w2110, new element=w2108, index (row)=w2109) -> (w2105:string[][])  [unwired: 1 in]
                    n1437 = flat-sequence {
                      tunnel: [w2111] -> _
                      tunnel: [w2112] -> _
                      tunnel: [w2112] -> w2107
                      tunnel: [w2111] -> w2106
                      tunnel: w2105 -> [w2112]
                      tunnel: w2104 -> [w2111]
                      tunnel: w2107 -> [w2114]
                      tunnel: w2106 -> [w2113]
                      frame #0 {
                        n1438 = Delete(path (use dialog)=w2111) -> ()  [unwired: 4 in, 3 out]
                      }
                      frame #1 {
                        n1439 = call-poly <vilib>:"Write To Spreadsheet File.vi"("append to file? (new file:F)"=TRUE, "2D data"=w2114, "file path (dialog if empty)"=w2113) -> ()  [unwired: 5 in, 1 out]
                      }
                    }
                  }
                  frame True {
                    n1440 = local read "Current \nRecord"() -> (w2116:string[])
                    n1441 = call-poly <vilib>:"Write To Spreadsheet File.vi"("append to file? (new file:F)"=TRUE, "1D data"=w2116, "file path (dialog if empty)"=w2117) -> ()  [unwired: 5 in, 1 out]
                  }
                }
              }
            }
          }
          event "Export": Mouse Down {
            n1442 = event-data() -> ()  [unwired: 1 in, 7 out]
            n1443 = flat-sequence {
              frame #0 {
                n1444 = stacked-sequence {
                  frame #0 {
                    n1445 = local read "Independant Variable"() -> (w2635:string)
                    n1446 = Equal?(x=w2635, y="Length (um):") -> (x = y?=w2636:bool)
                    n1447 = case shown="True" w2636 {
                      frame False {
                      }
                      frame True {
                        n1448 = local write "Opj X Axis"("2") -> ()
                      }
                    }
                  }
                  frame #1 {
                    n1449 = local read "Independant Variable"() -> (w2639:string)
                    n1450 = Equal?(x=w2639, y="Sample Temp (K):") -> (x = y?=w2640:bool)
                    n1451 = case shown="True" w2640 {
                      frame False {
                      }
                      frame True {
                        n1452 = local write "Opj X Axis"("1") -> ()
                      }
                    }
                  }
                  frame #2 {
                    n1453 = local read "Independant Variable"() -> (w2643:string)
                    n1454 = Equal?(x=w2643, y="Mobility-Sat (cm^2/Vs):") -> (x = y?=w2644:bool)
                    n1455 = case shown="True" w2644 {
                      frame False {
                      }
                      frame True {
                        n1456 = local write "Opj X Axis"("2") -> ()
                      }
                    }
                  }
                  frame #3 {
                    n1457 = local read "Independant Variable"() -> (w2647:string)
                    n1458 = Equal?(x=w2647, y="Mobility-Lin (cm^2/Vs):") -> (x = y?=w2648:bool)
                    n1459 = case shown="True" w2648 {
                      frame False {
                      }
                      frame True {
                        n1460 = local write "Opj X Axis"("2") -> ()
                      }
                    }
                  }
                  frame #4 {
                    n1461 = local read "Independant Variable"() -> (w2651:string)
                    n1462 = Equal?(x=w2651, y="On/Off I-Sat:") -> (x = y?=w2652:bool)
                    n1463 = case shown="True" w2652 {
                      frame False {
                      }
                      frame True {
                        n1464 = local write "Opj X Axis"("2") -> ()
                      }
                    }
                  }
                  frame #5 {
                    n1465 = local read "Independant Variable"() -> (w2655:string)
                    n1466 = Equal?(x=w2655, y="Off I-Sat (A):") -> (x = y?=w2656:bool)
                    n1467 = case shown="True" w2656 {
                      frame False {
                      }
                      frame True {
                        n1468 = local write "Opj X Axis"("2") -> ()
                      }
                    }
                  }
                  frame #6 {
                    n1469 = local read "Independant Variable"() -> (w2659:string)
                    n1470 = Equal?(x=w2659, y="Vt-Sat (V):") -> (x = y?=w2660:bool)
                    n1471 = case shown="True" w2660 {
                      frame False {
                      }
                      frame True {
                        n1472 = local write "Opj X Axis"("1") -> ()
                      }
                    }
                  }
                  frame #7 {
                    n1473 = local read "Independant Variable"() -> (w2663:string)
                    n1474 = Equal?(x=w2663, y="STS-Sat (V/decade):") -> (x = y?=w2664:bool)
                    n1475 = case shown="True" w2664 {
                      frame False {
                      }
                      frame True {
                        n1476 = local write "Opj X Axis"("1") -> ()
                      }
                    }
                  }
                  frame #8 {
                    n1477 = local read "Independant Variable"() -> (w2667:string)
                    n1478 = Equal?(x=w2667, y="Trap Density-VT (Traps/Vcm^2):") -> (x = y?=w2668:bool)
                    n1479 = case shown="True" w2668 {
                      frame False {
                      }
                      frame True {
                        n1480 = local write "Opj X Axis"("2") -> ()
                      }
                    }
                  }
                  frame #9 {
                    n1481 = local read "Independant Variable"() -> (w2671:string)
                    n1482 = Equal?(x=w2671, y="Trap Density-STS (Traps/Vcm^2):") -> (x = y?=w2672:bool)
                    n1483 = case shown="True" w2672 {
                      frame False {
                      }
                      frame True {
                        n1484 = local write "Opj X Axis"("2") -> ()
                      }
                    }
                  }
                }
              }
              frame #1 {
                n1485 = local read "Transfer Folder"() -> (w2679:path)
                n1486 = Build Path(base path=w2679, name or relative path="Stats") -> (appended path=w2680:path)
                n1487 = local read "Origin Project File"() -> (w2691:path)
                n1488 = call <vilib>:"Check if File or Folder Exists.vi"("path"=w2680) -> ("file or folder exists?"=w2695:bool, "dup path"=w2694:path)  [unwired: 8 in, 1 out]
                n1489 = call <userlib>:"OA_ConnectToOrigin.vi"() -> ("error out"=w2692:errorcluster, "Origin.IOApplication"=w2693:refnum<k7>)  [unwired: 8 in]
                n1490 = case shown="False" w2695 {
                  tunnel: w2694 -> [w2852 w2853]
                  tunnel: [w2851 w2853] -> w2678
                  frame False {
                    n1491 = Create Folder(path (use dialog)=w2852) -> (created path=w2851:path)  [unwired: 2 in, 2 out]
                  }
                  frame True {
                  }
                }
                n1492 = call <userlib>:"OA_Load.vi"("error in (no error)"=w2692, "Path"=w2691, "Origin.IOApplication"=w2693) -> ("error out"=w2689:errorcluster, "Origin.IOApplication"=w2690:refnum<k7>)  [unwired: 1 out]
                n1493 = call <userlib>:"OAExecute.vi"("script"="document -m 3;", "Error IO"=w2689, "Origin.IOApplication"=w2690) -> ("Error IO Out"=w2687:errorcluster, "Origin.IOApplication"=w2688:refnum<k7>)  [unwired: 1 in, 1 out]
                n1494 = call "File Dialog"("start path"=w2680) -> ("selected path"=w2682:path)  [unwired: 11 in, 3 out]
                n1495 = local read "Independant Variable"() -> (w2675:string)
                n1496 = stacked-sequence {
                  tunnel: w2679 -> [w2704 w2732 w2742 w2762 w2780 w2799 w2818 w2839]
                  tunnel: w2678 -> [w2705 w2731 w2743 w2761 w2781 w2800 w2819 w2840]
                  tunnel: w2688 -> [w2707 w2729 w2745 w2764 w2783 w2802 w2821 w2842]
                  tunnel: w2687 -> [w2706 w2730 w2744 w2763 w2782 w2801 w2820 w2841]
                  tunnel: [_ _ _ _ _ _ _ w2837] -> w2677
                  tunnel: [_ _ _ _ _ _ _ w2838] -> w2676
                  tunnel: w2675 -> [w2703 w2722 w2741 w2760 w2779 w2798 w2817 w2836]
                  frame #0 {
                    n1497 = local read "Opj X Axis"() -> (w2699:string)
                    n1498 = Concatenate Strings("window -a MOBLGraph;\nlayer.x.type=", w2699, ";", "window -a MOBLTable;\nwindow -s TV;") -> (w2697:string)
                    n1499 = call "Param_Analysis_7_24b_JW.vi"("Independant Variable"=w2703, "error in (no error)"=w2706, "Data Folder"=w2704, "Parameter String"="Mobility-Lin (cm^2/Vs):", "Parameter Name"="Mobility-Lin", "Stats Folder"=w2705) -> ("error out"=w2709:errorcluster, "Output Array"=w2711:string[][], "Variables"=w2702:T16)  [unwired: 2 in, 1 out]
                    n1500 = call "Origin_Export_7_27a_JW.vi"("Input Conditions"=w2702, "Analysis Array"=w2711, "error in (no error)"=w2709, "Parameter Worksheet Name"="[MOBLTable]Mobilities", "Parameter Folder Script"="pe_cd \"Mobility-Lin\";", "Origin.IOApplication"=w2707) -> ("error out"=w2708:errorcluster, "reference out"=w2710:refnum<k7>)  [unwired: 3 in, 1 out]
                    n1501 = call <userlib>:"OAExecute.vi"("script"=w2697, "Error IO"=w2708, "Origin.IOApplication"=w2710) -> ()  [unwired: 1 in, 3 out]
                  }
                  frame #1 {
                    n1502 = local read "Opj X Axis"() -> (w2718:string)
                    n1503 = Concatenate Strings("window -a MOBSGraph;\nlayer.x.type=", w2718, ";", "window -a MOBSTable;\nwindow -s TV;") -> (w2716:string)
                    n1504 = call "Param_Analysis_7_24b_JW.vi"("Independant Variable"=w2722, "error in (no error)"=w2730, "Data Folder"=w2732, "Parameter String"="Mobility-Sat (cm^2/Vs):", "Parameter Name"="Mobility-Sat", "Stats Folder"=w2731) -> ("error out"=w2725:errorcluster, "Output Array"=w2723:string[][], "Variables"=w2721:T16)  [unwired: 2 in, 1 out]
                    n1505 = call "Origin_Export_7_27a_JW.vi"("Input Conditions"=w2721, "Analysis Array"=w2723, "error in (no error)"=w2725, "Parameter Worksheet Name"="[MOBSTable]Mobilities", "Parameter Folder Script"="pe_cd \"Mobility-Sat\";", "Origin.IOApplication"=w2729) -> ("error out"=w2724:errorcluster, "reference out"=w2726:refnum<k7>)  [unwired: 3 in, 1 out]
                    n1506 = call <userlib>:"OAExecute.vi"("script"=w2716, "Error IO"=w2724, "Origin.IOApplication"=w2726) -> ()  [unwired: 1 in, 3 out]
                  }
                  frame #2 {
                    n1507 = local read "Opj X Axis"() -> (w2737:string)
                    n1508 = Concatenate Strings("window -a NSTSGraph;\nlayer.x.type=", w2737, ";", "window -a NSTSTable;\nwindow -s TV;") -> (w2735:string)
                    n1509 = call "Param_Analysis_7_24b_JW.vi"("Independant Variable"=w2741, "error in (no error)"=w2744, "Data Folder"=w2742, "Parameter String"="Trap Density-STS (Traps/Vcm^2):", "Parameter Name"="Trap Density-STS", "Stats Folder"=w2743) -> ("error out"=w2748:errorcluster, "Output Array"=w2746:string[][], "Variables"=w2740:T16)  [unwired: 2 in, 1 out]
                    n1510 = call "Origin_Export_7_27a_JW.vi"("Input Conditions"=w2740, "Analysis Array"=w2746, "error in (no error)"=w2748, "Parameter Worksheet Name"="[NSTSTable]Trap Densities", "Parameter Folder Script"="pe_cd \"N-STS\";", "Origin.IOApplication"=w2745) -> ("error out"=w2747:errorcluster, "reference out"=w2749:refnum<k7>)  [unwired: 3 in, 1 out]
                    n1511 = call <userlib>:"OAExecute.vi"("script"=w2735, "Error IO"=w2747, "Origin.IOApplication"=w2749) -> ()  [unwired: 1 in, 3 out]
                  }
                  frame #3 {
                    n1512 = local read "Opj X Axis"() -> (w2756:string)
                    n1513 = call "Param_Analysis_7_24b_JW.vi"("Independant Variable"=w2760, "error in (no error)"=w2763, "Data Folder"=w2762, "Parameter String"="Trap Density-VT (Traps/Vcm^2):", "Parameter Name"="Trap Density-Vt", "Stats Folder"=w2761) -> ("error out"=w2767:errorcluster, "Output Array"=w2765:string[][], "Variables"=w2759:T16)  [unwired: 2 in, 1 out]
                    n1514 = Concatenate Strings("window -a NVtGraph;\nlayer.x.type=", w2756, ";", "window -a NVtTable;\nwindow -s TV;") -> (w2754:string)
                    n1515 = call "Origin_Export_7_27a_JW.vi"("Input Conditions"=w2759, "Analysis Array"=w2765, "error in (no error)"=w2767, "Parameter Worksheet Name"="[NVTTable]Trap Densities", "Parameter Folder Script"="pe_cd \"N-Vt\";", "Origin.IOApplication"=w2764) -> ("error out"=w2766:errorcluster, "reference out"=w2768:refnum<k7>)  [unwired: 3 in, 1 out]
                    n1516 = call <userlib>:"OAExecute.vi"("script"=w2754, "Error IO"=w2766, "Origin.IOApplication"=w2768) -> ()  [unwired: 1 in, 3 out]
                  }
                  frame #4 {
                    n1517 = local read "Opj X Axis"() -> (w2775:string)
                    n1518 = Concatenate Strings("window -a OffIGraph;\nlayer.x.type=", w2775, ";", "window -a OffITable;\nwindow -s TV;") -> (w2773:string)
                    n1519 = call "Param_Analysis_7_24b_JW.vi"("Independant Variable"=w2779, "error in (no error)"=w2782, "Data Folder"=w2780, "Parameter String"="Off I-Sat (A):", "Parameter Name"="Off I-Sat", "Stats Folder"=w2781) -> ("error out"=w2786:errorcluster, "Output Array"=w2784:string[][], "Variables"=w2778:T16)  [unwired: 2 in, 1 out]
                    n1520 = call "Origin_Export_7_27a_JW.vi"("Input Conditions"=w2778, "Analysis Array"=w2784, "error in (no error)"=w2786, "Parameter Worksheet Name"="[OffItable]OffCurrents", "Parameter Folder Script"="pe_cd \"OffI-Sat\";", "Origin.IOApplication"=w2783) -> ("error out"=w2785:errorcluster, "reference out"=w2787:refnum<k7>)  [unwired: 3 in, 1 out]
                    n1521 = call <userlib>:"OAExecute.vi"("script"=w2773, "Error IO"=w2785, "Origin.IOApplication"=w2787) -> ()  [unwired: 1 in, 3 out]
                  }
                  frame #5 {
                    n1522 = local read "Opj X Axis"() -> (w2794:string)
                    n1523 = Concatenate Strings("window -a OnOffGraph;\nlayer.x.type=", w2794, ";", "window -a OnOffTable;\nwindow -s TV;") -> (w2792:string)
                    n1524 = call "Param_Analysis_7_24b_JW.vi"("Independant Variable"=w2798, "error in (no error)"=w2801, "Data Folder"=w2799, "Parameter String"="On/Off I-Sat:", "Parameter Name"="OnOff Ratio", "Stats Folder"=w2800) -> ("error out"=w2805:errorcluster, "Output Array"=w2803:string[][], "Variables"=w2797:T16)  [unwired: 2 in, 1 out]
                    n1525 = call "Origin_Export_7_27a_JW.vi"("Input Conditions"=w2797, "Analysis Array"=w2803, "error in (no error)"=w2805, "Parameter Worksheet Name"="[OnOffTable]On/Off Ratios", "Parameter Folder Script"="pe_cd \"OnOff-Ratio\";", "Origin.IOApplication"=w2802) -> ("error out"=w2804:errorcluster, "reference out"=w2806:refnum<k7>)  [unwired: 3 in, 1 out]
                    n1526 = call <userlib>:"OAExecute.vi"("script"=w2792, "Error IO"=w2804, "Origin.IOApplication"=w2806) -> ()  [unwired: 1 in, 3 out]
                  }
                  frame #6 {
                    n1527 = local read "Opj X Axis"() -> (w2813:string)
                    n1528 = call "Param_Analysis_7_24b_JW.vi"("Independant Variable"=w2817, "error in (no error)"=w2820, "Data Folder"=w2818, "Parameter String"="STS-Sat (V/decade):", "Parameter Name"="STS-Sat", "Stats Folder"=w2819) -> ("error out"=w2824:errorcluster, "Output Array"=w2822:string[][], "Variables"=w2816:T16)  [unwired: 2 in, 1 out]
                    n1529 = Concatenate Strings("window -a SGraph;\nlayer.x.type=", w2813, ";", "window -a STable;\nwindow -s TV;") -> (w2811:string)
                    n1530 = call "Origin_Export_7_27a_JW.vi"("Input Conditions"=w2816, "Analysis Array"=w2822, "error in (no error)"=w2824, "Parameter Worksheet Name"="[STable]Threshold Swing", "Parameter Folder Script"="pe_cd \"STS-Sat\";", "Origin.IOApplication"=w2821) -> ("error out"=w2823:errorcluster, "reference out"=w2825:refnum<k7>)  [unwired: 3 in, 1 out]
                    n1531 = call <userlib>:"OAExecute.vi"("script"=w2811, "Error IO"=w2823, "Origin.IOApplication"=w2825) -> ()  [unwired: 1 in, 3 out]
                  }
                  frame #7 {
                    n1532 = local read "Opj X Axis"() -> (w2832:string)
                    n1533 = Concatenate Strings("window -a VtGraph;\nlayer.x.type=", w2832, ";", "window -a VtTable;\nwindow -s TV;") -> (w2830:string)
                    n1534 = call "Param_Analysis_7_24b_JW.vi"("Independant Variable"=w2836, "error in (no error)"=w2841, "Data Folder"=w2839, "Parameter String"="Vt-Sat (V):", "Parameter Name"="Vt-Sat", "Stats Folder"=w2840) -> ("error out"=w2845:errorcluster, "Output Array"=w2843:string[][], "Variables"=w2835:T16)  [unwired: 2 in, 1 out]
                    n1535 = call "Origin_Export_7_27a_JW.vi"("Input Conditions"=w2835, "Analysis Array"=w2843, "error in (no error)"=w2845, "Parameter Worksheet Name"="[VtTable]Threshold Voltages", "Parameter Folder Script"="pe_cd \"Vt-Sat\";", "Origin.IOApplication"=w2842) -> ("error out"=w2844:errorcluster, "reference out"=w2846:refnum<k7>)  [unwired: 3 in, 1 out]
                    n1536 = call <userlib>:"OAExecute.vi"("script"=w2830, "Error IO"=w2844, "Origin.IOApplication"=w2846) -> ("Error IO Out"=w2837:errorcluster, "Origin.IOApplication"=w2838:refnum<k7>)  [unwired: 1 in, 1 out]
                  }
                }
                n1537 = Path To String(path=w2682) -> (string=w2681:string)
                n1538 = call <userlib>:"OAExecute.vi"("script"="pe_cd /; ", "Error IO"=w2677, "Origin.IOApplication"=w2676) -> ("Error IO Out"=w2683:errorcluster, "Origin.IOApplication"=w2684:refnum<k7>)  [unwired: 1 in, 1 out]
                n1539 = call <userlib>:"OASaveProject.vi"("path"=w2681, "Error IO"=w2683, "Origin.IOApplication"=w2684) -> ()  [unwired: 3 out]
              }
            }
          }
          event "Blank Button": Mouse Down {
            n1540 = event-data() -> ()  [unwired: 1 in, 7 out]
            n1541 = local read "Transfer File"() -> (w2861:path)
            n1542 = disable-structure shown="Disabled" {
              frame Disabled {
                n1543 = local read "Folder Index"() -> (w2862:dbl)
                n1544 = Decrement(x=w2862) -> (x-1=w2863:dbl)
                n1545 = local write "Folder Index"(w2863) -> ()
              }
              frame Enabled {
              }
            }
            n1546 = Strip Path(path=w2861) -> (stripped path=w2857:path, name=w2859:string)
            n1547 = Path To String(path=w2857) -> (string=w2856:string)
            n1548 = Concatenate Strings(w2856, "\\", "X_", w2859) -> (w2855:string)
            n1549 = String To Path(string=w2855) -> (path=w2854:path)
            n1550 = Move(source path=w2861, 10:w2854) -> ()  [unwired: 3 in, 3 out]
            n1551 = local write "Transfer File"(w2854) -> ()
          }
          event "Cancel Button": Mouse Down {
            (unwired) 6
            n1552 = event-data() -> ()  [unwired: 1 in, 7 out]
            n1553 = call "Simulate_Keyboard.vi"("Action"=2, "Virtual Key"=162) -> ()  [unwired: 7 in, 1 out]
          }
        }
        n1554 = Multiply(x=w525, y=10) -> (x*y=w527:sgl)
        n1555 = case shown="\"0\"" w566 {
          tunnel: w540 -> [w620 w626 w630 w632 w636 w638 w640 w642 w644 w646 w648 w650 w652 w654 w656 w658 w660 w662 w664 w666 w668 w670 w672 w674 w676 w678 w680 w682 w684 w686 w688 w690 w692 w694 w696 w698 w700 w702 w704 w706 w708 w710 w712 w714 w716 w718 w720 w722 w724 w726 w728 w730 w732 w734 w736 w738 w740 w742 w744 w746 w748 w750 w752 w754 w756 w758 w760 w762 w764 w766 w768 w770 w772 w774 w776 w778 w780 w782 w784 w786 w788 w790 w792 w794 w796 w798 w800 w802 w804 w806 w808 w810 w812 w814 w816 w818 w820 w822 w824 w826 w828 w830 w832 w834 w836]
          tunnel: [w620 w625 w629 w632 w636 w638 w640 w642 w644 w646 w648 w650 w652 w654 w656 w658 w660 w662 w664 w666 w668 w670 w672 w674 w676 w678 w680 w682 w684 w686 w688 w690 w692 w694 w696 w698 w700 w702 w704 w706 w708 w710 w712 w714 w716 w718 w720 w722 w724 w726 w728 w730 w732 w734 w736 w738 w740 w742 w744 w746 w748 w750 w752 w754 w756 w758 w760 w762 w764 w766 w768 w770 w772 w774 w776 w778 w780 w782 w784 w786 w788 w790 w792 w794 w796 w798 w800 w802 w804 w806 w808 w810 w812 w814 w816 w818 w820 w822 w824 w826 w828 w830 w832 w834 w836] -> w565
          tunnel: w541 -> [w622 w624 w628 w634 w635 w637 w639 w641 w643 w645 w647 w649 w651 w653 w655 w657 w659 w661 w663 w665 w667 w669 w671 w673 w675 w677 w679 w681 w683 w685 w687 w689 w691 w693 w695 w697 w699 w701 w703 w705 w707 w709 w711 w713 w715 w717 w719 w721 w723 w725 w727 w729 w731 w733 w735 w737 w739 w741 w743 w745 w747 w749 w751 w753 w755 w757 w759 w761 w763 w765 w767 w769 w771 w773 w775 w777 w779 w781 w783 w785 w787 w789 w791 w793 w795 w797 w799 w801 w803 w805 w807 w809 w811 w813 w815 w817 w819 w821 w823 w825 w827 w829 w831 w833 w835]
          tunnel: [w621 w624 w628 w633 w635 w637 w639 w641 w643 w645 w647 w649 w651 w653 w655 w657 w659 w661 w663 w665 w667 w669 w671 w673 w675 w677 w679 w681 w683 w685 w687 w689 w691 w693 w695 w697 w699 w701 w703 w705 w707 w709 w711 w713 w715 w717 w719 w721 w723 w725 w727 w729 w731 w733 w735 w737 w739 w741 w743 w745 w747 w749 w751 w753 w755 w757 w759 w761 w763 w765 w767 w769 w771 w773 w775 w777 w779 w781 w783 w785 w787 w789 w791 w793 w795 w797 w799 w801 w803 w805 w807 w809 w811 w813 w815 w817 w819 w821 w823 w825 w827 w829 w831 w833 w835] -> w564
          tunnel: w527 -> [w619 w623 w627 w631 _ _ _ _ _ _ _ _ _ _ _ _ _ _ _ _ _ _ _ _ _ _ _ _ _ _ _ _ _ _ _ _ _ _ _ _ _ _ _ _ _ _ _ _ _ _ _ _ _ _ _ _ _ _ _ _ _ _ _ _ _ _ _ _ _ _ _ _ _ _ _ _ _ _ _ _ _ _ _ _ _ _ _ _ _ _ _ _ _ _ _ _ _ _ _ _ _ _ _ _ _]
          frame "DOWN" {
            n1556 = Add(x=w622, y=w619) -> (x+y=w621:sgl)
          }
          frame "LEFT" {
            n1557 = Subtract(x=w626, y=w623) -> (x-y=w625:sgl)
          }
          frame "RIGHT" {
            n1558 = Add(x=w630, y=w627) -> (x+y=w629:sgl)
          }
          frame "UP" {
            n1559 = Subtract(x=w634, y=w631) -> (x-y=w633:sgl)
          }
          frame "ENTER (num pad)" {
          }
          frame "' (quote)" {
          }
          frame "END" {
          }
          frame "EQUALS" {
          }
          frame "ESCAPE" {
          }
          frame "GRAVE (`)" {
          }
          frame "HOME" {
          }
          frame "INSERT" {
          }
          frame "LBRACKET" {
          }
          frame "LCONTROL" {
          }
          frame "L ALT" {
          }
          frame "LSHIFT" {
          }
          frame "LWIN" {
          }
          frame "MINUS" {
          }
          frame "MULTIPLY" {
          }
          frame "NEXT" {
          }
          frame "NUMLOCK" {
          }
          frame "NUMPAD_0" {
          }
          frame "NUMPAD_1" {
          }
          frame "NUMPAD_2" {
          }
          frame "NUMPAD_3" {
          }
          frame "NUMPAD_4" {
          }
          frame "NUMPAD_5" {
          }
          frame "NUMPAD_6" {
          }
          frame "NUMPAD_7" {
          }
          frame "NUMPAD_8" {
          }
          frame "NUMPAD_9" {
          }
          frame "PAUSE" {
          }
          frame "PERIOD" {
          }
          frame "PRIOR (PG UP)" {
          }
          frame "RBRACKET" {
          }
          frame "RCONTROL" {
          }
          frame "RETURN" {
          }
          frame "R ALT" {
          }
          frame "RSHIFT" {
          }
          frame "RWIN" {
          }
          frame "SCROLL" {
          }
          frame "SEMICOLON" {
          }
          frame "SLASH" {
          }
          frame "SPACE" {
          }
          frame "SUBTRACT" {
          }
          frame "TAB" {
          }
          frame "DIVIDE" {
          }
          frame "DELETE" {
          }
          frame "DECIMAL" {
          }
          frame "COMMA" {
          }
          frame "CAPITAL" {
          }
          frame "BACKSLASH" {
          }
          frame "BACK" {
          }
          frame "ADD" {
          }
          frame "F15" {
          }
          frame "F14" {
          }
          frame "F13" {
          }
          frame "F12" {
          }
          frame "F11" {
          }
          frame "F10" {
          }
          frame "F9" {
          }
          frame "F8" {
          }
          frame "F7" {
          }
          frame "F6" {
          }
          frame "F5" {
          }
          frame "F4" {
          }
          frame "F3" {
          }
          frame "F2" {
          }
          frame "F1" {
          }
          frame "Z" {
          }
          frame "Y" {
          }
          frame "X" {
          }
          frame "W" {
          }
          frame "V" {
          }
          frame "U" {
          }
          frame "T" {
          }
          frame "S" {
          }
          frame "R" {
          }
          frame "Q" {
          }
          frame "P" {
          }
          frame "O" {
          }
          frame "N" {
          }
          frame "M" {
          }
          frame "L" {
          }
          frame "K" {
          }
          frame "J" {
          }
          frame "I" {
          }
          frame "H" {
          }
          frame "G" {
          }
          frame "F" {
          }
          frame "E" {
          }
          frame "D" {
          }
          frame "C" {
          }
          frame "B" {
          }
          frame "A" {
          }
          frame "9" {
          }
          frame "8" {
          }
          frame "7" {
          }
          frame "6" {
          }
          frame "5" {
          }
          frame "4" {
          }
          frame "3" {
          }
          frame "2" {
          }
          frame "1" {
          }
          frame "0" {
          }
        }
        n1560 = Bundle(w543, w542, w557, w556, 0.0) -> (w555:cluster{dbl, dbl, dbl, dbl, dbl})  [unwired: 1 in]
        n1561 = Bundle("X"=w565, "Y"=w564) -> (w559:cluster{"X":sgl, "Y":sgl})  [unwired: 1 in]
        n1562 = Divide(x=20, y=w526) -> (x/y=w529:sgl)
        n1563 = property on="Image Out" class="ImageControl"("Image Center Position"=w559) -> ()  [unwired: 2 in, 2 out]
        n1564 = call "IMAQ Convert Rectangle to ROI (Polygon)"("Rectangle"=w555) -> ("ROI Descriptor"=w553:T3)  [unwired: 7 in, 2 out]
        n1565 = Bundle("Application Font", w529, w533, w533, w533, w533, w533, TRUE, w531) -> (w535:T17)  [unwired: 1 in]
        n1566 = property on="Image Out 2" class="ImageControl"("ROI"=w553) -> ()  [unwired: 2 in, 2 out]
        n1567 = Bundle(w531, w535, w531, w531) -> (w534:T18)  [unwired: 1 in]
        n1568 = property on="Image Out" class="ImageControl"() -> ("ROI"=w518:T10)  [unwired: 2 in, 2 out]
        n1569 = Unbundle By Name(w518) -> ("Contours"=w582:T14)
        n1570 = local read "Image Out"() -> (w537:T2)
        n1571 = call "IMAQ Clear Overlay"("Image"=w537) -> ("Image Out"=w536:T2)  [unwired: 9 in, 1 out]
        n1572 = Initialize Array(0) -> (w580:i32[])  [unwired: 1 in]
        n1573 = local read "Magnification"() -> (w571:u16)
        n1574 = Array Size(array=w582) -> (size(s)=w581:i32)
        n1575 = Build Array(0.505025, 0.252522, 0.127742, 0.050345, 0.031129) -> (w572:dbl[])
        n1576 = Array Subset(array=w572, index=w571, length=1) -> (w569:dbl[])
        n1577 = property on="Image Out" class="ImageControl"() -> ("ZoomInteger"=w561:cluster{"X":i32, "Y":i32})  [unwired: 2 in, 2 out]
        n1578 = To Double Precision Float(number=w569) -> (double precision float=w568:dbl[])
        n1579 = for {
          N: w581 -> [_]
          shift-right: [w859] -> _
          shift-left: w582 -> [w859]
          shift-right: [w857] -> w567
          shift-left: w580 -> [w856]
          tunnel: w568 -> [w855]
          shift-right: [w852] -> _
          shift-left: w536 -> [w854]
          tunnel: w534 -> [w847]
          i -> [w851]
          n1580 = Index Array(array=w859, index=w851) -> (element=w868:T19)
          n1581 = Unbundle(w868) -> ("Points"=w867:i32[])  [unwired: 2 out]
          n1582 = Array To Cluster(array=w867) -> (cluster=w866:T20)
          n1583 = Unbundle(w866) -> ("Points[0]"=w846:i32, "Points[1]"=w843:i32, "Points[2]"=w858:i32, "Points[3]"=w864:i32)  [unwired: 5 out]
          n1584 = Add(x=w846, y=10) -> (x+y=w844:i32)
          n1585 = Subtract(x=w843, y=w864) -> (x-y=w863:i32)
          n1586 = Subtract(x=w846, y=w858) -> (x-y=w865:i32)
          n1587 = Square(x=w863) -> (x^2=w861:i32)
          n1588 = Square(x=w865) -> (x^2=w862:i32)
          n1589 = Add(x=w862, y=w861) -> (x+y=w860:i32)
          n1590 = Square Root(x=w860) -> (sqrt(x)=w837:dbl)
          n1591 = Multiply(x=w837, y=0.5) -> (x*y=w840:dbl)
          n1592 = Add(x=w840, y=w843) -> (x+y=w842:dbl)
          n1593 = Bundle(w844, w842) -> (w853:cluster{i32, dbl})  [unwired: 1 in]
          n1594 = Multiply(x=w837, y=w855) -> (x*y=w850:dbl[])
          n1595 = Index Array(array=w850) -> (element=w849:dbl)  [unwired: 1 in]
          n1596 = Number To Fractional String(number=w849) -> (F-format string=w848:string)  [unwired: 3 in]
          n1597 = call "IMAQ Overlay Text"("BG Color (Transparent)"=u32 0, "Text Color (black)"=u32 16448250, "Font, Size & Style"=w847, "String"=w848, "Origin"=w853, "Image"=w854) -> ("Image Out"=w852:T2)  [unwired: 4 in, 1 out]
          n1598 = Build Array (concatenate)(w856, w850) -> (w857:dbl[])
          n1599 = local write "Numeric 3"(w837) -> ()
        }
        n1600 = local write "ROI Descriptor"(w518) -> ()
        n1601 = Unbundle(w561) -> ("X"=w560:i32)  [unwired: 1 out]
        n1602 = Add Array Elements(numeric array=w567) -> (sum=w578:dbl)
        n1603 = local write "Distances"(w567) -> ()
        n1604 = local write "Total Width"(w578) -> ()
        n1605 = local write "Zoom"(w560) -> ()
        n1606 = local read "Manual-Width"() -> (w517:bool)
        n1607 = local read "Total Width"() -> (w521:dbl)
        n1608 = local read "Rec: Width"() -> (w519:dbl)
        n1609 = Not(x=w517) -> (.not. x?=w515:bool)
        n1610 = Equal To 0?(x=w521) -> (x = 0?=w516:bool)
        n1611 = Or(x=w516, y=w517) -> (x .or. y?=w520:bool)
        n1612 = And(x=w516, y=w515) -> (x .and. y?=w514:bool)
        n1613 = case shown="True" w514 {
          tunnel: w519 -> [_ w597]
          frame False {
          }
          frame True {
            n1614 = local write "New: Width"(w597) -> ()
          }
        }
        n1615 = case shown="False" w520 {
          tunnel: w521 -> [w598 _]
          frame False {
            n1616 = local write "New: Width"(w598) -> ()
          }
          frame True {
          }
        }
        n1617 = local read "Manuel-Dielectric"() -> (w443:bool)
        n1618 = local read "Rec: Dielectric (d)"() -> (w442:dbl)
        n1619 = local read "Manuel-Length"() -> (w444:bool)
        n1620 = local read "Manual-Temp"() -> (w416:bool)
        n1621 = local read "Rec: Length"() -> (w445:dbl)
        n1622 = local read "Rec: Temp"() -> (w417:dbl)
        n1623 = case shown="False" w444 {
          tunnel: w445 -> [w588 _]
          frame False {
            n1624 = local write "New: Length"(w588) -> ()
          }
          frame True {
          }
        }
        n1625 = case shown="False" w443 {
          tunnel: w442 -> [w587 _]
          frame False {
            n1626 = local write "New: Dielectric"(w587) -> ()
          }
          frame True {
          }
        }
        n1627 = case shown="False" w416 {
          tunnel: w417 -> [w584 _]
          frame False {
            n1628 = local write "New: Temp"(w584) -> ()
          }
          frame True {
          }
        }
      }
    }
  }
  n1629 = Build Array("DeviceID", "Fabricator", "Deposition", "Date", "Sample", "Row", "Column", "L (um)", "W (um)", "Material", "Treatment", "TC (mM)", "Solvent", "C (%)", "ST (C)", "Drops", "Wait (s)", "RT (F)", "RH (%)", "Ramp (s)", "RPM", "Accel (RPM/s)", "Time (s)", "Mobility", "On/Off", "Vt", "S.T.S") -> (→"Transformer \nHeaders":string[])
